vi "多点监测上位机.vi"() -> ()   [LabVIEW 2017]
uses:
  <vilib>/Utility/miscctls.llb/LVRowAndColumnTypeDef.ctl
  <vilib>/Utility/miscctls.llb/LVRowAndColumnUnsignedTypeDef.ctl
  <vilib>/Platform/TimedLoop/XDataNode/timing_clust.ctl
  <vilib>/Platform/TimedLoop/XDataNode/nitl_modes.ctl
  <vilib>/Platform/TimedLoop/XDataNode/wakeup.ctl
  <vilib>/event_ctls.llb/eventvkey.ctl
  <vilib>/Utility/xml.llb/Read From XML File(string).vi
  <vilib>/sound2/lvsound2.llb/Sound File Info (path).vi
  <vilib>/sound2/lvsound2.llb/Sound File Read Open.vi
  <vilib>/sound2/lvsound2.llb/Sound File Read (DBL).vi
  <vilib>/Instr/_visa.llb/VISA Configure Serial Port (Instr).vi
  <vilib>/Utility/inputDevices.llb/closeMouse.vi
  <vilib>/Utility/xml.llb/Write to XML File(string).vi
  <vilib>/Utility/inputDevices.llb/mouseAcquire.vi
  <vilib>/Platform/TimedLoop/XDataNode/XDataNode.xnode
  <vilib>/Platform/TimedLoop/XDataNode/XDNodeRunTimeDep.lvlib
  <vilib>/addons/database/NI_Database_API.lvlib
panel:
  out "标志-首次累积报警":bool=TRUE
  out "信号-保存配置":bool=TRUE
  out "手动静音窗口VI-引用":refnum<vi>
  in  "报警方式":T1(array[cluster])
  in  "轮询间隔 ms":dbl
  in  "一周期间隔":timestamp
  in  "周期":i64
  in  "有掉线？":bool
  out "事件-累积剂量":refnum<user-event>
  in  "报警状态":enum16{"正常", "一级报警", "二级报警", "累积报警"}[](array[ring])
  in  "累积剂量":T2(array[cluster])
  out "监测数量限值":cluster{"min":i32, "max":i32}
  out "监-停止信号":refnum<vi>
  in  "报警列表提示":string[](array[string])=["选行技巧：按住 ctl 可离散选择，按住 shift 可范围选择，ctl+A 选择全部行", "右键菜单：多选后 某些项可批量操作", "双击“单元格”：打开报警记录数据分析界面，可编辑结论、生成Word报表", "底端“状态栏”：可调整状态栏高度、分类筛选、清除状态"]
  in  "设备列表提示":string[](array[string])=["选行技巧：按住 ctl 可离散选择，按住 shift 可范围选择，ctl+A 选择全部行", "右键菜单：多选后 某些项可批量操作", "双击“状态”列：启用或禁用设备（某些版本中禁用此功能）", "双击“设备信息”列：修改设备信息", "双击“一级限值”列：修改报警限值", "双击“网络地址”列：删除设备", "双击“空白行”：添加设备"]
  in  "停止信号":enum16{"内部停止信号", "外部停止信号"}(ring)=enum."外部停止信号"
  out "事件-探头重连":refnum<user-event>
  out "报警记录数":i32
  out "通知窗口VI-引用":refnum<vi>
  in  "新记录簇":cluster{"新记录列表行":string[], "对应缓存文件":string}[](array[cluster])
  in  "报警状态":enum16{"正常", "一级报警", "二级报警", "累积报警"}(ring)
  out "蜂鸣音效":waveform(dbl)[](array[waveform]) caption="数据"
  in  "Right":i16
  in  "Left":i16
  out "间隔":u32
  in  "计时":u32
  out "引用-更新数据信号":refnum<vi>
  out "引用-更新数据簇":refnum<vi>
  in  "信号-设置":bool
  in  "菜单项-报警列表":enum16{"刷新", "预览并生成报表", "删除记录", "复制选中项至剪贴板"}(ring)=enum."预览并生成报表"
  in  "菜单项-实时列表":T3(ring)=enum."禁用"
  out "监测窗口VI":refnum<vi>
  out "报警记录缓存数据文件":string[](array[string])
  in  "缓存值":cluster{"X":timestamp[], "Y":dbl[]}[](array[cluster])
  in  "状态栏-项名[]":string[](array[string])
  in  "状态与编辑":bool
  in  "监测模式":bool caption="方格样式"
  in  "查看报表":bool caption="方格样式"
  in  "设置":bool
  in  "帮助":bool
  out "公司LOGO与型号":bool
  out "设备列表标题":enum16{"设备管理列表"}(ring)
  out "当前端口":string
  out "当前波特率":string
  out "设备列表操作提示":string
  in  "限值":T4(array[cluster])
  in  "实时数据列表":i32[](listbox)
  out "报警列表标题":enum16{"报警记录列表"}(ring)
  out "报警列表操作提示":string
  in  "T:G,F:B":bool
  in  "回复背景色锁":bool
  in  "等待时间（毫秒）":u32=10
  in  "暂停发送":bool=TRUE
  in  "报警记录列表":i32[](listbox)
  in  "状态类型":enum16{"全部", "报警", "通信", "设置"}(ring)
  in  "报警方式变了？":bool
  in  "限值变了？":bool
  in  "状态栏":i32(listbox)=-1
  out "事件-探头掉线":refnum<user-event>
  out "事件-报警缓存":refnum<user-event>
  out "测量值":cluster{"X":timestamp, "Y":dbl}[](array[cluster])
  in  "开机启动":bool
  in  "device ID":refnum<k1> caption="设备ID"
  in  "变了？":bool
  in  "发送次数":u8[](array[numeric])
  in  "异常保存记录？":bool[](array[boolean])
  in  "报警记录标志？":bool[](array[boolean])
  in  "更新列表？":bool
  in  "确认设置":bool
  out "编辑前项名":string[][](array[string])
  out "点到行列-实时列表":T5 caption="单元格位置"
  in  "探头地址":i32[](array[numeric])
  in  "探头信息":string[](array[string])
  out "点到行列-报警记录":T5 caption="单元格位置"
  in  "探头启用状态？":bool[](array[boolean])
  out "停止":bool=TRUE
  in  "清除状态":bool
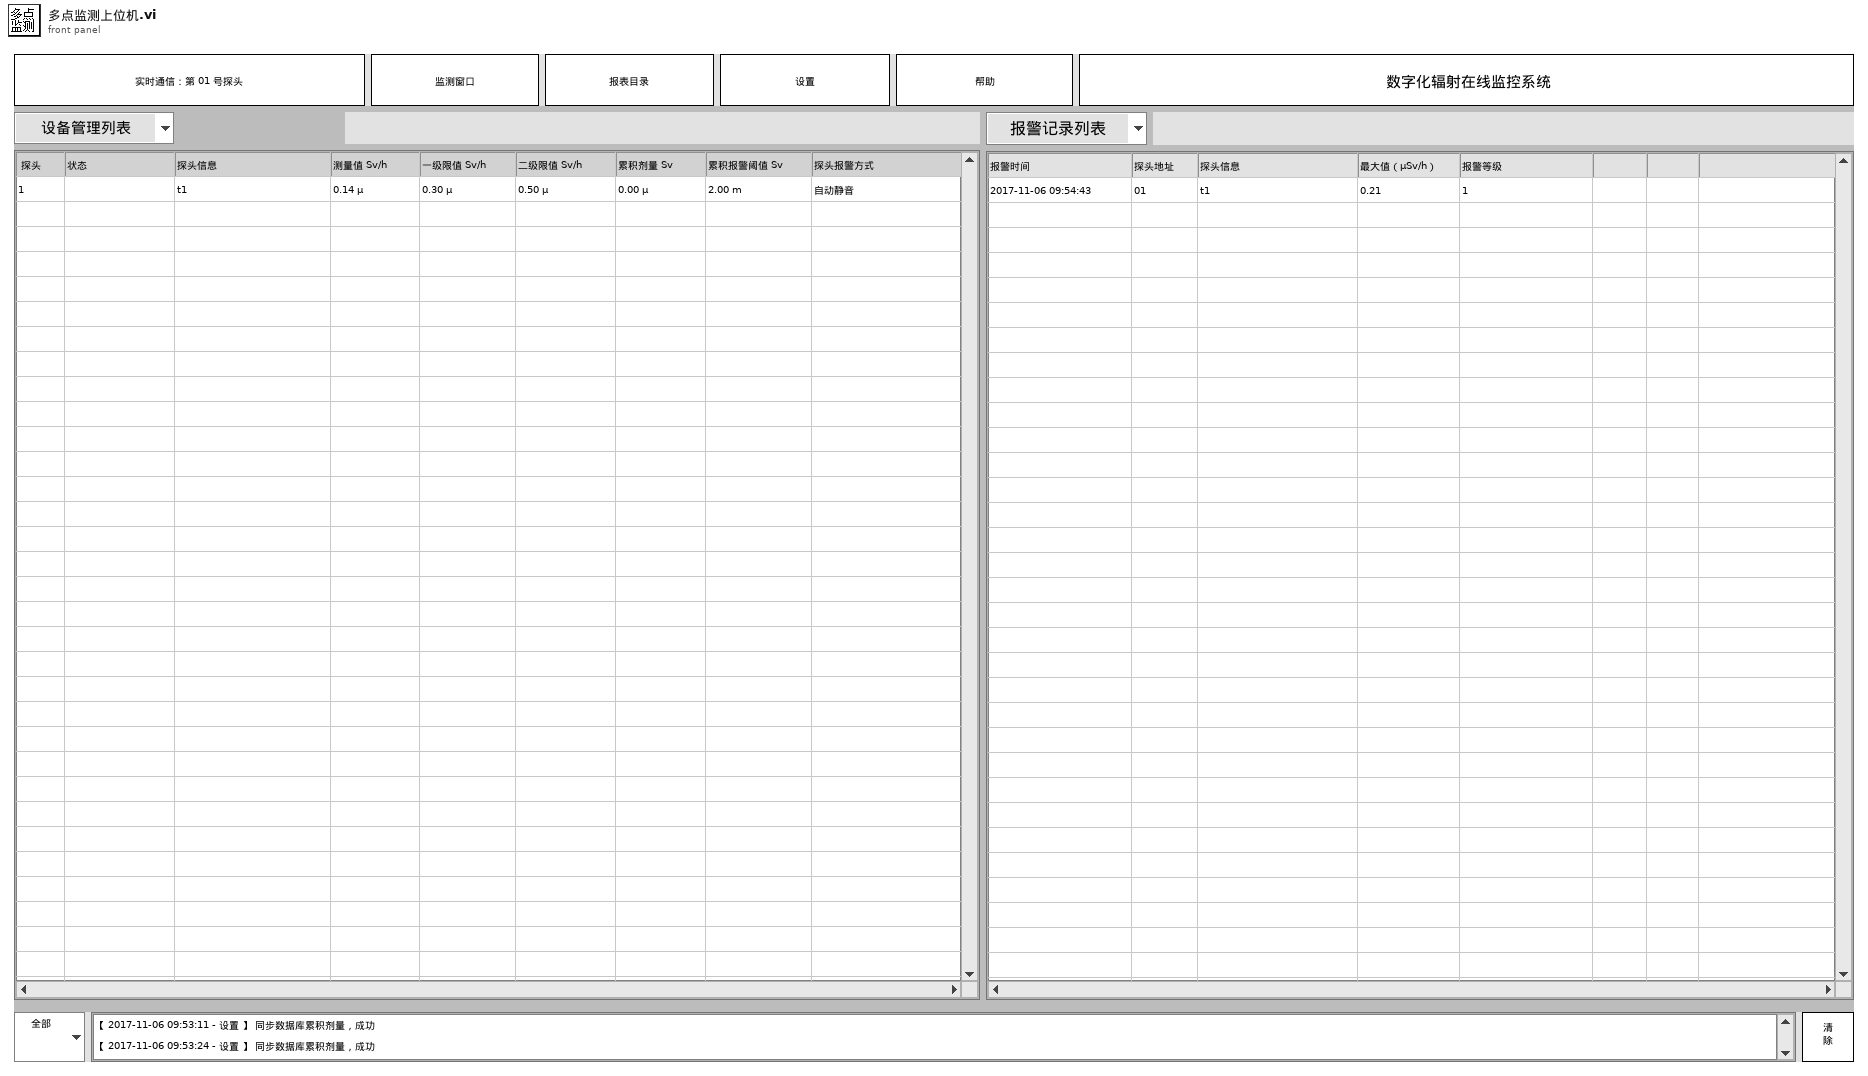
[diagram p1: front panel]
types:
  T1 = cluster{"报警方式":enum16{"常报警", "自动静音", "手动静音"}, "延迟计时":u16, "报警中？":bool}[]
  T2 = cluster{"设备名称":string, "启用累积？":bool, "起始时间":timestamp, "累积剂量":dbl, "累积报警阈值":dbl}[]
  T3 = enum16{"启用", "禁用", "修改探头信息", "修改报警限值", "交换探头地址", "备注信息", "启用累积", "禁用累积", "累积清零", "累积报警阈值", "探头报警方式"}
  T4 = cluster{"限值1":dbl, "限值2":dbl, "探头限值":enum16{"一级限值", "二级限值"}}[]
  T5 = typedef "LVRowAndColumnTypeDef.ctl" = cluster{"Row":i32, "Column":i32}
  T6 = typedef "LVRowAndColumnUnsignedTypeDef.ctl" = cluster{"Row":u32, "Column":u32}
  T7 = enum32{"Invalid", "Standard", "Closed", "Hidden", "Minimized", "Maximized"}
  T8 = enum8{"Enabled", "Disabled", "Disabled and Grayed Out"}
  T9 = enum16{"初始化", "扫描探头", "发送命令", "接收数据", "暂停发送", "结束程序", "退出"}
  T10 = typedef "XDNodeRunTimeDep.lvlib/timing_clust.ctl" = cluster{"Expected End [f-1]":u64, "Actual End [f-1]":u64, "Finished Late? [f-1]":bool, "Expected End [i-1]":u64, "Actual End [i-1]":u64, "Finished Late? [i-1]":bool, "Expected Start [i]":u64, "Actual Start [i]":u64, "Expected Start [f]":u64, "Actual Start [f]":u64, "Source Name":string, "Structure Name":string, "Period":i64, "Deadline":i64, "Offset":i64, "Start":i64, "Priority":i32, "Timeout":i32, "Mode":T11, "Wakeup Reason":T12, "Error":errorcluster, "Source Type":string, "Secondary Source Type":string, "Global End Time":u64, "Global Start Time":u64, "Frame Duration":u64, "Iteration Duration":u64, "Assigned CPU":i32, "I/O Scan Engine Mode":u32}
  T11 = typedef "XDNodeRunTimeDep.lvlib/nitl_modes.ctl" = enum32{"No Change", "Process missed periods, maintain original phase", "Discard missed periods, maintain original phase", "Process missed periods, ignore original phase", "Discard missed periods, ignore original phase"}
  T12 = typedef "XDNodeRunTimeDep.lvlib/wakeup.ctl" = enum32{"Normal", "Aborted", "Asynchronous wakeup", "Timing source error", "Timed loop error", "Timeout"}
  T13 = cluster{"探头启用状态？":bool[], "测量值":cluster{"X":timestamp, "Y":dbl}[], "限值":cluster{"限值1":dbl, "限值2":dbl, "探头限值":enum16{"一级限值", "二级限值"}}[], "报警状态":enum16{"正常", "一级报警", "二级报警", "累积报警"}[], "探头信息":string[], "累积剂量":cluster{"设备名称":string, "启用累积？":bool, "起始时间":timestamp, "累积剂量":dbl, "累积报警阈值":dbl}[]}
  T14 = cluster{"记录时间":string, "起始时间":string, "累积剂量":dbl, "报警":bool, "记录名称":string}
  T15 = cluster{"限值1":dbl, "限值2":dbl, "探头限值":enum16{"一级限值", "二级限值"}}
  T16 = enum16{"启用", "禁用", "修改探头信息", "修改报警限值", "交换探头地址", "微调测量值", "探头排序", "备注信息"}
  T17 = enum16{"启用", "禁用", "修改探头信息", "修改报警限值", "交换探头地址", "备注信息"}
  T18 = enum16{"启用", "禁用", "修改探头信息", "修改报警限值", "交换探头地址", "备注信息", "启用累积", "禁用累积", "累积清零", "累积报警阈值"}
  T19 = cluster{"实时数据列表":refnum<vi>, "缓存值":refnum<vi>, "发送次数":refnum<vi>, "限值":refnum<vi>, "异常保存记录？":refnum<vi>, "报警记录标志？":refnum<vi>, "探头启用状态？":refnum<vi>, "探头信息":refnum<vi>, "报警状态":refnum<vi>}
  T20 = cluster{"设备名称":string, "启用累积？":bool, "起始时间":timestamp, "累积剂量":dbl, "累积报警阈值":dbl}
  T21 = cluster{"企业编号":string, "员工编号":string, "通道号":string, "密码":string, "联系人数组":cluster{"姓名":string, "手机号":string}[]}
  T22 = cluster{"探头索引":i32, "缓存值":cluster{"X":timestamp[], "Y":dbl[]}}
  T23 = typedef "LVRectTypeDef.ctl" = cluster{"Left":i16, "Top":i16, "Right":i16, "Bottom":i16}
  T24 = typedef "Sound File Refnum.ctl" = refnum<file>
  T25 = cluster{"COM":refnum<visa-resource-name>, "探头地址":i32[], "探头启用状态？":bool[], "开机启动？":bool, "探头信息":string[], "限值":cluster{"限值1":dbl, "限值2":dbl, "探头限值":enum16{"一级限值", "二级限值"}}[], "最大探头数":i32, "波特率":enum16{"9600", "19200"}, "周期":i64, "报警方式":cluster{"报警方式":enum16{"常报警", "自动静音", "手动静音"}, "延迟计时":u16, "报警中？":bool}[], "静音延迟":u16}
  T26 = cluster{"COM":refnum<visa-resource-name>, "探头地址":i32[], "探头启用状态？":bool[], "开机启动？":bool, "探头信息":string[], "限值":cluster{"限值1":dbl, "限值2":dbl, "探头限值":enum16{"一级限值", "二级限值"}}[], "最大探头数":i32, "波特率":enum16{"9600", "19200"}, "周期":i64, "初始化的数组":cluster{"报警方式":enum16{"常报警", "自动静音", "手动静音"}, "延迟计时":u16, "报警中？":bool}[], "静音延迟":u16}
  T27 = cluster{"报警方式":enum16{"常报警", "自动静音", "手动静音"}, "延迟计时":u16, "报警中？":bool}
  T28 = cluster{"维数大小":i32, "缓存值":cluster{"X":timestamp[], "Y":dbl[]}}
  T29 = cluster{"seconds since 1Jan1904":timestamp, "测量值":dbl}
  T30 = typedef "NI_Database_API.lvlib/Conn ObjectReference.ctl" = refnum<k1>
  T31 = typedef "LVPoint32TypeDef.ctl" = cluster{"Horizontal":i32, "Vertical":i32}
  T32 = cluster{"button 1":bool, "button 2":bool, "button 3":bool, "button 4":bool}
  T33 = cluster{"Shift":bool, "Ctrl":bool, "Alt":bool, "Cmd":bool, "Opt":bool}
  T34 = typedef "eventvkey.ctl" = enum16{"ASCII", "Enter", "Return", "Shift", "Ctrl", "Alt", "Cmd", "Opt", "Caps", "NumLock", "Clear", "Break", "Up", "Down", "Left", "Right", "Insert", "Delete", "Home", "End", "PageUp", "PageDown", "Escape", "Help", "Pause", "ScrollLock", "F1", "F2", "F3", "F4", "F5", "F6", "F7", "F8", "F9", "F10", "F11", "F12", "F13", "F14", "F15", "F16", "F17", "F18", "F19", "F20", "F21", "F22", "F23", "F24", "Play", "VolumeUp", "VolumeDown", "Mute", "Two Byte Char"}
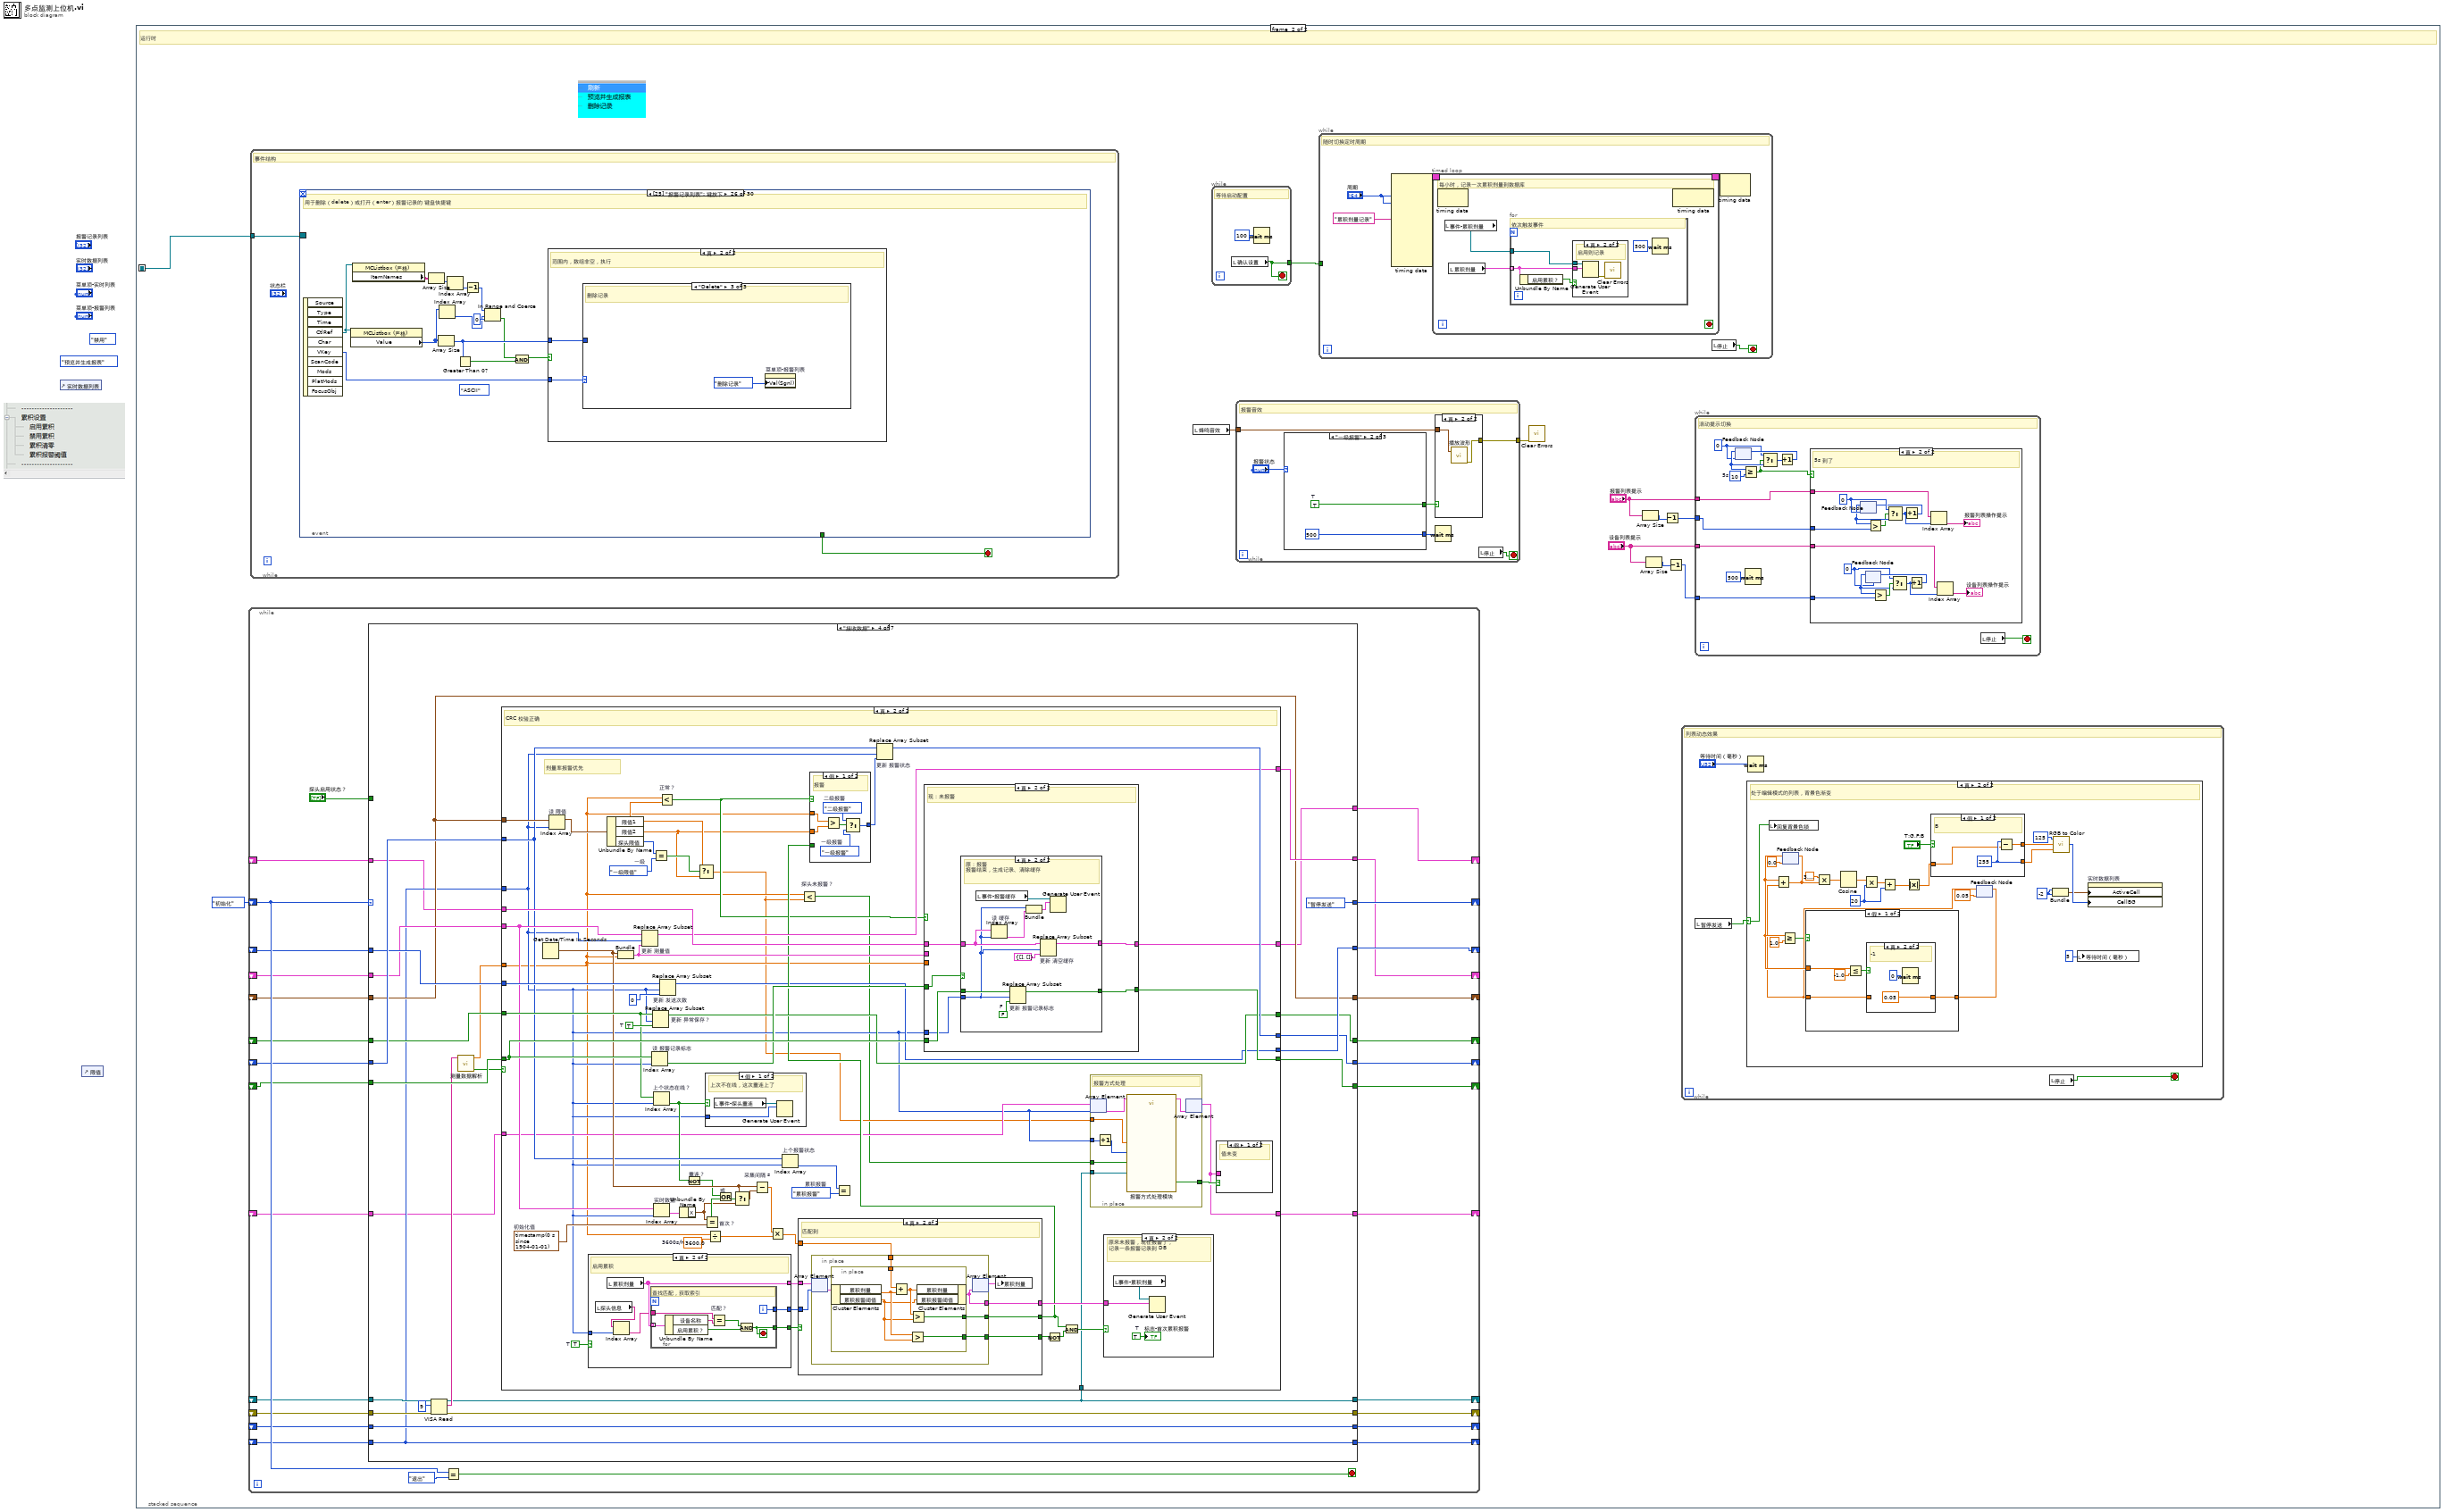
[diagram p0: block diagram]
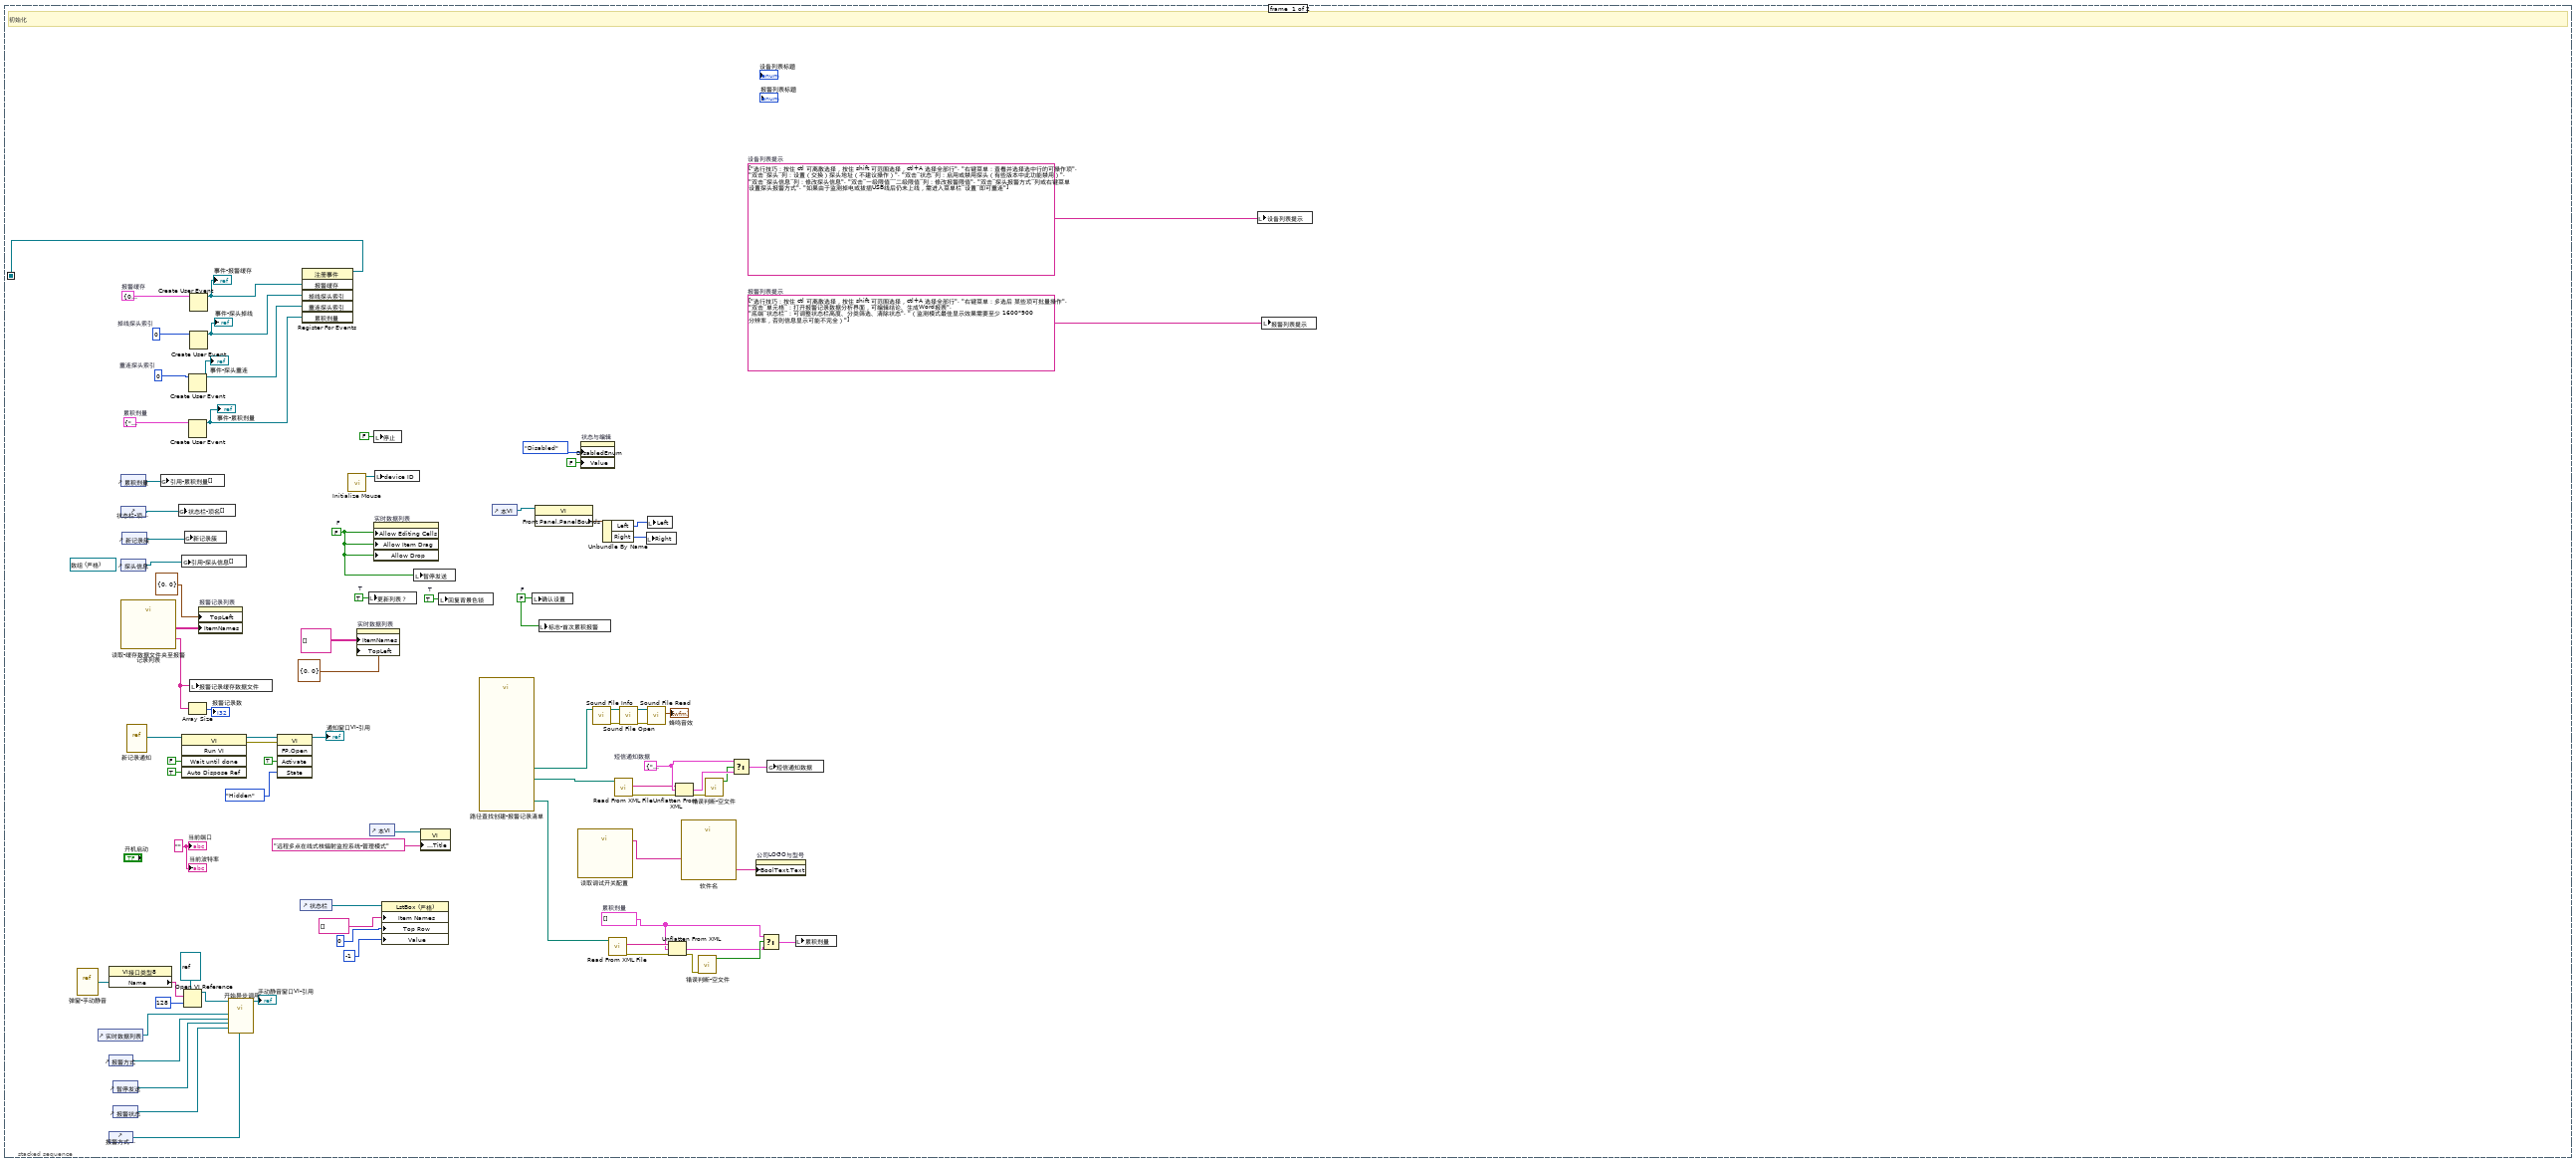
[diagram p2: hidden frame]
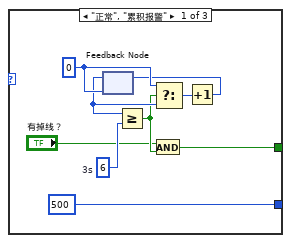
[diagram p6: hidden frame]
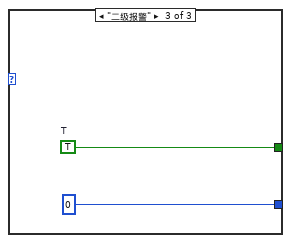
[diagram p7: hidden frame]
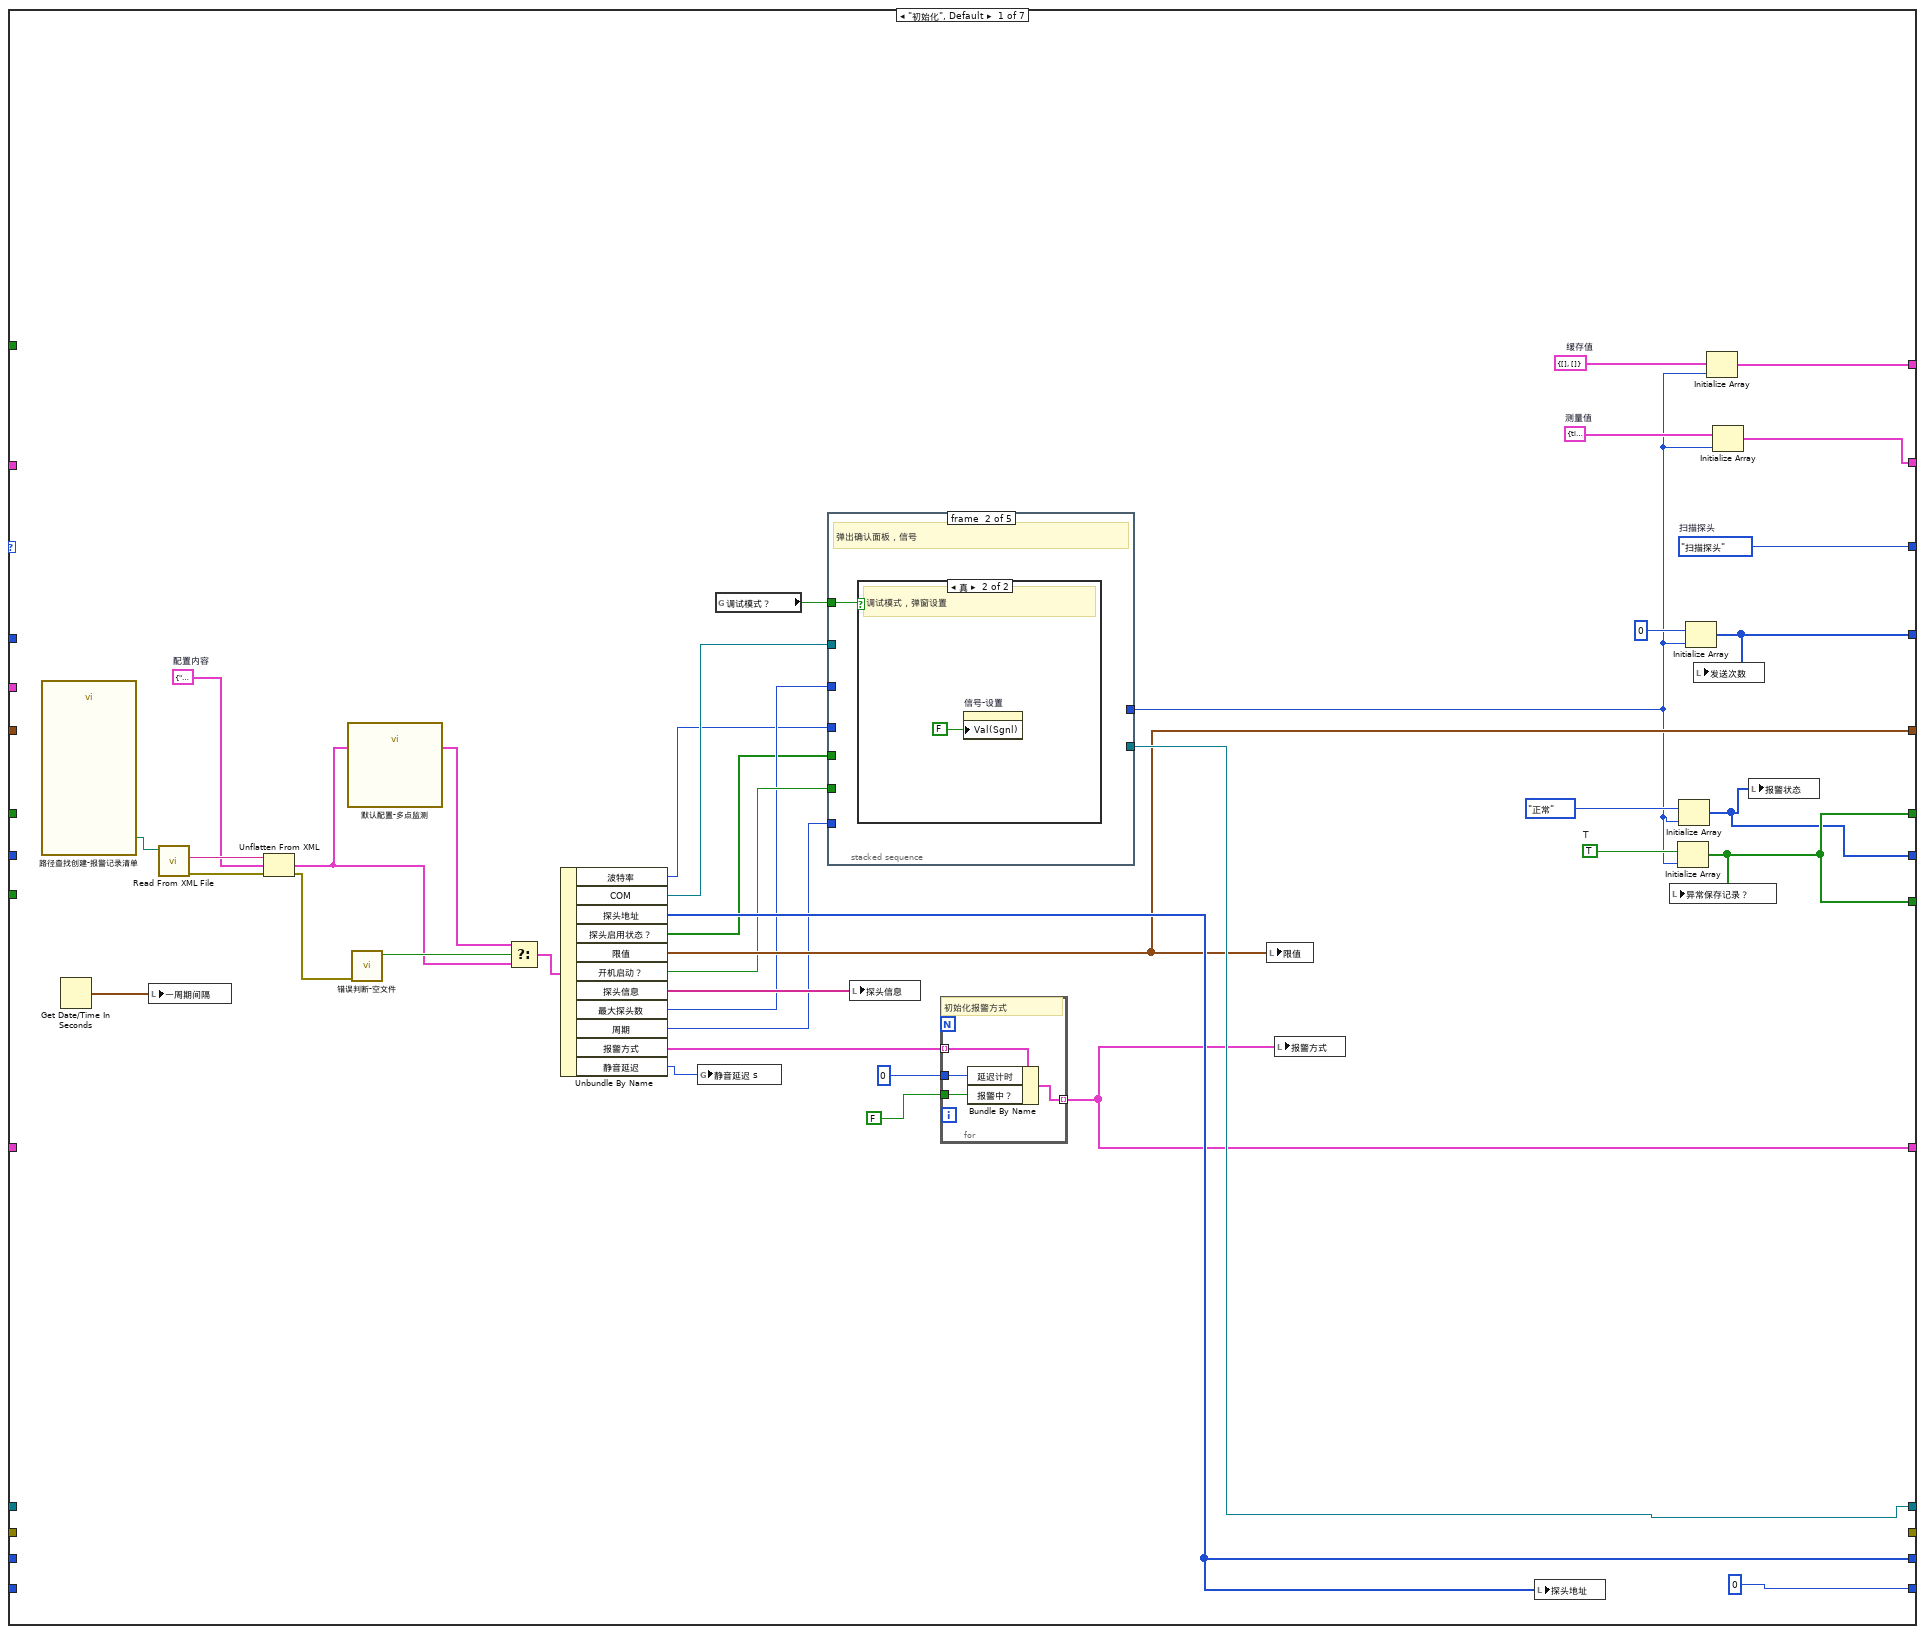
[diagram p8: hidden frame]
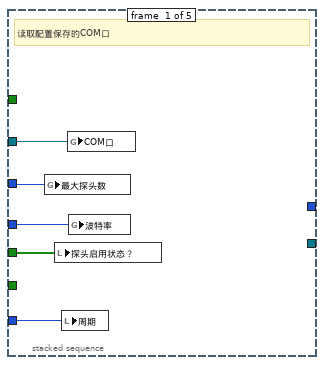
[diagram p9: hidden frame]
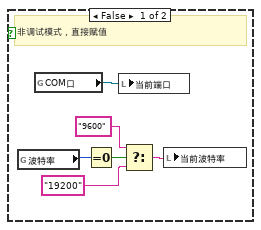
[diagram p10: hidden frame]
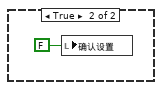
[diagram p12: hidden frame]
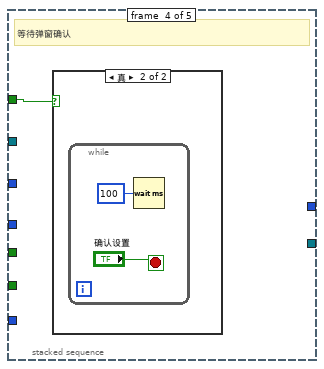
[diagram p13: hidden frame]
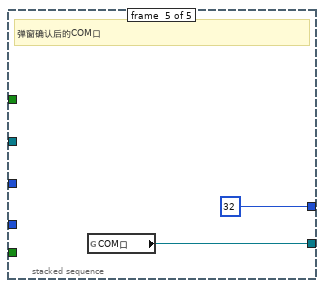
[diagram p15: hidden frame]
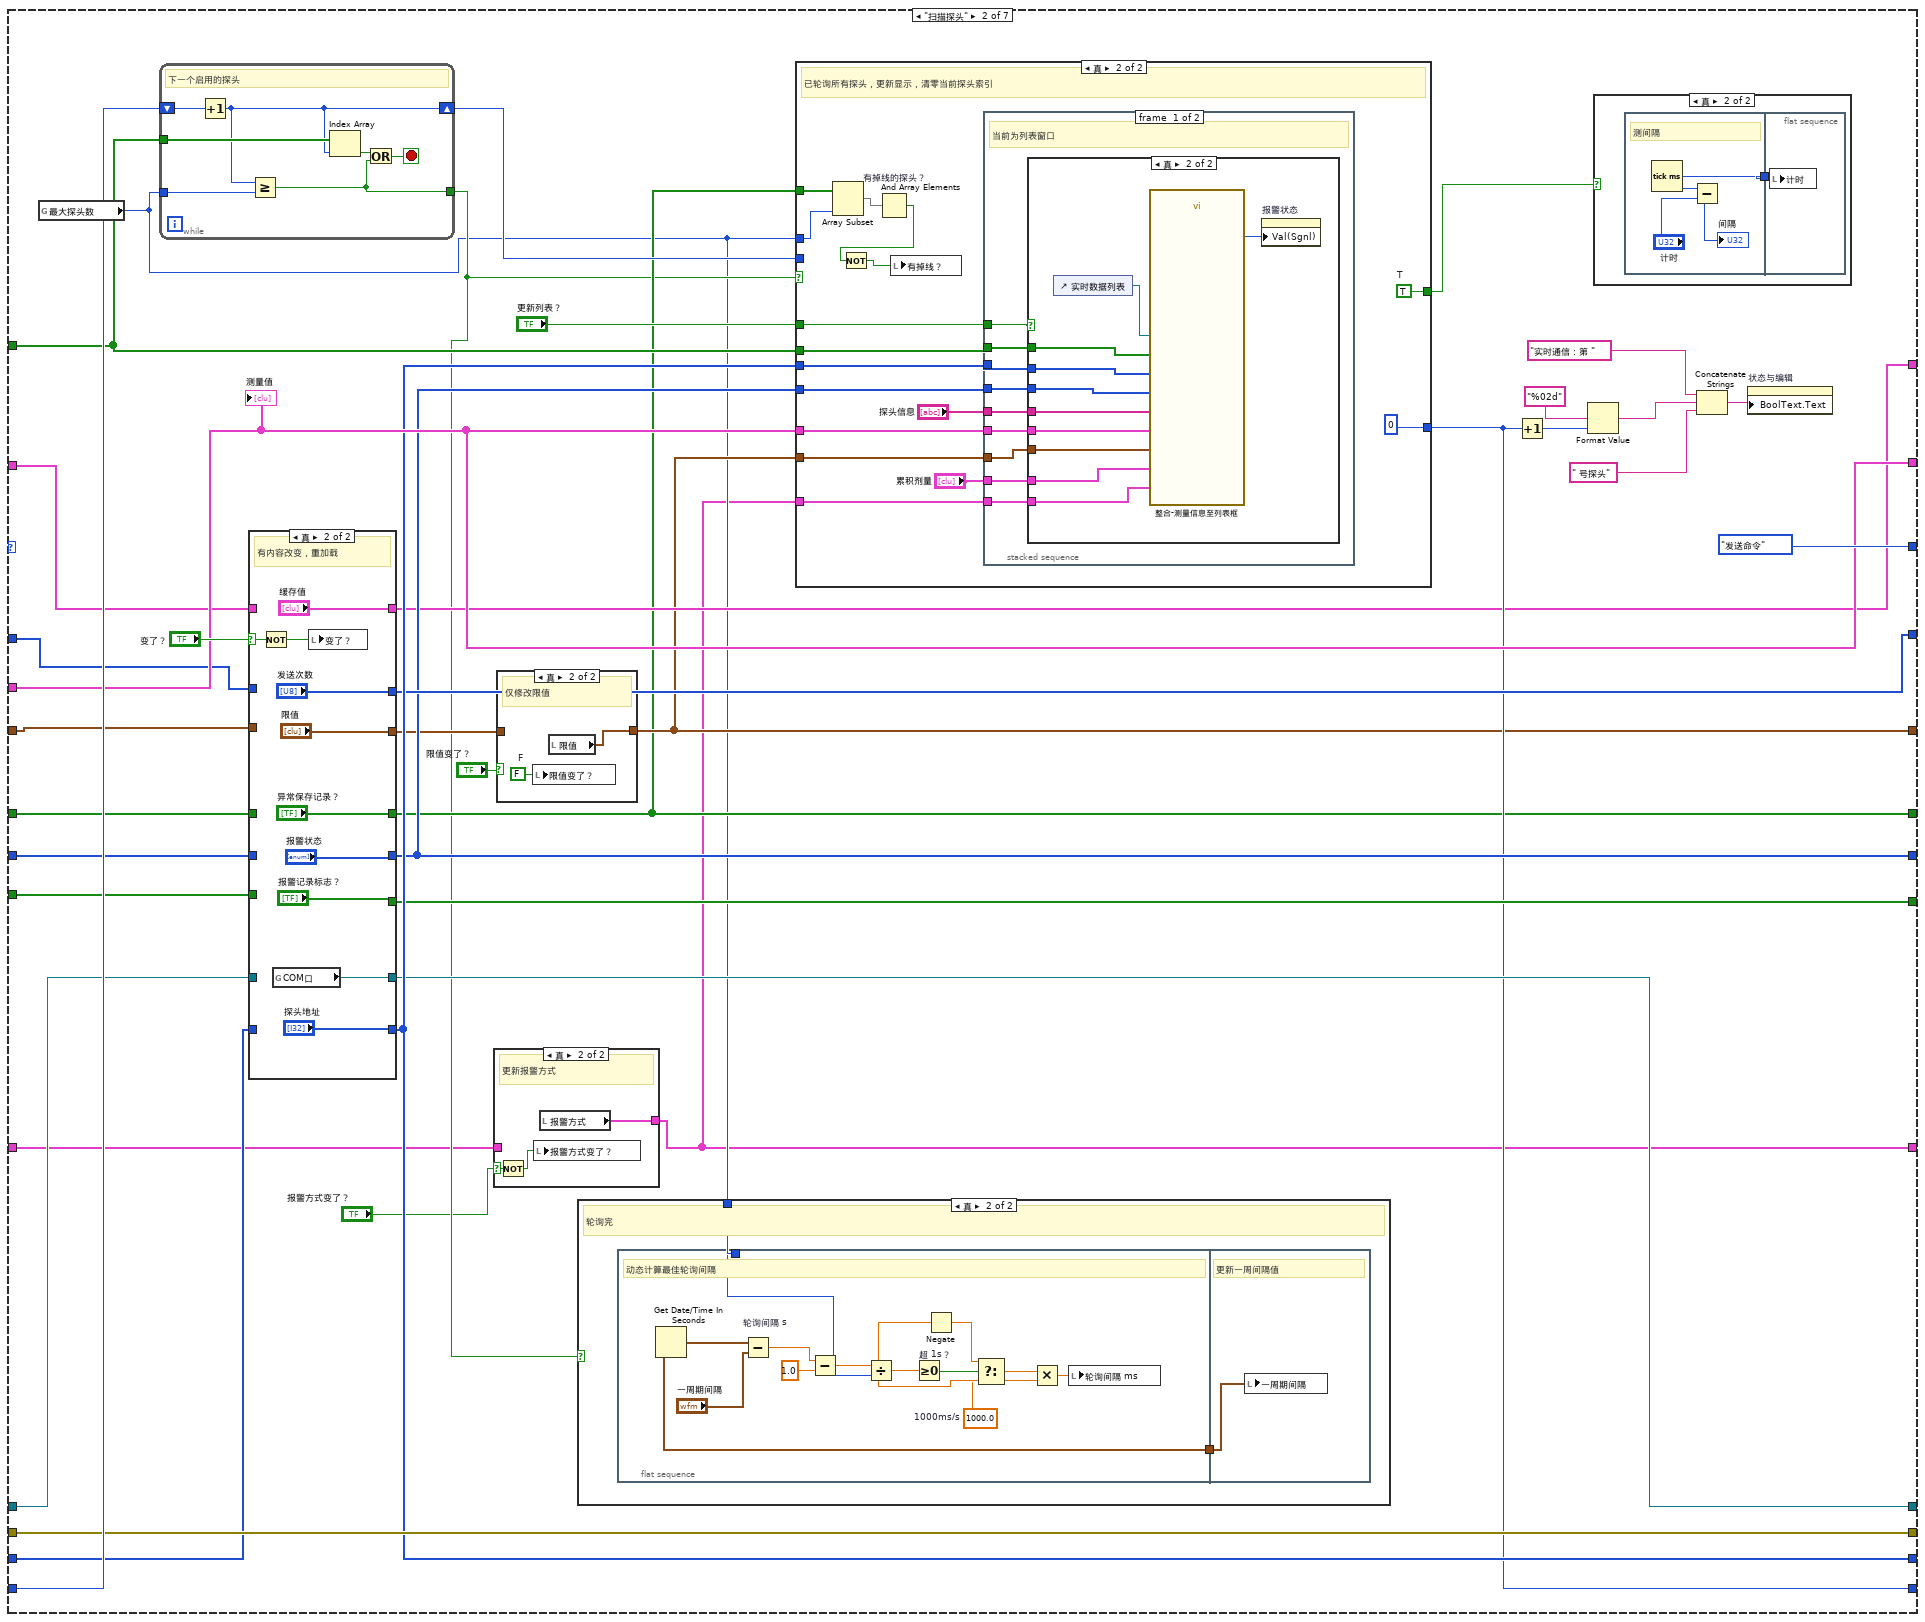
[diagram p16: hidden frame]
diagram:
  (unwired) T3."禁用" ("菜单项-实时列表")
  (unwired) enum16{"刷新", "预览并生成报表", "删除记录", "复制选中项至剪贴板"}."预览并生成报表" ("菜单项-报警列表")
  n1 = control-ref of="实时数据列表"() -> ()  [unwired: 1 out]
  n2 = control-ref of="限值"() -> ()  [unwired: 1 out]
  n3 = stacked-sequence {
    seq-local: [w80 _] -> [_ w93]
    frame #0 {
      w2 = FALSE  # F
      (unwired) refnum<vi> refnum ("探头信息")
      w20 = T20 {"设备名称"="", "启用累积？"=FALSE, "起始时间"=timestamp(0 s since 1904-01-01), "累积剂量"=0.0, "累积报警阈值"=0.0}  # 累积剂量
      w23 = T2 []  # 累积剂量
      w31 = "" ("当前端口")
      w35 = string[] ["选行技巧：按住 ctl 可离散选择，按住 shift 可范围选择，ctl+A 选择全部行", "右键菜单：多选后 某些项可批量操作", "双击“单元格”：打开报警记录数据分析界面，可编辑结论、生成Word报表", "底端“状态栏”：可调整状态栏高度、分类筛选、清除状态", "（监测模式最佳显示效果需要至少 1600*900 分辨率，否则信息显示可能不完全）"]  # 报警列表提示
      w36 = string[] ["选行技巧：按住 ctl 可离散选择，按住 shift 可范围选择，ctl+A 选择全部行", "右键菜单：查看并选择选中行的可操作项", "双击“探头”列：设置（交换）探头地址（不建议操作）", "双击“状态”列：启用或禁用探头（有些版本中此功能禁用）", "双击“探头信息”列：修改探头信息", "双击“一级限值”“二级限值”列：修改报警限值", "双击“探头报警方式”列或右键菜单 设置探头报警方式", "如果由于监测掉电或拔插USB线后仍未上线，需进入菜单栏“设置”即可重连"]  # 设备列表提示
      w42 = T21 {"企业编号"="", "员工编号"="", "通道号"="", "密码"="", "联系人数组"=[]}  # 短信通知数据
      w46 = u32 0  # 重连探头索引
      w70 = TRUE  # T
      w76 = TRUE  # T
      w75 = FALSE  # F
      w79 = u32 0  # 掉线探头索引
      w82 = T22 {"探头索引"=0, "缓存值"={"X"=[], "Y"=[]}}  # 报警缓存
      # "初始化"
      n4 = vi-ref "弹窗-手动静音.vi"() -> (w7:refnum<vi>)
      n5 = control-ref of="实时数据列表"() -> (w13:refnum<vi>)
      n6 = property class="VI接口类型8"(reference=w7) -> ("Name"=w6:string)  [unwired: 1 in, 2 out]
      n7 = control-ref of="报警方式"() -> (w12:refnum<vi>)
      n8 = control-ref of="报警方式变了？"() -> (w9:refnum<vi>)
      n9 = control-ref of="暂停发送"() -> (w11:refnum<vi>)
      n10 = control-ref of="报警状态"() -> (w10:refnum<vi>)
      n11 = control-ref of="累积剂量"() -> (w25:refnum<vi>)
      n12 = control-ref of="状态栏-项名[]"() -> (w78:refnum<vi>)
      n13 = control-ref of="探头信息"() -> (w18:refnum<vi>)
      n14 = call "读取-缓存数据文件夹至报警记录列表.vi"() -> ("文件名"=w48:string[], "报警记录列表"=w69:string[][])  [unwired: 8 in, 2 out]
      n15 = control-ref of="新记录簇"() -> (w58:refnum<vi>)
      n16 = vi-ref "新记录通知.vi"() -> (w57:refnum<vi>)
      n17 = global write "全局变量-35点监测.vi" "引用-累积剂量[]"(w25) -> ()
      n18 = global write "全局变量-35点监测.vi" "状态栏-项名[]"(w78) -> ()
      n19 = invoke class="VI" method="Run VI"(reference=w57, "Wait until done"=FALSE ("结束前等待"), "Auto Dispose Ref"=TRUE ("自动销毁引用")) -> (reference out=w54:refnum<vi>, error out=w34:errorcluster)  [unwired: 2 in, 3 out]
      n20 = global write "全局变量-35点监测.vi" "引用-探头信息[]"(w18) -> ()
      n21 = Open VI Reference(type specifier VI Refnum (for type only)=refnum<vi> refnum ("类型说明符VI引用句柄（仅用于类型）"), vi path=w6, options=128 ("选项")) -> (vi reference=w3:refnum<vi>)  [unwired: 3 in, 1 out]
      n22 = global write "全局变量-35点监测.vi" "新记录簇"(w58) -> ()
      n23 = Create User Event(user event datatype=w46) -> (user event=w45:refnum<user-event>)  [unwired: 1 in, 1 out]
      "事件-探头重连" <- w45
      n24 = Create User Event(user event datatype=w20) -> (user event=w19:refnum<user-event>)  [unwired: 1 in, 1 out]
      "事件-累积剂量" <- w19
      n25 = Array Size(array=w48) -> (size(s)=→"报警记录数":i32)
      n26 = Create User Event(user event datatype=w82) -> (user event=w81:refnum<user-event>)  [unwired: 1 in, 1 out]
      "事件-报警缓存" <- w81
      n27 = Create User Event(user event datatype=w79) -> (user event=w74:refnum<user-event>)  [unwired: 1 in, 1 out]
      "事件-探头掉线" <- w74
      n28 = local write "报警记录缓存数据文件"(w48) -> ()
      n29 = property on="报警记录列表" class="MCListbox (严格)"("TopLeft"=T6 {"Row"=0, "Column"=0} ("左上可见单元格"), "ItemNames"=w69) -> ()  [unwired: 2 in, 2 out]
      n30 = call-by-ref "开始异步调用"(reference=w3, "引用-报警方式值改变？"=w9, "引用-报警状态"=w10, "引用-暂停发送"=w11, "引用-报警方式"=w12, "引用-实时数据列表"=w13) -> (reference out=→"手动静音窗口VI-引用":refnum<vi>)  [unwired: 8 in, 1 out]
      n31 = invoke class="VI" method="FP.Open"(reference=w54, error in=w34, "Activate"=TRUE ("激活？"), "State"=T7."Hidden" ("状态")) -> (reference out=→"通知窗口VI-引用":refnum<vi>)  [unwired: 1 in, 4 out]
      n32 = control-ref of="状态栏"() -> (w16:refnum<vi>)
      n33 = register-events(w81, w74, w45, w19) -> (reference out=w80:refnum<event-registration>)  [unwired: 2 in, 1 out]
      n34 = call <vilib>:"Initialize Mouse.vi"() -> ("device ID"=w77:refnum<k1>)  [unwired: 10 in, 1 out]
      n35 = property on="实时数据列表" class="MCListbox (严格)"("ItemNames"=string[][] [] ("项名"), "TopLeft"=T6 {"Row"=0, "Column"=0} ("左上可见单元格")) -> ()  [unwired: 2 in, 2 out]
      n36 = local write "更新列表？"(w76) -> ()
      n37 = control-ref of="本VI"() -> (w50:refnum<vi>)
      n38 = local write "停止"(FALSE ("停止")) -> ()
      n39 = property on="实时数据列表" class="多列列表框 (严格)"("Allow Editing Cells"=w75, "Allow Item Drag"=w75, "Allow Drop"=w75) -> ()  [unwired: 2 in, 2 out]
      n40 = local write "device ID"(w77) -> ()
      n41 = property class="LstBox (严格)"(reference=w16, "Item Names"=string[] [] ("项名"), "Top Row"=0 ("顶行"), "Value"=-1 ("顶行")) -> ()  [unwired: 1 in, 2 out]
      n42 = local write "暂停发送"(w75) -> ()
      n43 = property class="VI"(reference=w50, "Front Panel.Title"="远程多点在线式核辐射监控系统-管理模式" ("前面板窗口:标题")) -> ()  [unwired: 1 in, 2 out]
      n44 = local write "回复背景色锁"(w70) -> ()
      n45 = call "路径查找创建-报警记录清单.vi"() -> ("短信通知配置文件"=w37:path, "蜂鸣音效文件路径"=w60:path, "累积剂量配置文件"=w17:path)  [unwired: 8 in, 9 out]
      n46 = control-ref of="本VI"() -> (w67:refnum<vi>)
      n47 = local write "确认设置"(w2) -> ()
      n48 = property class="VI"(reference=w67) -> ("Front Panel.PanelBounds"=w68:T23)  [unwired: 1 in, 2 out]
      n49 = local write "标志-首次累积报警"(w2) -> ()
      n50 = call "读取调试开关配置.vi"() -> ("软件版本"=w30:string)  [unwired: 9 in, 2 out]
      n51 = property on="状态与编辑" class="Bool (严格)"("DisabledEnum"=T8."Disabled" ("禁用"), "Value"=FALSE ("状态与编辑")) -> ()  [unwired: 2 in, 2 out]
      n52 = call-poly <vilib>:"Sound File Info.vi"("path"=w60) -> ("error out"=w63:errorcluster, "path out"=w62:path)  [unwired: 7 in, 2 out]
      n53 = Unbundle By Name(w68) -> ("Left"=w66:i16, "Right"=w65:i16)
      n54 = call-poly <vilib>:"Read From XML File.vi"("XML File Path"=w17) -> ("error out"=w28:errorcluster, "XML Elements"=w26:string)  [unwired: 8 in, 1 out]
      n55 = call-poly <vilib>:"Read From XML File.vi"("XML File Path"=w37) -> ("error out"=w38:errorcluster, "XML Elements"=w40:string)  [unwired: 8 in, 1 out]
      n56 = call-poly <vilib>:"Sound File Open.vi"("error in (no error)"=w63, "path"=w62) -> ("error out"=w64:errorcluster, "sound file refnum"=w61:T24)  [unwired: 8 in]
      n57 = local write "Right"(w65) -> ()
      n58 = local write "Left"(w66) -> ()
      n59 = call-poly <vilib>:"Sound File Read.vi"("error in (no error)"=w64, "sound file refnum"=w61) -> ("data"=→"蜂鸣音效":waveform(dbl)[])  [unwired: 5 in, 4 out]
      n60 = Unflatten From XML(xml string=w26, type=w23, error in (no error)=w28) -> (value=w22:T2, error out=w27:errorcluster)
      n61 = Unflatten From XML(xml string=w40, type=w42, error in (no error)=w38) -> (value=w43:T21, error out=w39:errorcluster)
      n62 = call "软件名"("软件版本"=w30) -> ("Result"=w29:string)  [unwired: 13 in, 1 out]
      n63 = call "错误判断-空文件.vi"("错误输入"=w27) -> ("空文件？"=w24:bool)  [unwired: 9 in, 1 out]
      n64 = call "错误判断-空文件.vi"("错误输入"=w39) -> ("空文件？"=w41:bool)  [unwired: 9 in, 1 out]
      n65 = Select(t=w42, s=w41, f=w43) -> (s? t:f=w44:T21)
      n66 = property on="公司LOGO与型号" class="Bool"("BoolText.Text"=w29) -> ()  [unwired: 2 in, 2 out]
      n67 = Select(t=w23, s=w24, f=w22) -> (s? t:f=w21:T2)
      n68 = global write "全局变量-35点监测.vi" "短信通知数据"(w44) -> ()
      n69 = local write "累积剂量"(w21) -> ()
      n70 = local write "设备列表提示"(w36) -> ()
      n71 = local write "报警列表提示"(w35) -> ()
      "当前端口" <- w31
      "当前波特率" <- w31
    }
    frame #1 {
      # "运行时"
      n72 = while {
        shift-right: [w194] -> _
        shift-left: T9."初始化" -> [w195]
        shift-right: [w193] -> _
        shift-left: _ -> [w191]
        shift-right: [w192] -> _
        shift-left: _ -> [w190]
        shift-right: [w176] -> _
        shift-left: _ -> [w180]
        shift-right: [w175] -> _
        shift-left: _ -> [w182]
        shift-right: [w179] -> _
        shift-left: _ -> [w181]
        shift-right: [w187] -> _
        shift-left: _ -> [w188]
        shift-right: [w173] -> _
        shift-left: _ -> [w185]
        shift-right: [w183] -> _
        shift-left: _ -> [w184]
        shift-right: [w174] -> _
        shift-left: _ -> [w178]
        shift-right: [w177] -> _
        shift-left: _ -> [w186]
        shift-right: [w172] -> _
        shift-left: _ -> [w171]
        shift-right: [w169] -> _
        shift-left: _ -> [w168]
        stop <- w196 stop-if-true
        n73 = case shown="\"接收数据\"" w195 {
          selector: w195 -> [_ _ _ _ _ _ w758]
          tunnel: [w235 T9."发送命令" T9."接收数据" T9."暂停发送" w714 T9."退出" w758] -> w194
          tunnel: [w224 w281 w426 w486 w712 _ w757] -> w193
          tunnel: [_ w297 w437 w489 w711 _ w756] -> w192
          tunnel: w191 -> [_ w282 _ w510 w712 w742 w757]
          tunnel: w190 -> [_ w297 _ w509 w711 w744 w756]
          tunnel: w188 -> [_ w286 w432 w506 w706 w737 w753]
          tunnel: [w227 w285 w430 w501 w706 w737 w753] -> w187
          tunnel: w186 -> [_ w291 w421 w496 w701 w733 w749]
          tunnel: w185 -> [_ w298 w411 w495 w700 w732 w748]
          tunnel: w184 -> [_ w287 w429 w505 w704 w736 w750]
          tunnel: [w226 w265 w428 w500 w704 w736 w750] -> w183
          tunnel: [0 ("维数大小") w278 w411 w495 w700 w732 w748] -> w173
          tunnel: w182 -> [_ w284 w422 w507 w703 w735 w755]
          tunnel: w181 -> [_ w292 w424 w504 w707 w738 w752]
          tunnel: w180 -> [_ w293 w418 w499 w705 w725 w751]
          tunnel: [w220 w292 w423 w502 w707 w738 w752] -> w179
          tunnel: w178 -> [_ w289 w414 w503 w702 w734 w754]
          tunnel: [w223 w290 w421 w496 w701 w733 w749] -> w177
          tunnel: [w216 w270 w417 w499 w705 w725 w751] -> w176
          tunnel: [w208 w283 w422 w497 w703 w735 w755] -> w175
          tunnel: [w226 w288 w413 w498 w702 w734 w754] -> w174
          tunnel: [w219 w276 w415 w490 w699 w729 w747] -> w172
          tunnel: w171 -> [_ w275 w410 w491 w699 w729 w747]
          tunnel: "探头启用状态？" -> [_ w266 _ _ _ _ _]
          tunnel: [w200 w260 w404 w487 w688 w719 w746] -> w169
          tunnel: w168 -> [_ w261 w404 w488 w688 w719 w746]
          frame "初始化", Default {
            w199 = T25 {"COM"="", "探头地址"=[], "探头启用状态？"=[], "开机启动？"=FALSE, "探头信息"=[], "限值"=[], "最大探头数"=0, "波特率"=enum."19200", "周期"=0, "报警方式"=[], "静音延迟"=0}  # 配置内容
            w221 = cluster{"X":timestamp[], "Y":dbl[]} {"X"=[], "Y"=[]}  # 缓存值
            w222 = cluster{"X":timestamp, "Y":dbl} {"X"=timestamp(0 s since 1904-01-01), "Y"=0.0}  # 测量值
            w232 = TRUE  # T
            w235 = T9."扫描探头"  # 扫描探头
            n74 = call "路径查找创建-报警记录清单.vi"() -> ("配置文件"=w217:path)  [unwired: 8 in, 11 out]
            n75 = Get Date/Time In Seconds() -> (seconds since 1Jan1904=w206:timestamp)
            n76 = local write "一周期间隔"(w206) -> ()
            n77 = call-poly <vilib>:"Read From XML File.vi"("XML File Path"=w217) -> ("error out"=w233:errorcluster, "XML Elements"=w234:string)  [unwired: 8 in, 1 out]
            n78 = Unflatten From XML(xml string=w234, type=w199, error in (no error)=w233) -> (value=w198:T25, error out=w210:errorcluster)
            n79 = call "默认配置-多点监测.vi"("配置内容（结构）"=w198) -> ("默认配置"=w228:T26)  [unwired: 10 in]
            n80 = call "错误判断-空文件.vi"("错误输入"=w210) -> ("空文件？"=w209:bool)  [unwired: 9 in, 1 out]
            n81 = Select(t=w228, s=w209, f=w198) -> (s? t:f=w229:T25)
            n82 = Unbundle By Name(w229) -> ("波特率"=w212:enum16{"9600", "19200"}, "COM"=w225:refnum<visa-resource-name>, "探头地址"=w223:i32[], "探头启用状态？"=w211:bool[], "限值"=w216:T4, "开机启动？"=w214:bool, "探头信息"=w215:string[], "最大探头数"=w213:i32, "周期"=w207:i64, "报警方式"=w203:T1, "静音延迟"=w197:u16)
            n83 = global write "全局变量-35点监测.vi" "静音延迟 s"(w197) -> ()
            n84 = global read "全局变量-35点监测.vi" "调试模式？"() -> (w205:bool)
            n85 = stacked-sequence {
              tunnel: w225 -> [w244 _ _ _ _]
              tunnel: [_ _ _ _ w259] -> w224
              tunnel: [_ _ _ _ 32 ("最大探头数")] -> w204
              tunnel: w214 -> [_ _ _ _ _]
              tunnel: w213 -> [w243 _ _ _ _]
              tunnel: w212 -> [w242 _ _ _ _]
              tunnel: w211 -> [w241 _ _ _ _]
              tunnel: w207 -> [w240 _ _ _ _]
              tunnel: w205 -> [_ w245 w253 w255 _]
              frame #0 {
                # "读取配置保存的COM口"
                n86 = global write "全局变量-35点监测.vi" "最大探头数"(w243) -> ()
                n87 = local write "探头启用状态？"(w241) -> ()
                n88 = local write "周期"(w240) -> ()
                n89 = global write "全局变量-35点监测.vi" "COM口"(w244) -> ()
                n90 = global write "全局变量-35点监测.vi" "波特率"(w242) -> ()
              }
              frame #1 {
                # "弹出确认面板，信号"
                n91 = case shown="真" w245 {
                  frame False {
                    # "非调试模式，直接赋值"
                    n92 = global read "全局变量-35点监测.vi" "波特率"() -> (w250:enum16{"9600", "19200"})
                    n93 = global read "全局变量-35点监测.vi" "COM口"() -> (w251:refnum<visa-resource-name>)
                    n94 = Equal To 0?(x=w250) -> (x = 0?=w249:bool)
                    n95 = local write "当前端口"(w251) -> ()
                    n96 = Select(t="9600" ("当前波特率"), s=w249, f="19200" ("当前波特率")) -> (s? t:f=w246:string)
                    n97 = local write "当前波特率"(w246) -> ()
                  }
                  frame True {
                    # "调试模式，弹窗设置"
                    n98 = property on="信号-设置" class="Bool (严格)"("Val(Sgnl)"=FALSE ("允许编辑单元格")) -> ()  [unwired: 2 in, 2 out]
                  }
                }
              }
              frame #2 {
                # "等待标志置F"
                n99 = case shown="假" w253 {
                  frame False {
                  }
                  frame True {
                    n100 = local write "确认设置"(FALSE ("确认COM")) -> ()
                  }
                }
              }
              frame #3 {
                # "等待弹窗确认"
                n101 = case shown="真" w255 {
                  frame False {
                  }
                  frame True {
                    n102 = while {
                      stop <- "确认设置" stop-if-true
                      n103 = Wait (ms)(milliseconds to wait=u32 100 ("等待时间（毫秒）")) -> ()  [unwired: 1 out]
                    }
                  }
                }
              }
              frame #4 {
                # "弹窗确认后的COM口"
                n104 = global read "全局变量-35点监测.vi" "COM口"() -> (w259:refnum<visa-resource-name>)
              }
            }
            n105 = local write "探头信息"(w215) -> ()
            n106 = for {
              tunnel: w203 -> [w239] mode=indexing
              tunnel: u16 0 ("延迟计时") -> [w238]
              tunnel: FALSE ("报警中？") -> [w237]
              tunnel: [w236] -> w200 mode=indexing
              # "初始化报警方式"
              n107 = Bundle By Name(cluster=w239, "延迟计时"=w238, "报警中？"=w237) -> (w236:T27)
            }
            n108 = local write "限值"(w216) -> ()
            n109 = local write "报警方式"(w200) -> ()
            n110 = local write "探头地址"(w223) -> ()
            n111 = Initialize Array(w232, w204) -> (w226:bool[])
            n112 = local write "异常保存记录？"(w226) -> ()
            n113 = Initialize Array(enum16{"正常", "一级报警", "二级报警", "累积报警"}."正常", w204) -> (w208:enum16{"正常", "一级报警", "二级报警", "累积报警"}[])
            n114 = Initialize Array(u8 0 ("维数大小"), w204) -> (w227:u8[])
            n115 = local write "发送次数"(w227) -> ()
            n116 = Initialize Array(w221, w204) -> (w219:cluster{"X":timestamp[], "Y":dbl[]}[])
            n117 = Initialize Array(w222, w204) -> (w220:cluster{"X":timestamp, "Y":dbl}[])
            n118 = local write "报警状态"(w208) -> ()
          }
          frame "扫描探头" {
            n119 = global read "全局变量-35点监测.vi" "最大探头数"() -> (w263:i32)
            n120 = while {
              shift-right: [w398] -> w296
              shift-left: w298 -> [w403]
              tunnel: [w400] -> w264
              tunnel: w266 -> [w399]
              tunnel: w263 -> [w397]
              stop <- w401 stop-if-true
              # "下一个启用的探头"
              n121 = Increment(x=w403) -> (x+1=w398:i32)
              n122 = Greater Or Equal?(x=w398, y=w397) -> (x >= y?=w400:bool)
              n123 = Index Array(array=w399, index=w398) -> (element=w402:bool)
              n124 = Or(x=w402, y=w400) -> (x .or. y?=w401:bool)
            }
            n125 = case shown="真" "变了？" {
              selector: "变了？" -> [_ w343]
              tunnel: [w333 "限值"] -> w268
              tunnel: w293 -> [w333 _]
              tunnel: w291 -> [w332 _]
              tunnel: [w332 "探头地址"] -> w290
              tunnel: w289 -> [w331 _]
              tunnel: [w331 "报警记录标志？"] -> w288
              tunnel: w284 -> [w330 _]
              tunnel: [w330 "报警状态"] -> w283
              tunnel: w287 -> [w329 _]
              tunnel: [w329 "异常保存记录？"] -> w265
              tunnel: w286 -> [w328 _]
              tunnel: [w328 "发送次数"] -> w285
              tunnel: w282 -> [w327 _]
              tunnel: [w327 w338] -> w281
              tunnel: [w326 "缓存值"] -> w276
              tunnel: w275 -> [w326 _]
              frame False {
                # "没有内容改变，则传递"
              }
              frame True {
                # "有内容改变，重加载"
                n126 = Not(x=w343) -> (.not. x?=w342:bool)
                n127 = global read "全局变量-35点监测.vi" "COM口"() -> (w338:refnum<visa-resource-name>)
                n128 = local write "变了？"(w342) -> ()
              }
            }
            n129 = case shown="真" "报警方式变了？" {
              selector: "报警方式变了？" -> [_ w302]
              tunnel: w261 -> [w299 _]
              tunnel: [w299 w300] -> w260
              frame False {
                # "没变"
              }
              frame True {
                # "更新报警方式"
                n130 = Not(x=w302) -> (.not. x?=w301:bool)
                n131 = local write "报警方式变了？"(w301) -> ()
                n132 = local read "报警方式"() -> (w300:T1)
              }
            }
            n133 = case shown="真" "限值变了？" {
              tunnel: [w323 w325] -> w270
              tunnel: w268 -> [w323 _]
              frame False {
              }
              frame True {
                w324 = FALSE  # F
                # "仅修改限值"
                n134 = local write "限值变了？"(w324) -> ()
                n135 = local read "限值"() -> (w325:T4)
              }
            }
            n136 = case shown="真" w264 {
              tunnel: w263 -> [_ w303]
              frame False {
                # "未轮询完"
              }
              frame True {
                # "轮询完"
                n137 = flat-sequence {
                  tunnel: w303 -> [w312]
                  tunnel: [w305] -> w304
                  tunnel: w304 -> [w317]
                  frame #0 {
                    w307 = 1000.0  # 1000ms/s
                    # "动态计算最佳轮询间隔"
                    n138 = Get Date/Time In Seconds() -> (seconds since 1Jan1904=w305:timestamp)
                    n139 = Subtract "轮询间隔 s"(x=w305, y="一周期间隔") -> (x-y=w315:dbl)
                    n140 = Subtract(x=w315, y=1.0) -> (x-y=w313:dbl)
                    n141 = Divide(x=w313, y=w312) -> (x/y=w309:dbl)
                    n142 = Greater Or Equal To 0? "超 1s？"(x=w309) -> (x >= 0?=w311:bool)
                    n143 = Negate(x=w309) -> (-x=w310:dbl)
                    n144 = Select(t=w310, s=w311, f=w309) -> (s? t:f=w308:dbl)
                    n145 = Multiply(x=w308, y=w307) -> (x*y=w306:dbl)
                    n146 = local write "轮询间隔 ms"(w306) -> ()
                  }
                  frame #1 {
                    # "更新一周间隔值"
                    n147 = local write "一周期间隔"(w317) -> ()
                  }
                }
              }
            }
            n148 = case shown="真" w264 {
              tunnel: w292 -> [_ w360]
              tunnel: w270 -> [_ w359]
              tunnel: w283 -> [_ w358]
              tunnel: w290 -> [_ w357]
              tunnel: w296 -> [w344 _]
              tunnel: [w344 u8 0] -> w278
              tunnel: w266 -> [_ w355]
              tunnel: "更新列表？" -> [_ w352]
              tunnel: [_ w353] -> w267
              tunnel: w265 -> [_ w348]
              tunnel: w263 -> [_ w349]
              tunnel: w260 -> [_ w345]
              frame False {
                # "更新当前探头索引，通知全探头窗口更新显示"
              }
              frame True {
                w353 = TRUE  # T
                # "已轮询所有探头，更新显示，清零当前探头索引"
                n149 = Array Subset(array=w348, length=w349) -> (w347:bool[])  [unwired: 1 in]
                n150 = And Array Elements "有掉线的探头？"(Boolean array=w347) -> (logical AND=w350:bool)
                n151 = Not(x=w350) -> (.not. x?=w346:bool)
                n152 = local write "有掉线？"(w346) -> ()
                n153 = stacked-sequence {
                  tunnel: w360 -> [w366 w388]
                  tunnel: w359 -> [w365 w387]
                  tunnel: w358 -> [w367 w382]
                  tunnel: w357 -> [w368 _]
                  tunnel: w355 -> [w369 w389]
                  tunnel: "探头信息" -> [w364 w386]
                  tunnel: w352 -> [w363 _]
                  tunnel: "累积剂量" -> [w362 w381]
                  tunnel: w345 -> [w361 _]
                  frame #0 {
                    # "当前为列表窗口"
                    n154 = case shown="真" w363 {
                      tunnel: w369 -> [_ w378]
                      tunnel: w368 -> [_ w377]
                      tunnel: w367 -> [_ w376]
                      tunnel: w366 -> [_ w375]
                      tunnel: w365 -> [_ w374]
                      tunnel: w364 -> [_ w373]
                      tunnel: w362 -> [_ w372]
                      tunnel: w361 -> [_ w371]
                      frame False {
                      }
                      frame True {
                        n155 = control-ref of="实时数据列表"() -> (w379:refnum<vi>)
                        n156 = call "整合-测量信息至列表框.vi"("报警方式"=w371, "限值"=w374, "累积剂量"=w372, "测量值"=w375, "MCListbox引用句柄"=w379, "备注信息"=w373, "报警状态"=w376, "探头地址"=w377, "探头启用状态？"=w378) -> ("报警状态状态"=w370:enum16{"正常", "一级报警", "二级报警", "累积报警"})  [unwired: 2 in]
                        n157 = property on="报警状态" class="Enum (严格)"("Val(Sgnl)"=w370) -> ()  [unwired: 2 in, 2 out]
                      }
                    }
                  }
                  frame #1 {
                    # "当前为探头模块窗口"
                    n158 = local read "引用-更新数据信号"() -> (w383:refnum<vi>)
                    n159 = local read "引用-更新数据簇"() -> (w385:refnum<vi>)
                    n160 = Bundle By Name(cluster=T13 {"探头启用状态？"=[], "测量值"=[], "限值"=[], "报警状态"=[], "探头信息"=[], "累积剂量"=[]} ("输出簇"), "探头启用状态？"=w389, "测量值"=w388, "限值"=w387, "报警状态"=w382, "探头信息"=w386, "累积剂量"=w381) -> (w384:T13)
                    n161 = Array Max & Min(array=w382) -> (max value=w380:enum16{"正常", "一级报警", "二级报警", "累积报警"})  [unwired: 3 out]
                    n162 = stacked-sequence {
                      tunnel: w385 -> [w393 _]
                      tunnel: w384 -> [w392 _]
                      tunnel: w383 -> [_ w396]
                      frame #0 {
                        # "先更新数据"
                        n163 = property class="Ctl"(reference=w393, "Value"=w392) -> (error out=w391:errorcluster)  [unwired: 1 in, 1 out]
                        n164 = call <vilib>:"Clear Errors.vi"("error in (no error)"=w391) -> ()  [unwired: 5 in, 2 out]
                      }
                      frame #1 {
                        # "再通知更新"
                        n165 = property class="Ctl"(reference=w396, "Val(Sgnl)"=TRUE ("更新列表？")) -> (error out=w394:errorcluster)  [unwired: 1 in, 1 out]
                        n166 = call <vilib>:"Clear Errors.vi"("error in (no error)"=w394) -> ()  [unwired: 5 in, 2 out]
                      }
                    }
                    n167 = property on="报警状态" class="Enum (严格)"("Val(Sgnl)"=w380) -> ()  [unwired: 2 in, 2 out]
                  }
                }
              }
            }
            n168 = Increment(x=w278) -> (x+1=w274:i32)
            n169 = Format Value(format string="%02d" ("格式字符串"), value (0)=w274) -> (output string=w272:string)  [unwired: 1 in]
            n170 = case shown="真" w267 {
              frame False {
              }
              frame True {
                n171 = flat-sequence {
                  tunnel: [w319] -> w318
                  tunnel: w318 -> [w322]
                  frame #0 {
                    # "测间隔"
                    n172 = Tick Count (ms)() -> (millisecond timer value=w319:u32)
                    n173 = Subtract(x=w319, y="计时") -> (x-y=→"间隔":u32)
                  }
                  frame #1 {
                    n174 = local write "计时"(w322) -> ()
                  }
                }
              }
            }
            n175 = Concatenate Strings("实时通信：第 " ("字符串"), w272, " 号探头" ("字符串")) -> (w271:string)
            n176 = property on="状态与编辑" class="Bool (严格)"("BoolText.Text"=w271) -> ()  [unwired: 2 in, 2 out]
            "测量值" <- w292
          }
          frame "发送命令" {
            w435 = 3
            n177 = Index Array(array=w432, index=w411) -> (element=w434:u8)
            n178 = Increment(x=w434) -> (x+1=w433:u8)
            n179 = Index Array(array=w421, index=w411) -> (element=w425:i32)
            n180 = Index Array "读 缓存"(array=w410, index=w411) -> (element=w409:cluster{"X":timestamp[], "Y":dbl[]})
            n181 = global read "全局变量-35点监测.vi" "波特率"() -> (w420:enum16{"9600", "19200"})
            n182 = global read "全局变量-35点监测.vi" "COM口"() -> (w416:refnum<visa-resource-name>)
            n183 = Greater?(x=w433, y=w435) -> (0:w412:bool)
            n184 = Unbundle By Name(w409) -> ("Y"=w408:dbl[])
            n185 = Select(t=w435, s=w412, f=w433) -> (s? t:f=w431:i32)
            n186 = Empty Array?(array=w408) -> (empty?=w407:bool)
            n187 = case shown="\"9600\", 默认" w420 {
              tunnel: [u16 9600 u16 19200] -> w446
              frame "9600", Default {
              }
              frame "19200" {
              }
            }
            n188 = Not(x=w407) -> (.not. x?=w405:bool)
            n189 = Replace Array Subset "更新发送次数"(array=w432, new element=w431, index=w411) -> (w430:u8[])
            n190 = VISA Open(VISA resource name=w416) -> (VISA resource name=w438:refnum<visa-resource-name>, error out=w439:errorcluster)  [unwired: 1 in, 3 out]
            n191 = And(x=w405, y=w412) -> (x .and. y?=w406:bool)
            n192 = call-poly "VISA Configure Serial Port"("VISA resource name"=w438, "timeout (10sec)"=u32 50, "Enable Termination\nChar (T)"=FALSE ("Enable Termination\nChar (T)"), "baud rate (9600)"=w446, "error in (no error)"=w439) -> ("VISA resource name out"=w440:refnum<visa-resource-name>, "error out"=w441:errorcluster)  [unwired: 3 in, 6 out]
            n193 = case shown="真" w406 {
              tunnel: w414 -> [w447 w457]
              tunnel: w411 -> [_ w451]
              tunnel: [w447 w456] -> w413
              tunnel: w410 -> [w448 w452]
              tunnel: [w448 w449] -> w415
              frame False {
                # "原值：未报警"
              }
              frame True {
                w458 = FALSE  # F
                # "原：报警\n报警结束，生成记录、清除缓存"
                n194 = local read "事件-报警缓存"() -> (w455:refnum<user-event>)
                n195 = Index Array "读 缓存"(array=w452, index=w451) -> (element=w453:cluster{"X":timestamp[], "Y":dbl[]})
                n196 = Replace Array Subset "更新 报警记录标志"(array=w457, new element=w458, index=w451) -> (w456:bool[])
                n197 = Bundle("维数大小"=w451, "缓存值"=w453) -> (w454:T28)  [unwired: 1 in]
                n198 = Replace Array Subset "更新 清空缓存"(array=w452, new element=cluster{"X":timestamp[], "Y":dbl[]} {"X"=[], "Y"=[]} ("新元素/子数组"), index=w451) -> (w449:cluster{"X":timestamp[], "Y":dbl[]}[])
                n199 = Generate User Event(user event=w455, event data cluster=w454) -> ()  [unwired: 2 in, 2 out]
              }
            }
            n200 = VISA Set I/O Buffer Size(VISA resource name=w440, error in (no error)=w441) -> (VISA resource name out=w442:refnum<visa-resource-name>, error out=w443:errorcluster)  [unwired: 2 out]
            n201 = case shown="真" w412 {
              tunnel: w429 -> [w463 w470]
              tunnel: [w463 w469] -> w428
              tunnel: w411 -> [_ w466]
              tunnel: w424 -> [w462 w468]
              tunnel: [w462 w467] -> w423
              tunnel: w418 -> [w461 w465]
              tunnel: [w461 w464] -> w417
              frame False {
                # "通信正常"
              }
              frame True {
                # "多次无回应，认为掉线异常，将测量值置-1，用于判断掉线"
                n202 = Index Array(array=w470, index=w466) -> (element=w471:bool)
                n203 = in-place {
                  # "用“-1”表示掉线"
                  n204 = in-place-array #1(w468, w466) -> (w474:cluster{"X":timestamp, "Y":dbl})
                  n205 = Bundle By Name(cluster=w474, "Y"=-1.0 ("新元素/子数组")) -> (w473:cluster{"X":timestamp, "Y":dbl})
                  n206 = in-place-array #1(w473) -> (w467:cluster{"X":timestamp, "Y":dbl}[])  [unwired: 1 out]
                }
                n207 = case shown="真" w471 {
                  tunnel: w466 -> [_ w478]
                  tunnel: w470 -> [w476 w483]
                  tunnel: [w476 w481] -> w469
                  tunnel: w465 -> [w475 w477]
                  tunnel: [w475 w477] -> w464
                  frame False {
                  }
                  frame True {
                    w482 = FALSE  # F
                    # "不至位 Inf，等重连时自动同步"
                    # "探头掉线事件"
                    n208 = Increment(x=w478) -> (x+1=w479:i32)
                    n209 = local read "事件-探头掉线"() -> (w480:refnum<user-event>)
                    n210 = Replace Array Subset(array=w483, new element=w482, index=w478) -> (w481:bool[])
                    n211 = Generate User Event(user event=w480, event data cluster=w479) -> ()  [unwired: 2 in, 2 out]
                  }
                }
              }
            }
            n212 = call "发送命令.vi"("探头号"=w425) -> ("探头命令"=w419:string)
            n213 = VISA Write(VISA resource name=w442, write buffer=w419, error in (no error)=w443) -> (VISA resource name out=w427:refnum<visa-resource-name>, error out=w437:errorcluster)  [unwired: 1 out]
            n214 = flat-sequence {
              tunnel: w427 -> [w460]
              tunnel: [w460] -> w426
              frame #0 {
                # "通讯等待"
                n215 = Wait (ms)(milliseconds to wait=u32 0 ("毫秒倍数")) -> ()  [unwired: 1 out]
              }
            }
          }
          frame "接收数据" {
            n216 = VISA Read(VISA resource name=w510, byte count=u32 9 ("字节总数"), error in (no error)=w509) -> (VISA resource name out=w486:refnum<visa-resource-name>, read buffer=w494:string, error out=w489:errorcluster)  [unwired: 1 out]
            n217 = call "测量数据解析.vi"("完整输入"=w494) -> ("CRC？"=w492:bool, "测量值"=w493:dbl)  [unwired: 8 in, 1 out]
            n218 = case shown="真" w492 {
              tunnel: w493 -> [_ w532]
              tunnel: w495 -> [w516 w541]
              tunnel: w507 -> [w521 w553]
              tunnel: w506 -> [w517 w583]
              tunnel: w505 -> [w522 w572]
              tunnel: w504 -> [w523 w561]
              tunnel: w499 -> [_ w582]
              tunnel: w503 -> [w520 w581]
              tunnel: [w523 w568] -> w502
              tunnel: [w517 w544] -> w501
              tunnel: [w522 w546] -> w500
              tunnel: [w520 w579] -> w498
              tunnel: [w518 w578] -> w497
              tunnel: w491 -> [w519 w575]
              tunnel: [w519 w574] -> w490
              tunnel: w488 -> [w512 w543]
              tunnel: [w512 w538] -> w487
              tunnel: w486 -> [_ w540]
              frame False {
                w514 = u8 3  # 离线标志
                # "校验错误"
                n219 = Index Array "发送次数"(array=w517, index=w516) -> (element=w515:u8)
                n220 = Equal? "离线？"(x=w514, y=w515) -> (x = y?=w513:bool)
                n221 = case shown="假" w513 {
                  tunnel: w521 -> [w524 w528]
                  tunnel: [w524 w527] -> w518
                  tunnel: w516 -> [_ w525]
                  frame False {
                  }
                  frame True {
                    # "掉线的设备 设为“正常”\n防止报警时掉线无法停止报警"
                    # "离线则恢复为‘正常’"
                    n222 = Replace Array Subset "更新 报警状态"(array=w528, new element=enum16{"正常", "一级报警", "二级报警", "累积报警"}."正常" ("新元素/子数组"), index=w525) -> (w527:enum16{"正常", "一级报警", "二级报警", "累积报警"}[])
                  }
                }
              }
              frame True {
                w536 = enum16{"一级限值", "二级限值"}."一级限值"  # 一级
                w551 = enum16{"正常", "一级报警", "二级报警", "累积报警"}."累积报警"  # 累积报警
                w556 = timestamp(0 s since 1904-01-01)  # 初始化值
                w563 = 3600.0  # 3600s/h
                w565 = TRUE  # T
                w584 = TRUE  # T
                # "剂量率报警优先"
                # "CRC 校验正确"
                n223 = Get Date/Time In Seconds() -> (seconds since 1Jan1904=w559:timestamp)
                n224 = Index Array "读 限值"(array=w582, index=w541) -> (element=w577:T15)
                n225 = case shown="真" w565 {
                  tunnel: [_ w603] -> w571
                  tunnel: [_ w602] -> w570
                  tunnel: [_ w601] -> w569
                  tunnel: w541 -> [_ w599]
                  frame False {
                    # "禁用累积"
                  }
                  frame True {
                    # "启用累积"
                    n226 = local read "探头信息"() -> (w600:string[])
                    n227 = local read "累积剂量"() -> (w601:T2)
                    n228 = Index Array(array=w600, index=w599) -> (element=w598:string)
                    n229 = for {
                      tunnel: w601 -> [w610] mode=indexing
                      tunnel: w598 -> [w608]
                      tunnel: [w605] -> w602
                      tunnel: [w604] -> w603
                      i -> [w605]
                      stop <- w604 stop-if-true
                      # "查找匹配，获取索引"
                      n230 = Unbundle By Name(w610) -> ("设备名称"=w609:string, "启用累积？"=w606:bool)
                      n231 = Equal? "匹配？"(x=w608, y=w609) -> (x = y?=w607:bool)
                      n232 = And(x=w607, y=w606) -> (x .and. y?=w604:bool)
                    }
                  }
                }
                n233 = Unbundle By Name(w577) -> ("限值1"=w534:dbl, "限值2"=w533:dbl, "探头限值"=w537:enum16{"一级限值", "二级限值"})
                n234 = Bundle("seconds since 1Jan1904"=w559, "测量值"=w532) -> (w573:T29)  [unwired: 1 in]
                n235 = Replace Array Subset "更新 测量值"(array=w561, new element=w573, index=w541) -> (w568:cluster{"X":timestamp, "Y":dbl}[])
                n236 = Index Array "读 报警记录标志"(array=w581, index=w541) -> (element=w580:bool)
                n237 = Replace Array Subset "更新 异常保存？"(array=w572, new element=w584, index=w541) -> (w546:bool[])
                n238 = Equal?(x=w537, y=w536) -> (x = y?=w535:bool)
                n239 = Index Array "上个状态在线？"(array=w572, index=w541) -> (element=w548:bool)
                n240 = Index Array "实时数据"(array=w561, index=w541) -> (element=w560:cluster{"X":timestamp, "Y":dbl})
                n241 = Less? "正常？"(x=w532, y=w534) -> (x < y?=w542:bool)
                n242 = Replace Array Subset "更新 发送次数"(array=w583, new element=0, index=w541) -> (w544:u8[])
                n243 = Unbundle By Name(w560) -> ("X"=w554:timestamp)
                n244 = Not "重连？"(x=w548) -> (.not. x?=w547:bool)
                n245 = Select(t=w534, s=w535, f=w533) -> (s? t:f=w531:dbl)
                n246 = Equal? "首次？"(x=w554, y=w556) -> (x = y?=w555:bool)
                n247 = case shown="假" w548 {
                  tunnel: w541 -> [w629 _]
                  frame False {
                    # "上次不在线，这次重连上了"
                    n248 = local read "事件-探头重连"() -> (w630:refnum<user-event>)
                    n249 = Generate User Event(user event=w630, event data cluster=w629) -> ()  [unwired: 2 in, 2 out]
                  }
                  frame True {
                    # "上次在线，不执行"
                  }
                }
                n250 = Divide(x=w532, y=w563) -> (x/y=w564:dbl)
                n251 = Or "或"(x=w547, y=w555) -> (x .or. y?=w549:bool)
                n252 = Select(t=w559, s=w549, f=w554) -> (s? t:f=w558:timestamp)
                n253 = Subtract "采集间隔 s"(x=w559, y=w558) -> (x-y=w557:dbl)
                n254 = Multiply(x=w557, y=w564) -> (x*y=w562:dbl)
                n255 = Index Array "上个报警状态"(array=w553, index=w541) -> (element=w552:enum16{"正常", "一级报警", "二级报警", "累积报警"})
                n256 = case shown="真" w571 {
                  tunnel: w569 -> [_ w617]
                  tunnel: w570 -> [_ w616]
                  tunnel: w562 -> [_ w614]
                  tunnel: [_ w613] -> w545
                  tunnel: [_ w612] -> w529
                  tunnel: [_ w611] -> w566
                  frame False {
                    # "未匹配"
                  }
                  frame True {
                    # "匹配到"
                    n257 = in-place {
                      in-place-border: w614 -> [w621]
                      in-place-border: [w620] -> w613
                      in-place-border: [w619] -> w612
                      in-place-border: [w618] -> w611
                      n258 = in-place-array #2(w617, w616) -> (w622:T20)
                      n259 = in-place {
                        in-place-border: w621 -> [w628]
                        in-place-border: [w626] -> w620
                        in-place-border: [w624] -> w619
                        n260 = in-place-cluster #3(w622) -> ("累积剂量"=w625:dbl, "累积报警阈值"=w623:dbl)
                        n261 = Add(x=w628, y=w625) -> (x+y=w627:dbl)
                        n262 = Greater?(x=w625, y=w623) -> (0:w624:bool)
                        n263 = Greater?(x=w627, y=w623) -> (0:w626:bool)
                        n264 = in-place-cluster #3("累积剂量"=w627, "累积报警阈值"=w623) -> (w618:T20)
                      }
                      n265 = in-place-array #2(w618) -> (w615:T2)  [unwired: 1 out]
                    }
                    n266 = local write "累积剂量"(w615) -> ()
                  }
                }
                n267 = Less? "探头未报警？"(x=w532, y=w531) -> (x < y?=w530:bool)
                n268 = case shown="假" w542 {
                  tunnel: w532 -> [w635 _]
                  tunnel: w533 -> [w634 _]
                  tunnel: [w631 w637] -> w576
                  tunnel: w545 -> [_ w640]
                  frame False {
                    w633 = enum16{"正常", "一级报警", "二级报警", "累积报警"}."一级报警"  # 一级报警
                    w632 = enum16{"正常", "一级报警", "二级报警", "累积报警"}."二级报警"  # 二级报警
                    # "报警"
                    n269 = Greater?(x=w635, y=w634) -> (0:w636:bool)
                    n270 = Select(t=w632, s=w636, f=w633) -> (s? t:f=w631:enum16{"正常", "一级报警", "二级报警", "累积报警"})
                  }
                  frame True {
                    w638 = enum16{"正常", "一级报警", "二级报警", "累积报警"}."累积报警"  # 累积
                    w639 = enum16{"正常", "一级报警", "二级报警", "累积报警"}."正常"  # 正常
                    # "正常"
                    n271 = Select(t=w638, s=w640, f=w639) -> (s? t:f=w637:enum16{"正常", "一级报警", "二级报警", "累积报警"})
                  }
                }
                n272 = Equal?(x=w552, y=w551) -> ()  [unwired: 1 out]
                n273 = Replace Array Subset "更新 报警状态"(array=w553, new element=w576, index=w541) -> (w578:enum16{"正常", "一级报警", "二级报警", "累积报警"}[])
                n274 = case shown="真" w542 {
                  tunnel: w532 -> [_ _]
                  tunnel: w580 -> [w648 w671]
                  tunnel: w541 -> [w641 w673]
                  tunnel: w581 -> [w650 w674]
                  tunnel: [w649 w672] -> w579
                  tunnel: w575 -> [w643 w670]
                  tunnel: [w646 w669] -> w574
                  tunnel: w573 -> [w647 _]
                  frame False {
                    # "现：报警"
                    n275 = Array Size(array=w643) -> (size(s)=w644:i32)
                    n276 = in-place {
                      in-place-border: w647 -> [w654]
                      # "插入新测量值"
                      n277 = in-place-array #4(w643, w641) -> (w656:cluster{"X":timestamp[], "Y":dbl[]})
                      n278 = in-place {
                        in-place-border: w654 -> [w661]
                        n279 = in-place-cluster #5(w656) -> ("X"=w663:timestamp[], "Y"=w662:dbl[])
                        n280 = Unbundle(w661) -> ("seconds since 1Jan1904"=w660:timestamp, "测量值"=w659:dbl)
                        n281 = Insert Into Array(array=w663, new element=w660) -> (w657:timestamp[])  [unwired: 1 in]
                        n282 = Insert Into Array(array=w662, new element=w659) -> (w658:dbl[])  [unwired: 1 in]
                        n283 = in-place-cluster #5("X"=w657, "Y"=w658) -> (w655:cluster{"X":timestamp[], "Y":dbl[]})
                      }
                      n284 = in-place-array #4(w655) -> (w646:cluster{"X":timestamp[], "Y":dbl[]}[])  [unwired: 1 out]
                    }
                    n285 = case shown="假" w648 {
                      tunnel: w641 -> [w667 _]
                      tunnel: w650 -> [w666 w668]
                      tunnel: [w665 w668] -> w649
                      frame False {
                        w664 = TRUE  # T
                        # "原：未报警"
                        n286 = Replace Array Subset "更新 报警记录标志"(array=w666, new element=w664, index=w667) -> (w665:bool[])
                      }
                      frame True {
                        # "原：报警"
                      }
                    }
                    n287 = Equal?(x=w644, y=10 ("x")) -> (x = y?=w642:bool)
                    n288 = case shown="真" w642 {
                      tunnel: w641 -> [_ w652]
                      frame False {
                      }
                      frame True {
                        n289 = local read "探头信息"() -> (w653:string[])
                        n290 = Index Array(array=w653, index=w652) -> (element=w651:string)
                        n291 = call "短信通知-发送.vi"("探头名称"=w651) -> ()  [unwired: 11 in]
                      }
                    }
                  }
                  frame True {
                    # "现：未报警"
                    n292 = case shown="真" w671 {
                      tunnel: w674 -> [w675 w685]
                      tunnel: w673 -> [_ w679]
                      tunnel: [w675 w684] -> w672
                      tunnel: w670 -> [w676 w680]
                      tunnel: [w676 w677] -> w669
                      frame False {
                        # "原值：未报警"
                      }
                      frame True {
                        w686 = FALSE  # F
                        # "原：报警\n报警结束，生成记录、清除缓存"
                        n293 = local read "事件-报警缓存"() -> (w683:refnum<user-event>)
                        n294 = Index Array "读 缓存"(array=w680, index=w679) -> (element=w681:cluster{"X":timestamp[], "Y":dbl[]})
                        n295 = Replace Array Subset "更新 报警记录标志"(array=w685, new element=w686, index=w679) -> (w684:bool[])
                        n296 = Bundle("维数大小"=w679, "缓存值"=w681) -> (w682:T28)  [unwired: 1 in]
                        n297 = Replace Array Subset "更新 清空缓存"(array=w680, new element=cluster{"X":timestamp[], "Y":dbl[]} {"X"=[], "Y"=[]} ("新元素/子数组"), index=w679) -> (w677:cluster{"X":timestamp[], "Y":dbl[]}[])
                        n298 = Generate User Event(user event=w683, event data cluster=w682) -> ()  [unwired: 2 in, 2 out]
                      }
                    }
                  }
                }
                n299 = Not(x=w529) -> (.not. x?=w550:bool)
                n300 = And(x=w545, y=w550) -> (x .and. y?=w567:bool)
                n301 = in-place {
                  in-place-border: w531 -> [w592]
                  in-place-border: w530 -> [w591]
                  in-place-border: w541 -> [w590]
                  in-place-border: w540 -> [w588]
                  in-place-border: [w587] -> w539
                  # "报警方式处理"
                  n302 = in-place-array #6(w543, w541) -> (w594:T27)
                  n303 = Increment(x=w590) -> (x+1=w589:i32)
                  n304 = call "报警方式处理模块.vi"("未报警状态？"=w591, "VISA资源名称"=w588, "探头地址"=w589, "探头限值"=w592, "报警方式 i"=w594) -> ("值改变？"=w587:bool, "报警方式 o"=w593:T27)  [unwired: 5 in]
                  n305 = in-place-array #6(w593) -> (w538:T1)  [unwired: 1 out]
                }
                n306 = case shown="真" w567 {
                  tunnel: w566 -> [_ w596]
                  frame False {
                  }
                  frame True {
                    w595 = TRUE  # T
                    # "原来未报警，现在报警了，\n记录一条报警记录到 DB"
                    n307 = local read "事件-累积剂量"() -> (w597:refnum<user-event>)
                    n308 = Generate User Event(user event=w597, event data cluster=w596) -> ()  [unwired: 2 in, 2 out]
                    "标志-首次累积报警" <- w595
                  }
                }
                n309 = case shown="假" w539 {
                  tunnel: w538 -> [_ w586]
                  frame False {
                    # "值未变"
                  }
                  frame True {
                    # "值改变"
                    n310 = local write "报警方式"(w586) -> ()
                  }
                }
              }
            }
          }
          frame "暂停发送" {
            n311 = global read "全局变量-35点监测.vi" "最大探头数"() -> (w695:i32)
            n312 = Divide(x=1000.0 ("最大探头数"), y=w695) -> (x/y=w696:dbl)
            n313 = Add(x="轮询间隔 ms", y=w696) -> (x+y=w691:dbl)
            n314 = Greater Or Equal To 0?(x=w691) -> (x >= 0?=w690:bool)
            n315 = Select(t=w691, s=w690, f=0.0) -> (s? t:f=w689:dbl)
            n316 = Wait (ms)(milliseconds to wait=w689) -> (millisecond timer value=w687:u32)
            n317 = stacked-sequence {
              tunnel: ["暂停发送"] -> w697
              tunnel: w687 -> [_]
              frame #0 {
              }
            }
            n318 = case shown="真" w697 {
              frame False {
              }
              frame True {
                # "暂停发送，增加延迟"
                n319 = Wait (ms)(milliseconds to wait=u32 100 ("等待时间（毫秒）")) -> ()  [unwired: 1 out]
              }
            }
            n320 = local read "停止"() -> (w698:bool)
            n321 = Select(t=T9."暂停发送", s=w697, f=T9."扫描探头") -> (s? t:f=w713:T9)
            n322 = Select(t=T9."结束程序", s=w698, f=w713) -> (s? t:f=w714:T9)
          }
          frame "结束程序" {
            w717 = T25 {"COM"="", "探头地址"=[], "探头启用状态？"=[], "开机启动？"=FALSE, "探头信息"=[], "限值"=[], "最大探头数"=0, "波特率"=enum."19200", "周期"=0, "报警方式"=[], "静音延迟"=0}  # 配置内容
            n323 = VISA Close(VISA resource name=w742, error in (no error)=w744) -> (error out=w745:errorcluster)
            n324 = global read "全局变量-35点监测.vi" "波特率"() -> (w724:enum16{"9600", "19200"})
            n325 = local read "探头启用状态？"() -> (w730:bool[])
            n326 = call <vilib>:"Clear Errors.vi"("error in (no error)"=w745) -> ()  [unwired: 5 in, 2 out]
            n327 = global read "全局变量-35点监测.vi" "最大探头数"() -> (w727:i32)
            n328 = local read "探头信息"() -> (w728:string[])
            n329 = local read "开机启动"() -> (w741:bool)
            n330 = global read "全局变量-35点监测.vi" "静音延迟 s"() -> (w718:u16)
            n331 = local read "周期"() -> (w720:i64)
            n332 = Bundle By Name(cluster=w717, "静音延迟"=w718, "周期"=w720, "限值"=w725, "COM"=w742, "探头地址"=w733, "探头启用状态？"=w730, "最大探头数"=w727, "开机启动？"=w741, "探头信息"=w728, "波特率"=w724, "报警方式"=w719) -> (w740:T25)
            n333 = local read "累积剂量"() -> (w723:T2)
            n334 = Flatten To XML(anything=w740) -> (xml string=w739:string)
            n335 = Flatten To XML(anything=w723) -> (xml string=w722:string)
            n336 = call "路径查找创建-报警记录清单.vi"() -> ("配置文件"=w726:path, "累积剂量配置文件"=w721:path)  [unwired: 8 in, 10 out]
            n337 = call-poly <vilib>:"Write to XML File.vi"("XML Input"=w739, "XML File Path"=w726) -> ()  [unwired: 7 in, 3 out]
            n338 = call-poly <vilib>:"Write to XML File.vi"("XML Input"=w722, "XML File Path"=w721) -> ()  [unwired: 7 in, 3 out]
            n339 = local read "device ID"() -> (w731:refnum<k1>)
            n340 = call-poly <vilib>:"Close Input Device.vi"("device ID"=w731) -> ()  [unwired: 9 in, 1 out]
          }
          frame "退出" {
            n341 = Quit LabVIEW() -> ()  [unwired: 1 in]
          }
        }
        n342 = Equal?(x=w195, y=T9."退出") -> (x = y?=w196:bool)
      }
      n343 = while {
        tunnel: w93 -> [w814]
        stop <- w815 stop-if-true
        # "事件结构"
        n344 = event shown="[25] \"报警记录列表\": 键按下" {
          selector: w814 -> [_ _ _ _ _ _ _ _ _ _ _ _ _ _ _ _ _ _ _ _ _ _ _ _ _ _ _ _ _ _]
          dyn-events: _ -> [_ _ _ _ _ _ _ _ _ _ _ _ _ _ _ _ _ _ _ _ _ _ _ _ _ _ _ _ _ _]
          timeout: _ -> [_ _ _ _ _ _ _ _ _ _ _ _ _ _ _ _ _ _ _ _ _ _ _ _ _ _ _ _ _ _]
          tunnel: [_ w817 _ _ _ _ _ _ _ _ _ _ _ _ _ _ _ _ _ _ _ _ _ _ _ _ _ _ _ _] -> w815
          event Timeout {
            # "每分钟 保存配置"
            n345 = event-data() -> ()  [unwired: 1 in, 3 out]
          }
          event "停止信号": Value Change {
            # "触发停止"
            n346 = event-data() -> ("NewVal"=w816:enum16{"内部停止信号", "外部停止信号"})  [unwired: 1 in, 5 out]
            n347 = case shown="\"外部停止信号\"" w816 {
              tunnel: [w818 w819] -> w817
              frame "内部停止信号", Default {
                # "内部停止信号，需弹窗"
                n348 = call "显示对话框信息3"() -> ("确定"=w818:bool)  [unwired: 10 in, 1 out]
              }
              frame "外部停止信号" {
                w819 = TRUE  # T
                # "外部停止信号，不弹窗"
              }
            }
            "停止" <- w817
            n349 = case shown="真" w817 {
              frame False {
              }
              frame True {
                # "停止，关闭平行运行的通知窗口"
                n350 = local read "通知窗口VI-引用"() -> (w829:refnum<vi>)
                n351 = local read "手动静音窗口VI-引用"() -> (w821:refnum<vi>)
                n352 = invoke class="VI" method="Abort VI"(reference=w829) -> (reference out=w827:refnum<vi>, error out=w826:errorcluster)  [unwired: 2 in, 1 out]
                n353 = call <vilib>:"Stop Timed Structure.vi"("name"="累积剂量记录" ("源名称")) -> ("error out"=w824:errorcluster)  [unwired: 10 in]
                n354 = invoke class="VI (严格)" method="Abort VI"(reference=w821) -> (reference out=w822:refnum<vi>, error out=w823:errorcluster)  [unwired: 2 in, 1 out]
                n355 = call <vilib>:"Clear Errors.vi"("error in (no error)"=w824) -> ()  [unwired: 5 in, 2 out]
                n356 = invoke class="VI" method="FP.Close"(reference=w827, error in=w826) -> (error out=w828:errorcluster)  [unwired: 1 in, 2 out]
                n357 = invoke class="VI (严格)" method="FP.Close"(reference=w822, error in=w823) -> (error out=w820:errorcluster)  [unwired: 1 in, 2 out]
                n358 = call <vilib>:"Clear Errors.vi"("error in (no error)"=w828) -> ()  [unwired: 5 in, 2 out]
                n359 = call <vilib>:"Clear Errors.vi"("error in (no error)"=w820) -> ()  [unwired: 5 in, 2 out]
              }
            }
          }
          event Panel Close? {
            w831 = TRUE  # T
            n360 = event-data() -> ()  [unwired: 1 in, 4 out]
            n361 = property on="停止信号" class="Enum (严格)"("Val(Sgnl)"=enum16{"内部停止信号", "外部停止信号"}."内部停止信号" ("值(信号)")) -> ()  [unwired: 2 in, 2 out]
            n362 = event-data("Discard?"=w831) -> ()  [unwired: 1 in, 1 out]
          }
          event User Event {
            # "报警记录缓存结束，生成记录，生成报告"
            n363 = event-data() -> ("缓存值"=w832:cluster{"X":timestamp[], "Y":dbl[]}, "探头索引"=w833:i32)  [unwired: 1 in, 4 out]
            n364 = stacked-sequence {
              tunnel: w833 -> [w838 _]
              tunnel: w832 -> [w837 _]
              frame #0 {
                # "生成记录数据"
                n365 = local read "探头地址"() -> (w841:i32[])
                n366 = local read "探头信息"() -> (w840:string[])
                n367 = local read "限值"() -> (w839:T4)
                n368 = Index Array(array=w841, index=w838) -> (element=w836:i32)
                n369 = Index Array(array=w840, index=w838) -> (element=w835:string)
                n370 = Index Array(array=w839, index=w838) -> (element=w834:T15)
                n371 = call "生成-报警记录缓存数据文件-分类计时版.vi"("缓存绘图数据"=w837, "限值"=w834, "探头信息"=w835, "探头地址"=w836) -> ()  [unwired: 8 in]
              }
              frame #1 {
                w842 = enum16{"刷新", "预览并生成报表", "删除记录"}."刷新"  # 刷新
                # "立刻刷新报警列表"
                n372 = property on="菜单项-报警列表" class="Enum (严格)"("Val(Sgnl)"=w842) -> ()  [unwired: 2 in, 2 out]
              }
            }
          }
          event User Event {
            # "通知栏提示掉线"
            n373 = event-data() -> ("掉线探头索引"=w846:u32)  [unwired: 1 in, 4 out]
            n374 = Number To Decimal String(number=w846) -> (decimal integer string=w845:string)  [unwired: 1 in]
            n375 = Concatenate Strings(w845, "号探头掉线" ("字符串")) -> (w843:string)
            n376 = call "状态栏-插入状态信息-35点监测专用.vi"("消息内容"=w843, "状态类型"=enum16{"全部", "报警", "通信", "设置"}."通信") -> ()  [unwired: 10 in]
          }
          event User Event {
            n377 = event-data() -> ("重连探头索引"=w848:u32)  [unwired: 1 in, 4 out]
            n378 = stacked-sequence {
              tunnel: w848 -> [_ w859 _]
              frame #0 {
                # "暂停发送"
                n379 = local write "暂停发送"(TRUE ("暂停发送")) -> ()
              }
              frame #1 {
                w854 = enum16{"一级限值", "二级限值"}."一级限值"  # 一级
                # "同步报警限值"
                n380 = local read "探头信息"() -> (w860:string[])
                n381 = local read "限值"() -> (w864:T4)
                n382 = Index Array(array=w864, index=w859) -> (element=w880:T15)
                n383 = Index Array(array=w860, index=w859) -> (element=w857:string)
                n384 = Unbundle By Name(w880) -> ("探头限值"=w855:enum16{"一级限值", "二级限值"}, "限值1"=w852:dbl, "限值2"=w851:dbl)
                n385 = Increment(x=w859) -> (x+1=w858:u32)
                n386 = Equal?(x=w854, y=w855) -> (x = y?=w853:bool)
                n387 = Select(t=w852, s=w853, f=w851) -> (s? t:f=w850:dbl)
                n388 = call "创建文本3"("探头编号"=w858, "探头名称"=w857) -> ("Result"=w856:string)  [unwired: 12 in, 1 out]
                n389 = Greater Or Equal?(x=w850, y=1000.0) -> (x >= y?=w878:bool)
                n390 = Increment(x=w859) -> (x+1=w884:u32)
                n391 = Multiply(x=w850, y=10) -> (x*y=w882:dbl)
                n392 = Boolean To (0,1)(Boolean=w878) -> (0, 1=w877:i16)
                n393 = To Unsigned Word Integer(number=w882) -> (unsigned 16bit integer=w883:u16)
                n394 = To Unsigned Byte Integer(number=w884) -> (unsigned 8bit integer=w885:u8)
                n395 = To Unsigned Byte Integer(number=w877) -> (unsigned 8bit integer=w876:u8)
                n396 = Type Cast "数值"(x=w883) -> (*(type *) &x=w867:string)  [unwired: 1 in]
                n397 = Type Cast "单位"(x=w876) -> (*(type *) &x=w866:string)  [unwired: 1 in]
                n398 = Type Cast "编号"(x=w885) -> (*(type *) &x=w868:string)  [unwired: 1 in]
                n399 = global read "全局变量-35点监测.vi" "COM口"() -> (w861:refnum<visa-resource-name>)
                n400 = Concatenate Strings(w868, "\t\u0000", w867, w866) -> (w869:string)
                n401 = call "CRC16-发送校验.vi"("净数据"=w869) -> ("完整输出"=w871:string)
                n402 = VISA Write(VISA resource name=w861, write buffer=w871) -> (VISA resource name out=w873:refnum<visa-resource-name>, error out=w872:errorcluster)  [unwired: 1 in, 1 out]
                n403 = VISA Read(VISA resource name=w873, byte count=u32 9 ("字节总数"), error in (no error)=w872) -> (return count=w865:u32, error out=w875:errorcluster)  [unwired: 2 out]
                n404 = call <vilib>:"Clear Errors.vi"("error in (no error)"=w875) -> ()  [unwired: 5 in, 2 out]
                n405 = Greater Than 0?(x=w865) -> (x > 0?=w862:bool)
                n406 = case shown="真" w862 {
                  tunnel: w856 -> [_ w886]
                  frame False {
                  }
                  frame True {
                    # "有回复，设置成功"
                    n407 = call "状态栏-插入状态信息-35点监测专用.vi"("消息内容"=w886, "状态类型"=enum16{"全部", "报警", "通信", "设置"}."设置") -> ()  [unwired: 10 in]
                  }
                }
                n408 = Wait (ms)(milliseconds to wait=u32 70 ("等待时间（毫秒）")) -> ()  [unwired: 1 out]
              }
              frame #2 {
                w889 = TRUE  # T
                # "恢复发送"
                n409 = local write "限值变了？"(w889) -> ()
                n410 = local write "暂停发送"(FALSE ("暂停发送")) -> ()
              }
            }
          }
          event User Event {
            # "生成累积剂量，保存到数据库"
            n411 = event-data() -> ("设备名称"=w893:string, "起始时间"=w892:timestamp, "累积剂量"=w891:dbl, "累积报警阈值"=w890:dbl)  [unwired: 1 in, 4 out]
            n412 = local read "累积剂量"() -> (w895:T2)
            n413 = call "查找匹配累积剂量.vi"("探头名称"=w893, "累积剂量"=w895) -> ("匹配？"=w894:bool)  [unwired: 7 in, 2 out]
            n414 = case shown="真" w894 {
              tunnel: w893 -> [_ w906]
              tunnel: w892 -> [_ w900]
              tunnel: w891 -> [_ w909]
              tunnel: w890 -> [_ w911]
              frame False {
                # "无匹配，不执行"
              }
              frame True {
                # "有匹配，插入新数据"
                n415 = Equal? "空值？"(x=timestamp(0 s since 1904-01-01), y=w900) -> (x = y?=w902:bool)
                n416 = case shown="假" w902 {
                  tunnel: [w923 w924] -> w901
                  tunnel: w900 -> [w923 _]
                  frame False {
                    # "非空，不需初始化"
                  }
                  frame True {
                    # "初始化为今日"
                    n417 = Get Date/Time In Seconds() -> (seconds since 1Jan1904=w924:timestamp)
                  }
                }
                n418 = Greater?(x=w909, y=w911) -> (0:w910:bool)
                n419 = Format Date/Time String "日期时间"(time format string (%c)="%Y-%m-%d %H:%M:%S" ("时间格式字符串(%c)"), seconds (now)=w901) -> (date/time string=w912:string)  [unwired: 1 in]
                n420 = local read "标志-首次累积报警"() -> (w896:bool)
                n421 = call "今日-日期时间字符串.vi"() -> ("日期时间"=w914:string)  [unwired: 9 in, 2 out]
                n422 = Bundle By Name(cluster=T14 {"记录时间"="", "起始时间"="", "累积剂量"=0.0, "报警"=FALSE, "记录名称"=""} ("单条数据"), "记录名称"=w906, "记录时间"=w914, "起始时间"=w912, "累积剂量"=w909, "报警"=w910) -> (w899:T14)
                n423 = case shown="真" w896 {
                  selector: w896 -> [_ w916]
                  tunnel: w899 -> [_ w917]
                  frame False {
                  }
                  frame True {
                    # "由于首次报警而触发的事件"
                    n424 = Not(x=w916) -> (.not. x?=w915:bool)
                    n425 = vi-ref "弹窗-累积超限通知.vi"() -> (w918:refnum<vi>)
                    n426 = local write "标志-首次累积报警"(w915) -> ()
                    n427 = property class="VI接口类型9"(reference=w918) -> ("Name"=w919:string)  [unwired: 1 in, 2 out]
                    n428 = Open VI Reference(type specifier VI Refnum (for type only)=refnum<vi> refnum ("类型说明符VI引用句柄（仅用于类型）"), vi path=w919, options=128 ("选项")) -> (vi reference=w921:refnum<vi>)  [unwired: 3 in, 1 out]
                    n429 = call-by-ref "开始异步调用"(reference=w921, "报警信息"=w917) -> ()  [unwired: 12 in, 2 out]
                  }
                }
                n430 = call "连接数据库.vi"() -> ("error out"=w905:errorcluster, "connection reference"=w908:T30)  [unwired: 10 in]
                n431 = call "插入数据.vi"("error in (no error)"=w905, "单条数据"=w899, "数据库连接引用 i"=w908) -> ("error out"=w897:errorcluster, "数据库连接引用 o"=w904:T30)  [unwired: 7 in]
                n432 = call <vilib>:"DB Tools Close Connection.vi"("error in (no error)"=w897, "connection reference"=w904) -> ("error out"=w898:errorcluster)  [unwired: 5 in]
                n433 = call <vilib>:"Clear Errors.vi"("error in (no error)"=w898) -> ()  [unwired: 5 in, 2 out]
              }
            }
          }
          event "信号-设置": Value Change {
            n434 = event-data() -> ()  [unwired: 1 in, 6 out]
            n435 = stacked-sequence {
              frame #0 {
                # "弹窗设置，暂停读数据，在设置完报警值后 恢复发送"
                n436 = flat-sequence {
                  frame #0 {
                    w927 = 3600000.0  # 1小时
                    n437 = control-ref of="暂停发送"() -> (w932:refnum<vi>)
                    n438 = control-ref of="本VI"() -> (w933:refnum<vi>)
                    n439 = local read "测量值"() -> (w926:cluster{"X":timestamp, "Y":dbl}[])
                    n440 = control-ref of="实时数据列表"() -> (w925:refnum<vi>)
                    n441 = local read "周期"() -> (w931:i64)
                    n442 = Divide(x=w931, y=w927) -> (x/y=w929:dbl)
                    n443 = call-by-ref "?"("存储间隔（小时）"=w929, "VI引用句柄"=w933, "实时数据列表"=w925, "测量值"=w926, "暂停发送-引用"=w932) -> ("存储间隔（h）"=w930:dbl)  [unwired: 8 in, 2 out]
                    n444 = Multiply(x=w927, y=w930) -> (x*y=w928:dbl)
                    n445 = local write "周期"(w928) -> ()
                  }
                  frame #1 {
                    n446 = global read "全局变量-35点监测.vi" "波特率"() -> (w938:enum16{"9600", "19200"})
                    n447 = global read "全局变量-35点监测.vi" "COM口"() -> (w939:refnum<visa-resource-name>)
                    n448 = Equal To 0?(x=w938) -> (x = 0?=w937:bool)
                    n449 = Select(t="9600" ("当前波特率"), s=w937, f="19200" ("当前波特率")) -> (s? t:f=w934:string)
                    n450 = local write "当前端口"(w939) -> ()
                    n451 = local write "当前波特率"(w934) -> ()
                  }
                }
              }
              frame #1 {
                w946 = T27 {"报警方式"=enum."常报警", "延迟计时"=0, "报警中？"=TRUE}  # 默认报警方式
                w959 = inf
                w966 = TRUE  # T
                w967 = FALSE  # F
                # "将未显示的“限值”和“探头名称”重新初始化，\n防止下次变动时冲突"
                # "依据最大探头数，修改探头启用"
                n452 = global read "全局变量-35点监测.vi" "最大探头数"() -> (w944:i32)
                n453 = local read "限值"() -> (w960:T4)
                n454 = local read "探头信息"() -> (w950:string[])
                n455 = Bundle(cluster=T15 {"限值1"=0.0, "限值2"=0.0, "探头限值"=enum."一级限值"} ("探头限值簇"), "限值1"=w959, "限值2"=w959, "探头限值"=enum16{"一级限值", "二级限值"}."一级限值") -> (w958:T15)
                n456 = Subtract(x=32, y=w944) -> (x-y=w947:i32)
                n457 = Initialize Array(w958, w947) -> (w957:T4)
                n458 = Initialize Array("", w947) -> (w949:string[])
                n459 = Initialize Array(w946, w947) -> (w943:T1)
                n460 = Initialize Array(w967, w947) -> (w964:bool[])
                n461 = Initialize Array(w966, w944) -> (w965:bool[])
                n462 = Replace Array Subset(array=w950, new element=w949, index=w944) -> (w948:string[])
                n463 = Replace Array Subset(array=w960, new element=w957, index=w944) -> (w956:T4)
                n464 = Replace Array Subset(array="报警方式", new element=w943, index=w944) -> (w942:T1)
                n465 = Insert Into Array(array=bool[] [] ("数组"), new element #1=w965, new element #2=w964) -> (w962:bool[])  [unwired: 1 in]
                n466 = local write "探头信息"(w948) -> ()
                n467 = local write "探头启用状态？"(w962) -> ()
                n468 = flat-sequence {
                  tunnel: w942 -> [w969]
                  frame #0 {
                    n469 = local write "报警方式"(w969) -> ()
                  }
                  frame #1 {
                    w970 = TRUE  # T
                    n470 = local write "报警方式变了？"(w970) -> ()
                  }
                }
                n471 = flat-sequence {
                  tunnel: w956 -> [w974]
                  frame #0 {
                    n472 = local write "限值"(w974) -> ()
                  }
                  frame #1 {
                    w975 = TRUE  # T
                    n473 = local write "限值变了？"(w975) -> ()
                  }
                }
                n474 = local read "监测数量限值"() -> (w955:cluster{"min":i32, "max":i32})
                n475 = Wait (ms)(milliseconds to wait=u32 1000 ("等待时间（毫秒）")) -> ()  [unwired: 1 out]
                n476 = Unbundle By Name(w955) -> ("max"=w954:i32, "min"=w953:i32)
                n477 = In Range and Coerce(upper limit=w954, x=w944, lower limit=w953) -> (In Range?=w952:bool)  [unwired: 1 out]
                n478 = case shown="假" w952 {
                  frame False {
                    # "范围外，关闭监测VI"
                    n479 = local read "监-停止信号"() -> (w973:refnum<vi>)
                    n480 = property class="Ctl"(reference=w973, "Val(Sgnl)"=TRUE) -> (error out=w971:errorcluster)  [unwired: 1 in, 1 out]
                    n481 = call <vilib>:"Clear Errors.vi"("error in (no error)"=w971) -> ()  [unwired: 5 in, 2 out]
                  }
                  frame True {
                    # "范围内，不停止监测VI"
                  }
                }
              }
              frame #2 {
                # "同步： 数据库累积剂量设备表 与 “累积剂量”变量"
                n482 = call "连接数据库.vi"() -> ("error out"=w978:errorcluster, "connection reference"=w979:T30)  [unwired: 10 in]
                n483 = local read "累积剂量"() -> (w981:T2)
                n484 = call "从数据库同步累积剂量.vi"("error in (no error)"=w978, "累积剂量 i"=w981, "数据库连接引用 i"=w979) -> ("数据库连接引用 o"=w977:T30, "error out"=w976:errorcluster, "累积剂量 o"=w980:T2)  [unwired: 5 in, 1 out]
                n485 = local write "累积剂量"(w980) -> ()
                n486 = call <vilib>:"DB Tools Close Connection.vi"("error in (no error)"=w976, "connection reference"=w977) -> ()  [unwired: 5 in, 1 out]
              }
              frame #3 {
                w984 = TRUE  # T
                # "确认"
                n487 = local write "确认设置"(w984) -> ()
                n488 = call <vilib>:"Stop Timed Structure.vi"("name"="累积剂量记录" ("源名称")) -> ("error out"=w982:errorcluster)  [unwired: 10 in]
                n489 = call <vilib>:"Clear Errors.vi"("error in (no error)"=w982) -> ()  [unwired: 5 in, 2 out]
              }
              frame #4 {
                # "保存配置"
                n490 = property on="信号-保存配置" class="Bool (严格)"("Val(Sgnl)"=FALSE ("值(信号)")) -> ()  [unwired: 2 in, 2 out]
              }
            }
          }
          event "实时数据列表", "报警记录列表": Mouse Down {
            # "使  右击行  列表能够获取焦点"
            n491 = event-data() -> ("CtlRef"=w990:refnum<vi>, "Coords"=w992:T31)  [unwired: 1 in, 7 out]
            n492 = property class="MCListbox (严格)"(reference=w990) -> ("Label.Text"=w989:string)  [unwired: 1 in, 2 out]
            n493 = invoke class="多列列表框 (严格)" method="Point To Row Column"(reference=w990, "Point"=w992) -> ("CellPosition"=w991:T5)  [unwired: 5 in, 6 out]
            "点到行列-实时列表" <- w991
            n494 = property on="实时数据列表" class="MCListbox (严格)"() -> ("Label.Text"=w988:string)  [unwired: 2 in, 2 out]
            n495 = call-poly <vilib>:"Acquire Input Data.vi"("device ID"="device ID") -> ("button info"=w994:T32)  [unwired: 15 in, 3 out]
            n496 = Unbundle By Name "btn_2"(w994) -> ("button 2"=w993:bool)
            n497 = Equal?(x=w989, y=w988) -> (x = y?=w987:bool)
            n498 = case shown="真" w993 {
              tunnel: w990 -> [_ w1010]
              tunnel: w991 -> [_ w1008]
              tunnel: w987 -> [_ w1002]
              frame False {
                # "不是右键"
              }
              frame True {
                w1005 = TRUE  # T
                w1011 = TRUE  # T
                # "右键"
                n499 = property class="多列列表框 (严格)" props=["ContentRectPosTop", "Value"](reference=w1010) -> ("Value"=w1007:i32[])  [unwired: 1 in, 3 out]
                n500 = global read "全局变量-35点监测.vi" "最大探头数"() -> (w1001:i32)
                n501 = local read "报警记录数"() -> (w1000:i32)
                n502 = Unbundle By Name(w1008) -> ("Row"=w999:i32)
                n503 = Select(t=w1001, s=w1002, f=w1000) -> (s? t:f=w997:i32)
                n504 = Increment(x=w999) -> (x+1=w998:i32)
                n505 = Less Or Equal? "点在有效信息行内？"(x=w998, y=w997) -> (x <= y?=w995:bool)
                n506 = Empty Array? "空数组？"(array=w1007) -> (empty?=w1006:bool)
                n507 = for {
                  tunnel: w1007 -> [w1028] mode=indexing
                  shift-right: [w1025] -> w1004
                  shift-left: w1011 -> [w1026]
                  tunnel: w999 -> [w1024]
                  tunnel: w995 -> [w1022]
                  stop <- w1025 continue-if-true
                  # "在选中项之外？"
                  n508 = Not Equal?(x=w1028, y=w1024) -> (x != y?=w1027:bool)
                  n509 = Greater Or Equal To 0?(x=w1024) -> (x >= 0?=w1023:bool)
                  n510 = Compound Arithmetic op=AND(w1027, w1026, w1023, w1022) -> (w1025:bool)
                }
                n511 = Build Array(w999) -> (w1009:i32[])
                n512 = Select(t=w1005, s=w1006, f=w1004) -> (s? t:f=w1003:bool)
                n513 = And(x=w1003, y=w995) -> (x .and. y?=w996:bool)
                n514 = case shown="假" w996 {
                  tunnel: w1009 -> [_ w1019]
                  tunnel: w1002 -> [w1012 w1018]
                  tunnel: w995 -> [w1013 _]
                  frame False {
                    # "在选中项之中，不赋值"
                    n515 = case shown="假" w1013 {
                      tunnel: w1012 -> [w1015 _]
                      frame False {
                        # "点在不可选行，清空"
                        n516 = case shown="真" w1015 {
                          tunnel: i32[] [] ("实时数据列表") -> [w1016 w1017]
                          frame False {
                            n517 = local write "报警记录列表"(w1016) -> ()
                          }
                          frame True {
                            n518 = local write "实时数据列表"(w1017) -> ()
                          }
                        }
                      }
                      frame True {
                      }
                    }
                  }
                  frame True {
                    # "在选中项之外，赋值"
                    n519 = case shown="假" w1018 {
                      tunnel: w1019 -> [w1020 w1021]
                      frame False {
                        n520 = local write "报警记录列表"(w1020) -> ()
                      }
                      frame True {
                        n521 = local write "实时数据列表"(w1021) -> ()
                      }
                    }
                  }
                }
              }
            }
          }
          event "监测模式": Value Change {
            # "判断是否可以切换到监测模式\n跳过“禁用项”。"
            # "切换到 方格 样式 界面"
            n522 = event-data() -> ()  [unwired: 1 in, 6 out]
            n523 = local read "探头启用状态？"() -> (w1029:bool[])
            n524 = global read "全局变量-35点监测.vi" "最大探头数"() -> (w1031:i32)
            n525 = local read "探头信息"() -> (w1035:string[])
            n526 = local read "限值"() -> (w1036:T4)
            n527 = local write "监测模式"(FALSE ("监测模式")) -> ()
            n528 = for {
              N: w1031 -> [_]
              tunnel: w1035 -> [w1043] mode=indexing
              tunnel: [w1037] -> w1032
              tunnel: w1029 -> [w1040] mode=indexing
              stop <- w1037 stop-if-true
              w1039 = FALSE  # f
              # "查找未命名项"
              n529 = Empty String/Path?(string/path=w1043) -> (empty?=w1042:bool)
              n530 = White Space?(1:w1043) -> (0:w1041:bool)
              n531 = Or(x=w1042, y=w1041) -> (x .or. y?=w1038:bool)
              n532 = Select "启用的？"(t=w1038, s=w1040, f=w1039) -> (s? t:f=w1037:bool)
            }
            n533 = for {
              N: w1031 -> [_]
              tunnel: w1036 -> [w1108] mode=indexing
              tunnel: [w1102] -> w1033
              tunnel: w1029 -> [w1105] mode=indexing
              stop <- w1102 stop-if-true
              w1103 = FALSE  # f
              # "查找是否有未设置的报警值"
              n534 = Unbundle By Name(w1108) -> ("限值1"=w1107:dbl)
              n535 = Equal?(x=w1107, y=inf) -> (x = y?=w1104:bool)
              n536 = Select "启用的？"(t=w1104, s=w1105, f=w1103) -> (s? t:f=w1102:bool)
            }
            n537 = Or(x=w1033, y=w1032) -> (x .or. y?=w1034:bool)
            n538 = case shown="假" w1034 {
              tunnel: w1031 -> [w1045 _]
              tunnel: w1033 -> [_ w1101]
              tunnel: w1032 -> [_ w1100]
              frame False {
                # "没有 未设置报警值 或 未命名 的探头"
                n539 = case shown="0..2, 默认" w1045 {
                  tunnel: [w1074 w1076 w1078 w1080 w1082 w1084 w1086 w1088 w1090 w1092] -> w1051
                  tunnel: [cluster{"min":i32, "max":i32} {"min"=1, "max"=2} ("监测数量限值") cluster{"min":i32, "max":i32} {"min"=3, "max"=4} ("监测数量限值") cluster{"min":i32, "max":i32} {"min"=5, "max"=6} ("监测数量限值") cluster{"min":i32, "max":i32} {"min"=7, "max"=8} ("监测数量限值") cluster{"min":i32, "max":i32} {"min"=9, "max"=12} ("监测数量限值") cluster{"min":i32, "max":i32} {"min"=13, "max"=16} ("监测数量限值") cluster{"min":i32, "max":i32} {"min"=17, "max"=20} ("监测数量限值") cluster{"min":i32, "max":i32} {"min"=21, "max"=24} ("监测数量限值") cluster{"min":i32, "max":i32} {"min"=25, "max"=28} ("监测数量限值") cluster{"min":i32, "max":i32} {"min"=29, "max"=32} ("监测数量限值")] -> w1044
                  frame 0..2, Default {
                    n540 = vi-ref "探头窗口-2.vi"() -> (w1074:refnum<vi>)
                  }
                  frame 3, 4 {
                    n541 = vi-ref "探头窗口-4.vi"() -> (w1076:refnum<vi>)
                  }
                  frame 5, 6 {
                    n542 = vi-ref "探头窗口-6.vi"() -> (w1078:refnum<vi>)
                  }
                  frame 7, 8 {
                    n543 = vi-ref "探头窗口-8.vi"() -> (w1080:refnum<vi>)
                  }
                  frame 9..12 {
                    n544 = vi-ref "探头窗口-12.vi"() -> (w1082:refnum<vi>)
                  }
                  frame 13..16 {
                    n545 = vi-ref "探头窗口-16.vi"() -> (w1084:refnum<vi>)
                  }
                  frame 17..20 {
                    n546 = vi-ref "探头窗口-20.vi"() -> (w1086:refnum<vi>)
                  }
                  frame 21..24 {
                    n547 = vi-ref "探头窗口-24-4列.vi"() -> (w1088:refnum<vi>)
                  }
                  frame 25..28 {
                    n548 = vi-ref "探头窗口-28-4列.vi"() -> (w1090:refnum<vi>)
                  }
                  frame 29..32 {
                    n549 = vi-ref "探头窗口-32-4列.vi"() -> (w1092:refnum<vi>)
                  }
                }
                "监测数量限值" <- w1044
                n550 = invoke on="运行VI" class="VI" method="Run VI"(reference=w1051, "Wait until done"=FALSE ("结束前等待"), "Auto Dispose Ref"=TRUE ("自动销毁引用")) -> (reference out=w1055:refnum<vi>, error out=w1056:errorcluster)  [unwired: 2 in, 3 out]
                n551 = disable-structure shown="启用" {
                  disable-tunnel: w1056 -> [w1070 w1071]
                  disable-tunnel: w1055 -> [w1068 w1072]
                  disable-tunnel: [w1063 w1071] -> w1052
                  disable-tunnel: [w1062 w1072] -> w1046
                  frame Disabled {
                    # "无顶层框架时候，启用"
                    n552 = invoke on="打开前面板" class="VI" method="FP.Open"(reference=w1068, error in=w1070, "Activate"=TRUE ("激活？"), "State"=T7."Maximized" ("状态")) -> (reference out=w1062:refnum<vi>, error out=w1065:errorcluster)  [unwired: 1 in, 3 out]
                    n553 = control-ref of="本VI"() -> (w1066:refnum<vi>)
                    n554 = property class="VI"(reference=w1066, error in=w1065, "FP.State"=T7."Minimized" ("前面板窗口:状态")) -> (error out=w1063:errorcluster)  [unwired: 1 out]
                  }
                  frame Enabled {
                    # "有顶层框架时启用"
                  }
                }
                n555 = call <vilib>:"Clear Errors.vi"("error in (no error)"=w1052) -> ()  [unwired: 5 in, 2 out]
                n556 = stacked-sequence {
                  tunnel: w1046 -> [w1057 _]
                  frame #0 {
                    n557 = call "通过控件名获取控件引用.vi"("控件名数组"=string[] ["停止信号"], "VI引用"=w1057) -> ("控件引用输出"=w1058:refnum<vi>[])  [unwired: 7 in, 2 out]
                    n558 = Index Array(array=w1058) -> (element=→"监-停止信号":refnum<vi>)  [unwired: 1 in]
                    "监测窗口VI" <- w1057
                  }
                  frame #1 {
                    w1061 = FALSE  # F
                    n559 = property on="更新列表？" class="Bool (严格)"("Val(Sgnl)"=w1061) -> ()  [unwired: 2 in, 2 out]
                  }
                }
                n560 = call "通过控件名获取控件引用.vi"("控件名数组"=string[] ["更新数据", "更新数据？"], "VI引用"=w1046) -> ("控件引用输出"=w1049:refnum<vi>[])  [unwired: 7 in, 2 out]
                n561 = Index Array(array=w1049) -> (element #1=→"引用-更新数据簇":refnum<vi>, element #2=→"引用-更新数据信号":refnum<vi>)  [unwired: 2 in]
              }
              frame True {
                w1099 = ""
                # "存在未设置报警值的探头，弹窗提示"
                n562 = Select(t="\n报警限值", s=w1101, f=w1099) -> (s? t:f=w1096:string)
                n563 = Select(t="\n设备名称", s=w1100, f=w1099) -> (s? t:f=w1095:string)
                n564 = Concatenate Strings("存在待设置项：\n", w1096, w1095) -> (w1093:string)
                n565 = call "存在待设置项"("Message"=w1093) -> ()  [unwired: 9 in, 2 out]
              }
            }
          }
          event "查看报表": Value Change {
            # "打开文件路径"
            n566 = event-data() -> ()  [unwired: 1 in, 6 out]
            n567 = call "路径查找创建-报警记录清单.vi"() -> ("报表文件夹"=w1109:path)  [unwired: 8 in, 11 out]
            n568 = call "cmd打开文件夹.vi"("文件路径"=w1109) -> ()  [unwired: 10 in, 1 out]
          }
          event "帮助": Value Change {
            n569 = event-data() -> ()  [unwired: 1 in, 6 out]
            n570 = call "路径查找创建-报警记录清单.vi"() -> ("帮助文档路径"=w1110:path)  [unwired: 8 in, 11 out]
            n571 = call "cmd打开文件.vi"("文件路径"=w1110) -> ()  [unwired: 10 in, 1 out]
          }
          event "公司LOGO与型号": Mouse Up {
            n572 = event-data() -> ("Mods.Double Click"=w1111:bool)  [unwired: 1 in, 7 out]
            n573 = case shown="真" w1111 {
              frame False {
              }
              frame True {
                # "双击打开网址"
              }
            }
          }
          event "状态栏-项名[]": Value Change {
            # "在其他VI里改变值，在此处处理"
            n574 = event-data() -> ()  [unwired: 1 in, 6 out]
            n575 = local read "状态类型"() -> (w1115:enum16{"全部", "报警", "通信", "设置"})
            n576 = Array Size(array="状态栏-项名[]") -> (size(s)=w1118:i32)
            n577 = Decrement(x=w1118) -> (x-1=w1119:i32)
            n578 = Index Array "获取新增项"(array="状态栏-项名[]", index=w1119) -> (element=w1114:string)
            n579 = Equal To 0?(x=w1115) -> (x = 0?=w1116:bool)
            n580 = case shown="真" w1116 {
              tunnel: w1115 -> [w1135 _]
              tunnel: w1114 -> [w1133 _]
              tunnel: [w1130 w1136] -> w1112
              frame False {
                # "按关键词过滤"
                n581 = property on="状态类型" class="Enum (严格)"() -> ("Strings []"=w1129:string[])  [unwired: 2 in, 2 out]
                n582 = Index Array "当前关键词"(array=w1129, index=w1135) -> (element=w1132:string)
                n583 = Match Pattern(string=w1133, regular expression=w1132, offset (0)=20 ("偏移量(0)")) -> (offset past match=w1131:i32)  [unwired: 3 out]
                n584 = Greater Or Equal To 0?(x=w1131) -> (x >= 0?=w1130:bool)
              }
              frame True {
                w1136 = TRUE  # T
                # "显示全部"
              }
            }
            n585 = control-ref of="状态栏"() -> (w1113:refnum<vi>)
            n586 = case shown="真" w1112 {
              tunnel: w1113 -> [_ w1128]
              tunnel: w1114 -> [_ w1124]
              frame False {
                # "未匹配，不添加"
              }
              frame True {
                # "添加，并置为左上可见"
                n587 = call-poly "多态-列表插入项名.vi"("项名"=w1124, "限定行数(500)"=u32 500, "LstBox引用句柄"=w1128) -> ("引用输出"=w1127:refnum<vi>)  [unwired: 8 in]
                n588 = property class="LstBox"(reference=w1127) -> (reference out=w1126:refnum<vi>, error out=w1125:errorcluster, "Item Names"=w1123:string[])  [unwired: 1 in]
                n589 = Array Size(array=w1123) -> (size(s)=w1122:i32)
                n590 = Decrement(x=w1122) -> (x-1=w1121:i32)
                n591 = property class="LstBox"(reference=w1126, error in=w1125, "Top Row"=w1121) -> ()  [unwired: 2 out]
              }
            }
          }
          event "状态类型": Value Change {
            n592 = event-data() -> ()  [unwired: 1 in, 6 out]
            n593 = local read "状态栏-项名[]"() -> (w1144:string[])
            n594 = Equal To 0?(x="状态类型") -> (x = 0?=w1146:bool)
            n595 = case shown="假" w1146 {
              tunnel: "状态类型" -> [w1154 _]
              tunnel: w1144 -> [w1153 w1166]
              tunnel: [w1151 w1166] -> w1138
              frame False {
                # "按关键词过滤"
                n596 = property on="状态类型" class="Enum (严格)"() -> ("Strings []"=w1150:string[])  [unwired: 2 in, 2 out]
                n597 = Index Array "当前关键词"(array=w1150, index=w1154) -> (element=w1149:string)
                n598 = Concatenate Strings(w1149, " 】 ") -> (w1147:string)
                n599 = for {
                  tunnel: w1153 -> [w1156] mode=indexing
                  tunnel: w1147 -> [w1159]
                  shift-right: [w1155] -> w1151
                  shift-left: string[] [] ("项名") -> [w1157]
                  # "过滤关键词"
                  n600 = Match Pattern(string=w1156, regular expression=w1159, offset (0)=20 ("偏移量(0)")) -> (offset past match=w1161:i32)  [unwired: 3 out]
                  n601 = Greater Or Equal To 0?(x=w1161) -> (x >= 0?=w1158:bool)
                  n602 = case shown="真" w1158 {
                    tunnel: w1157 -> [w1162 w1165]
                    tunnel: w1156 -> [_ w1164]
                    tunnel: [w1162 w1163] -> w1155
                    frame False {
                      # "不匹配"
                    }
                    frame True {
                      # "匹配"
                      n603 = Insert Into Array(array=w1165, new element=w1164) -> (w1163:string[])  [unwired: 1 in]
                    }
                  }
                }
              }
              frame True {
                # "显示全部"
              }
            }
            n604 = Array Size(array=w1138) -> (size(s)=w1139:i32)
            n605 = Decrement(x=w1139) -> (x-1=w1141:i32)
            n606 = control-ref of="状态栏"() -> (w1137:refnum<vi>)
            n607 = Less Than 0?(x=w1141) -> (x < 0?=w1140:bool)
            n608 = Select(t=0, s=w1140, f=w1141) -> (s? t:f=w1143:i32)
            n609 = property class="LstBox (严格)"(reference=w1137, "Item Names"=w1138, "Top Row"=w1143) -> ()  [unwired: 1 in, 2 out]
          }
          event "清除状态": Value Change {
            n610 = event-data() -> ()  [unwired: 1 in, 6 out]
            n611 = control-ref of="状态栏"() -> (w1171:refnum<vi>)
            n612 = property class="LstBox (严格)"(reference=w1171, "Item Names"=string[] [] ("项名")) -> ()  [unwired: 1 in, 2 out]
            n613 = local read "状态栏-项名[]"() -> (w1169:string[])
            n614 = local read "状态类型"() -> (w1167:enum16{"全部", "报警", "通信", "设置"})
            n615 = Equal To 0?(x=w1167) -> (x = 0?=w1170:bool)
            n616 = case shown="假" w1170 {
              tunnel: w1167 -> [w1178 _]
              tunnel: w1169 -> [w1177 _]
              tunnel: [w1174 string[] [] ("项名")] -> w1168
              frame False {
                # "关键词以外的，保留"
                n617 = property on="状态类型" class="Enum (严格)"() -> ("Strings []"=w1173:string[])  [unwired: 2 in, 2 out]
                n618 = Index Array "当前关键词"(array=w1173, index=w1178) -> (element=w1176:string)
                n619 = for {
                  tunnel: w1177 -> [w1180] mode=indexing
                  tunnel: w1176 -> [w1183]
                  shift-right: [w1179] -> w1174
                  shift-left: string[] [] ("项名") -> [w1181]
                  # "过滤关键词"
                  n620 = Match Pattern(string=w1180, regular expression=w1183, offset (0)=20 ("偏移量(0)")) -> (offset past match=w1185:i32)  [unwired: 3 out]
                  n621 = Less Than 0? "不匹配？"(x=w1185) -> (x < 0?=w1182:bool)
                  n622 = case shown="假" w1182 {
                    tunnel: w1181 -> [w1186 w1189]
                    tunnel: w1180 -> [_ w1188]
                    tunnel: [w1186 w1187] -> w1179
                    frame False {
                      # "匹配\n不保留"
                    }
                    frame True {
                      # "不匹配\n保留"
                      n623 = Insert Into Array(array=w1189, new element=w1188) -> (w1187:string[])  [unwired: 1 in]
                    }
                  }
                }
              }
              frame True {
                # "全部清除"
              }
            }
            n624 = local write "状态栏-项名[]"(w1168) -> ()
          }
          event "更新列表？": Value Change {
            # "从方格窗口切换回来"
            n625 = event-data() -> ()  [unwired: 1 in, 6 out]
            n626 = disable-structure shown="启用" {
              frame Disabled {
                # "无顶层框架时候，开启"
                n627 = local read "监测窗口VI"() -> (w1195:refnum<vi>)
                n628 = invoke class="VI" method="FP.Close"(reference=w1195) -> (error out=w1192:errorcluster)  [unwired: 2 in, 2 out]
                n629 = control-ref of="本VI"() -> (w1193:refnum<vi>)
                n630 = property class="VI"(reference=w1193, error in=w1192, "FP.State"=T7."Standard" ("前面板窗口:状态")) -> (error out=w1191:errorcluster)  [unwired: 1 out]
                n631 = call <vilib>:"Clear Errors.vi"("error in (no error)"=w1191) -> ()  [unwired: 5 in, 2 out]
              }
              frame Enabled {
              }
            }
          }
          event "实时数据列表": Double Click {
            # "使 双击 可寻找到对应的列，并触发菜单处理事件，使打开修改弹窗"
            n632 = event-data() -> ("CtlRef"=w1203:refnum<vi>, "Coords"=w1215:T31, "PlatMods"=w1206:T33)  [unwired: 1 in, 6 out]
            n633 = property class="MCListbox (严格)"(reference=w1203) -> ("Value"=w1212:i32[])  [unwired: 1 in, 2 out]
            n634 = invoke class="多列列表框 (严格)" method="Point To Row Column"(reference=w1203, "Point"=w1215) -> ("CellPosition"=w1216:T5)  [unwired: 5 in, 6 out]
            n635 = property class="MCListbox (严格)"(reference=w1203) -> ("ItemNames"=w1202:string[][])  [unwired: 1 in, 2 out]
            n636 = Unbundle By Name(w1206) -> ("Shift"=w1208:bool, "Ctrl"=w1207:bool)
            n637 = local read "探头启用状态？"() -> (w1210:bool[])
            n638 = Not Or(1:w1207, 2:w1208) -> (0:w1204:bool)
            n639 = Array Size(array=w1202) -> (size(s)=w1201:i32[])
            n640 = Unbundle By Name(w1216) -> ("Row"=w1196:i32, "Column"=w1214:i32)
            n641 = Index Array(array=w1212) -> (element=w1211:i32)  [unwired: 1 in]
            n642 = Index Array(array=w1201) -> (element=w1200:i32)  [unwired: 1 in]
            n643 = Index Array(array=w1210, index=w1211) -> (element=w1209:bool)
            n644 = Decrement(x=w1200) -> (x-1=w1198:i32)
            n645 = Greater Or Equal?(x=w1198, y=w1196) -> (x >= y?=w1197:bool)
            n646 = Greater Or Equal To 0?(x=w1196) -> (x >= 0?=w1213:bool)
            n647 = And(x=w1197, y=w1213) -> (x .and. y?=w1199:bool)
            n648 = And(x=w1199, y=w1204) -> (x .and. y?=w1205:bool)
            n649 = case shown="真" w1205 {
              tunnel: w1203 -> [_ w1220]
              tunnel: w1214 -> [_ w1219]
              tunnel: w1209 -> [_ w1218]
              tunnel: w1196 -> [_ w1217]
              frame False {
                # "无效行"
              }
              frame True {
                # "有效行"
                n650 = case shown="0..2, 4..8" w1219 {
                  tunnel: w1219 -> [_ w1226]
                  tunnel: w1220 -> [_ w1225]
                  tunnel: w1218 -> [_ w1223]
                  tunnel: w1217 -> [_ w1221]
                  frame -1, Default {
                    # "不触发菜单事件"
                  }
                  frame 0..2, 4..8 {
                    # "指定列内才可以触发菜单事件"
                    n651 = case shown="8" w1226 {
                      tunnel: [T16."交换探头地址" ("启用") w1232 T17."修改探头信息" ("值(信号)") T17."修改报警限值" ("值(信号)") T18."累积清零" ("值(信号)") T18."累积报警阈值" ("值(信号)") T3."探头报警方式" ("菜单项-实时列表")] -> w1224
                      tunnel: w1225 -> [_ _ _ _ _ _ _]
                      tunnel: w1223 -> [w1228 w1231 _ w1240 _ _ w1256]
                      tunnel: [w1228 w1230 w1238 w1240 w1242 w1249 w1256] -> w1222
                      tunnel: w1221 -> [_ _ _ _ w1246 w1250 _]
                      frame 0, Default {
                        # "探头列，交换探头"
                      }
                      frame 1 {
                        # "禁用“禁用”、“启用”探头功能\n因为这个功能并没有什么实用价值"
                        # "状态列，禁用或启用探头"
                        n652 = disable-structure shown="禁用" {
                          disable-tunnel: [w1237 _] -> w1232
                          disable-tunnel: w1231 -> [w1234 _]
                          disable-tunnel: [w1233 _] -> w1230
                          frame Disabled {
                            w1233 = TRUE  # T
                            w1235 = T17."启用"  # 启用
                            w1236 = T17."禁用"  # 禁用
                            n653 = Select(t=w1236, s=w1234, f=w1235) -> (s? t:f=w1237:T17)
                          }
                          frame Enabled {
                          }
                        }
                      }
                      frame 2 {
                        w1238 = TRUE  # T
                        # "探头信息列，修改探头信息"
                      }
                      frame 4, 5 {
                        # "一级限值列"
                      }
                      frame 6 {
                        # "清零累积"
                        n654 = local read "累积剂量"() -> (w1244:T2)
                        n655 = local read "探头信息"() -> (w1247:string[])
                        n656 = Index Array(array=w1247, index=w1246) -> (element=w1245:string)
                        n657 = call "查找匹配累积剂量.vi"("探头名称"=w1245, "累积剂量"=w1244) -> ("匹配的累积剂量"=w1243:T20)  [unwired: 7 in, 2 out]
                        n658 = Unbundle By Name(w1243) -> ("启用累积？"=w1242:bool)
                      }
                      frame 7 {
                        # "设置累积报警阈值"
                        n659 = local read "累积剂量"() -> (w1252:T2)
                        n660 = local read "探头信息"() -> (w1254:string[])
                        n661 = Index Array(array=w1254, index=w1250) -> (element=w1253:string)
                        n662 = call "查找匹配累积剂量.vi"("探头名称"=w1253, "累积剂量"=w1252) -> ("匹配的累积剂量"=w1251:T20)  [unwired: 7 in, 2 out]
                        n663 = Unbundle By Name(w1251) -> ("启用累积？"=w1249:bool)
                      }
                      frame 8 {
                        # "探头报警方式"
                      }
                    }
                    n664 = case shown="真" w1222 {
                      tunnel: w1224 -> [_ w1227]
                      frame False {
                      }
                      frame True {
                        # "是否触发"
                        n665 = property on="菜单项-实时列表" class="Enum (严格)"("Val(Sgnl)"=w1227) -> ()  [unwired: 2 in, 2 out]
                      }
                    }
                  }
                }
              }
            }
          }
          event "报警记录列表": Double Click {
            # "历史数据列表双击，删除记录提示"
            n666 = event-data() -> ("CtlRef"=w1264:refnum<vi>, "Coords"=w1272:T31, "PlatMods"=w1269:T33)  [unwired: 1 in, 6 out]
            n667 = property class="MCListbox (严格)"(reference=w1264) -> ("ItemNames"=w1266:string[][])  [unwired: 1 in, 2 out]
            n668 = invoke class="多列列表框 (严格)" method="Point To Row Column"(reference=w1264, "Point"=w1272) -> ("CellPosition"=w1273:T5)  [unwired: 5 in, 6 out]
            "点到行列-报警记录" <- w1273
            n669 = Unbundle By Name(w1269) -> ("Shift"=w1270:bool, "Ctrl"=w1271:bool)
            n670 = Not Or(1:w1271, 2:w1270) -> (0:w1267:bool)
            n671 = Array Size(array=w1266) -> (size(s)=w1265:i32[])
            n672 = Unbundle By Name(w1273) -> ("Row"=w1261:i32)  [unwired: 1 out]
            n673 = Index Array(array=w1265) -> (element=w1263:i32)  [unwired: 1 in]
            n674 = Decrement(x=w1263) -> (x-1=w1262:i32)
            n675 = Greater Or Equal?(x=w1262, y=w1261) -> (x >= y?=w1260:bool)
            n676 = Greater Or Equal To 0?(x=w1261) -> (x >= 0?=w1259:bool)
            n677 = And(x=w1260, y=w1259) -> (x .and. y?=w1258:bool)
            n678 = And(x=w1258, y=w1267) -> (x .and. y?=w1268:bool)
            n679 = case shown="真" w1268 {
              frame False {
                # "无效行"
              }
              frame True {
                # "有效行"
                n680 = property on="菜单项-报警列表" class="Enum (严格)"("Val(Sgnl)"=enum16{"刷新", "预览并生成报表", "删除记录"}."预览并生成报表" ("菜单项-报警列表")) -> ()  [unwired: 2 in, 2 out]
              }
            }
          }
          event "实时数据列表": Shortcut Menu Activation? {
            w1277 = "禁用累积" ("项名称")
            w1278 = "启用累积" ("项名称")
            w1291 = "累积设置" ("项名称")
            w1287 = "累积报警阈值" ("项名称")
            w1288 = "累积清零" ("项名称")
            w1296 = FALSE  # F
            w1297 = FALSE  # F
            w1298 = "备注信息" ("项名称")
            w1302 = "修改报警限值" ("项名称")
            w1314 = "交换探头地址" ("项名称")
            w1311 = "禁用" ("项名称")
            w1310 = "启用" ("项名称")
            # "禁用“禁用”、“启用”探头功能\n因为这个功能并没有什么实用价值"
            # "启用"
            # "禁用"
            # "配置菜单项-实时列表"
            n681 = event-data() -> ("CtlRef"=w1306:refnum<vi>, "MenuRef"=w1292:refnum<k9>)  [unwired: 1 in, 5 out]
            n682 = property class="多列列表框 (严格)"(reference=w1306) -> ("Value"=w1293:i32[])  [unwired: 1 in, 2 out]
            n683 = Array Size(array=w1293) -> (size(s)=w1315:i32)
            n684 = Equal?(x=w1315, y=1) -> (x = y?=w1294:bool)
            n685 = case shown="真" w1294 {
              tunnel: w1293 -> [_ w1326]
              tunnel: [w1318 w1320] -> w1290
              tunnel: [w1318 w1319] -> w1276
              frame False {
                w1318 = TRUE  # T
                # "多选 全部启用"
                # "多选"
              }
              frame True {
                # "单项选择"
                n686 = local read "探头信息"() -> (w1325:string[])
                n687 = local read "累积剂量"() -> (w1323:T2)
                n688 = Index Array(array=w1326) -> (element=w1324:i32)  [unwired: 1 in]
                n689 = Index Array(array=w1325, index=w1324) -> (element=w1322:string)
                n690 = call "查找匹配累积剂量.vi"("探头名称"=w1322, "累积剂量"=w1323) -> ("匹配？"=w1320:bool, "匹配的累积剂量"=w1321:T20)  [unwired: 7 in, 1 out]
                n691 = Unbundle By Name(w1321) -> ("启用累积？"=w1319:bool)
              }
            }
            n692 = case shown="真" w1294 {
              tunnel: [w1330 w1331] -> _
              tunnel: [w1330 w1334] -> _
              tunnel: w1293 -> [_ w1333]
              tunnel: [w1329 w1331] -> w1300
              frame False {
                w1330 = TRUE  # T
                # "多线选择"
                n693 = Not(x=w1330) -> (.not. x?=w1329:bool)
              }
              frame True {
                # "单项选择"
                n694 = local read "探头启用状态？"() -> (w1335:bool[])
                n695 = Index Array(array=w1333) -> (element=w1332:i32)  [unwired: 1 in]
                n696 = Index Array(array=w1335, index=w1332) -> (element=w1331:bool)
                n697 = Not(x=w1331) -> (.not. x?=w1334:bool)
              }
            }
            n698 = Set Menu Item Info(7:w1310, 9:w1296, 10:w1310, 11:w1292) -> (0:w1308:errorcluster, 3:w1309:refnum<k9>)  [unwired: 3 in]
            n699 = Set Menu Item Info(7:w1291, 9:w1290, 10:w1291, 11:w1292) -> (0:w1284:errorcluster, 3:w1285:refnum<k9>)  [unwired: 3 in]
            n700 = Set Menu Item Info(7:w1311, 8:w1308, 9:w1296, 10:w1311, 11:w1309) -> (0:w1312:errorcluster, 3:w1313:refnum<k9>)  [unwired: 2 in]
            n701 = Set Menu Item Info(7:w1314, 8:w1312, 9:w1300, 10:w1314, 11:w1313) -> (0:w1304:errorcluster, 3:w1303:refnum<k9>)  [unwired: 2 in]
            n702 = Set Menu Item Info(7:w1288, 8:w1284, 9:w1276, 10:w1288, 11:w1285) -> (0:w1286:errorcluster, 3:w1289:refnum<k9>)  [unwired: 2 in]
            n703 = disable-structure shown="禁用" {
              disable-tunnel: [w1327 w1328] -> w1301
              disable-tunnel: w1300 -> [w1327 _]
              frame Disabled {
              }
              frame Enabled {
                w1328 = TRUE  # T
              }
            }
            n704 = Set Menu Item Info(7:w1287, 8:w1286, 9:w1276, 10:w1287, 11:w1289) -> (0:w1283:errorcluster, 3:w1280:refnum<k9>)  [unwired: 2 in]
            n705 = Set Menu Item Info(7:w1302, 8:w1304, 9:w1301, 10:w1302, 11:w1303) -> (0:w1295:errorcluster, 3:w1299:refnum<k9>)  [unwired: 2 in]
            n706 = Not(x=w1276) -> (.not. x?=w1275:bool)
            n707 = Set Menu Item Info(7:w1278, 8:w1283, 9:w1275, 10:w1278, 11:w1280) -> (0:w1282:errorcluster, 3:w1279:refnum<k9>)  [unwired: 2 in]
            n708 = Set Menu Item Info(7:w1298, 8:w1295, 9:w1297, 10:w1298, 11:w1299) -> ()  [unwired: 2 in, 2 out]
            n709 = local read "暂停发送"() -> (w1317:bool)
            n710 = Empty Array?(array=w1293) -> (empty?=w1316:bool)
            n711 = Set Menu Item Info(7:w1277, 8:w1282, 9:w1276, 10:w1277, 11:w1279) -> (0:w1281:errorcluster)  [unwired: 2 in, 1 out]
            n712 = Or(x=w1316, y=w1317) -> (x .or. y?=w1305:bool)
            n713 = call <vilib>:"Clear Errors.vi"("error in (no error)"=w1281) -> ()  [unwired: 5 in, 2 out]
            n714 = event-data("Discard?"=w1305) -> ()  [unwired: 1 in, 1 out]
          }
          event "报警记录列表": Shortcut Menu Activation? {
            w1340 = "预览并生成报表" ("项标识符")
            # "菜单项启用状态，仅单选可预览"
            n715 = event-data() -> ("CtlRef"=w1345:refnum<vi>, "MenuRef"=w1337:refnum<k9>)  [unwired: 1 in, 5 out]
            n716 = property class="多列列表框 (严格)"(reference=w1345) -> ("Value"=w1336:i32[])  [unwired: 1 in, 2 out]
            n717 = Array Size(array=w1336) -> (size(s)=w1338:i32)
            n718 = Equal? "单项？"(x=w1338, y=1) -> (x = y?=w1341:bool)
            n719 = Set Menu Item Info(7:w1340, 9:w1341, 10:w1340, 11:w1337) -> ()  [unwired: 3 in, 2 out]
            n720 = local read "暂停发送"() -> (w1344:bool)
            n721 = Empty Array?(array=w1336) -> (empty?=w1343:bool)
            n722 = Or(x=w1343, y=w1344) -> (x .or. y?=w1342:bool)
            n723 = event-data("Discard?"=w1342) -> ()  [unwired: 1 in, 1 out]
          }
          event "实时数据列表": Shortcut Menu Selection (User) {
            # "实时列表-菜单选择"
            n724 = event-data() -> ("ItemTag"=w1347:string)  [unwired: 1 in, 7 out]
            n725 = property on="菜单项-实时列表" class="Enum (严格)"() -> ("Strings []"=w1348:string[])  [unwired: 2 in, 2 out]
            n726 = Search 1D Array(1D array=w1348, element=w1347) -> (index of element=w1346:i32)  [unwired: 1 in]
            n727 = property on="菜单项-实时列表" class="Enum (严格)"("Val(Sgnl)"=w1346) -> ()  [unwired: 2 in, 2 out]
          }
          event "报警记录列表": Shortcut Menu Selection (User) {
            # "处理报警列表菜单事件"
            n728 = event-data() -> ("ItemTag"=w1350:string)  [unwired: 1 in, 7 out]
            n729 = property on="菜单项-报警列表" class="Enum (严格)"() -> ("Strings []"=w1351:string[])  [unwired: 2 in, 2 out]
            n730 = Search 1D Array(1D array=w1351, element=w1350) -> (index of element=w1349:i32)  [unwired: 1 in]
            n731 = property on="菜单项-报警列表" class="Enum (严格)"("Val(Sgnl)"=w1349) -> ()  [unwired: 2 in, 2 out]
          }
          event "菜单项-实时列表": Value Change {
            # "实时列表，菜单事件处理"
            n732 = event-data() -> ("CtlRef"=w1354:refnum<vi>)  [unwired: 1 in, 5 out]
            n733 = local read "点到行列-实时列表"() -> (w1352:T5)
            n734 = local read "暂停发送"() -> (w1353:bool)
            n735 = case shown="假" w1353 {
              tunnel: w1354 -> [w1362 _]
              tunnel: w1352 -> [w1358 _]
              frame False {
                # "非暂停发送状态，可以产生菜单事件"
                n736 = property class="Enum (严格)"(reference=w1362) -> ("RingText.Text"=w1361:string)  [unwired: 1 in, 2 out]
                n737 = local read "探头信息"() -> (w1357:string[])
                n738 = global read "全局变量-35点监测.vi" "最大探头数"() -> (w1356:i32)
                n739 = local read "实时数据列表"() -> (w1360:i32[])
                n740 = local read "探头地址"() -> (w1359:i32[])
                n741 = Array Subset(array=w1357, length=w1356) -> (w1355:string[])  [unwired: 1 in]
                n742 = case shown="\"修改报警限值\"" w1361 {
                  tunnel: w1360 -> [w1373 w1393 w1404 _ w1456 _ _ w1475 w1489 w1539 w1551 _ w1595]
                  tunnel: w1359 -> [_ _ w1405 _ w1457 _ _ w1474 w1488 _ _ _ _]
                  tunnel: w1358 -> [_ _ _ w1441 _ _ _ _ _ _ _ _ _]
                  tunnel: w1355 -> [_ _ _ _ _ _ _ _ w1487 w1538 w1550 w1578 _]
                  frame "禁用" {
                    w1371 = inf
                    # "禁用探头"
                    n743 = local read "探头启用状态？"() -> (w1374:bool[])
                    n744 = local read "限值"() -> (w1370:T4)
                    n745 = Bundle(cluster=T15 {"限值1"=0.0, "限值2"=0.0, "探头限值"=enum."一级限值"} ("探头限值簇"), "限值1"=w1371, "限值2"=w1371, "探头限值"=enum16{"一级限值", "二级限值"}."一级限值") -> (w1369:T15)
                    n746 = for {
                      tunnel: w1373 -> [w1380] mode=indexing
                      shift-right: [w1386] -> w1372
                      shift-left: w1374 -> [w1387]
                      shift-right: [w1384] -> w1368
                      shift-left: w1370 -> [w1385]
                      tunnel: w1369 -> [w1383]
                      shift-right: [w1377] -> w1365
                      shift-left: "禁用探头" ("字符串") -> [w1378]
                      w1388 = FALSE  # F
                      n747 = Replace Array Subset "限值无穷大"(array=w1385, new element=w1383, index=w1380) -> (w1384:T4)
                      n748 = Replace Array Subset "更新 探头启用状态"(array=w1387, new element=w1388, index=w1380) -> (w1386:bool[])
                      n749 = Increment(x=w1380) -> (x+1=w1379:i32)
                      n750 = Number To Decimal String(number=w1379) -> (decimal integer string=w1381:string)  [unwired: 1 in]
                      n751 = Concatenate Strings(w1378, "，" ("字符串"), w1381) -> (w1377:string)
                    }
                    n752 = local write "探头启用状态？"(w1372) -> ()
                    n753 = flat-sequence {
                      tunnel: w1368 -> [w1375]
                      frame #0 {
                        n754 = local write "限值"(w1375) -> ()
                      }
                      frame #1 {
                        w1376 = TRUE  # T
                        n755 = local write "限值变了？"(w1376) -> ()
                      }
                    }
                    n756 = call "状态栏-插入状态信息-35点监测专用.vi"("消息内容"=w1365, "状态类型"=enum16{"全部", "报警", "通信", "设置"}."设置") -> ()  [unwired: 10 in]
                  }
                  frame "启用" {
                    # "启用探头"
                    n757 = local read "探头启用状态？"() -> (w1394:bool[])
                    n758 = for {
                      tunnel: w1393 -> [w1400] mode=indexing
                      shift-right: [w1401] -> w1392
                      shift-left: w1394 -> [w1402]
                      shift-right: [w1398] -> w1389
                      shift-left: "启用探头" ("字符串") -> [w1399]
                      w1403 = TRUE  # T
                      n759 = Increment(x=w1400) -> (x+1=w1395:i32)
                      n760 = Replace Array Subset "更新 探头启用状态"(array=w1402, new element=w1403, index=w1400) -> (w1401:bool[])
                      n761 = Number To Decimal String(number=w1395) -> (decimal integer string=w1396:string)  [unwired: 1 in]
                      n762 = Concatenate Strings(w1399, "，" ("字符串"), w1396) -> (w1398:string)
                    }
                    n763 = local write "探头启用状态？"(w1392) -> ()
                    n764 = call "状态栏-插入状态信息-35点监测专用.vi"("消息内容"=w1389, "状态类型"=enum16{"全部", "报警", "通信", "设置"}."设置") -> ()  [unwired: 10 in]
                  }
                  frame "修改探头信息" {
                    # "只允许单项修改，探头名称不允许重复"
                    n765 = stacked-sequence {
                      tunnel: w1405 -> [_ w1414 _]
                      tunnel: w1404 -> [_ w1413 _]
                      frame #0 {
                        # "防止修改‘探头信息’‘累积剂量’造成读写冲突"
                        # "打开软键盘"
                        n766 = global read "全局变量-35点监测.vi" "屏幕键盘？"() -> (w1407:bool)
                        n767 = local write "暂停发送"(TRUE ("暂停发送")) -> ()
                        n768 = case shown="真" w1407 {
                          frame False {
                          }
                          frame True {
                            n769 = call "cmd启动屏幕键盘.vi"("软键盘开关"=enum16{"关闭", "打开"}."打开") -> ()  [unwired: 9 in, 2 out]
                          }
                        }
                      }
                      frame #1 {
                        # "弹窗修改"
                        n770 = local read "探头信息"() -> (w1409:string[])
                        n771 = for {
                          tunnel: w1414 -> [w1426]
                          tunnel: w1413 -> [w1424] mode=indexing
                          shift-right: [w1423] -> _
                          shift-left: w1409 -> [w1415]
                          shift-right: [w1421] -> w1411
                          shift-left: "修改探头信息：\n" -> [w1420]
                          # "依次修改探头信息"
                          n772 = Index Array(array=w1426, index=w1424) -> (element=w1425:i32)
                          n773 = Index Array(array=w1415, index=w1424) -> (element=w1416:string)
                          n774 = call "创建文本"("探头地址"=w1425) -> ("Result"=w1419:string)  [unwired: 13 in, 1 out]
                          n775 = call "修改探头名称.vi"("探头信息"=w1415, "原名称"=w1416, "输入信息"=w1419) -> ("确定修改？"=w1417:bool, "新名称 o"=w1418:string)  [unwired: 7 in]
                          n776 = case shown="真" w1417 {
                            tunnel: w1418 -> [_ w1432]
                            tunnel: w1415 -> [w1427 w1437]
                            tunnel: w1424 -> [_ w1435]
                            tunnel: [w1427 w1436] -> w1423
                            tunnel: w1416 -> [_ w1433]
                            tunnel: [_ w1429] -> w1422
                            frame False {
                              # "取消不修改"
                            }
                            frame True {
                              # "确定则修改"
                              n777 = Increment(x=w1435) -> (x+1=w1434:i32)
                              n778 = Replace Array Subset(array=w1437, new element=w1432, index=w1435) -> (w1436:string[])
                              n779 = call "创建文本2"("编号"=w1434, "原名称"=w1433, "新名称"=w1432) -> ("Result"=w1431:string)  [unwired: 11 in, 1 out]
                              n780 = local write "探头信息"(w1436) -> ()
                              n781 = Concatenate Strings("L-----------------------------------" ("字符串"), w1431, "\r") -> (w1429:string)
                            }
                          }
                          n782 = Concatenate Strings(w1420, w1422) -> (w1421:string)
                        }
                        n783 = call "状态栏-插入状态信息-35点监测专用.vi"("消息内容"=w1411, "状态类型"=enum16{"全部", "报警", "通信", "设置"}."设置") -> ()  [unwired: 10 in]
                      }
                      frame #2 {
                        # "关闭软键盘"
                        n784 = local write "暂停发送"(FALSE ("暂停发送")) -> ()
                        n785 = call "cmd启动屏幕键盘.vi"("软键盘开关"=enum16{"关闭", "打开"}."关闭") -> ()  [unwired: 9 in, 2 out]
                        n786 = property on="信号-保存配置" class="Bool (严格)"("Val(Sgnl)"=FALSE ("值(信号)")) -> ()  [unwired: 2 in, 2 out]
                      }
                    }
                  }
                  frame "交换探头地址" {
                    # "只可单项修改  与指定的探头 交换地址"
                    n787 = stacked-sequence {
                      tunnel: w1441 -> [_ w1447 _]
                      frame #0 {
                        # "暂停发送"
                        n788 = local write "暂停发送"(TRUE ("暂停发送")) -> ()
                      }
                      frame #1 {
                        # "修改"
                        n789 = control-ref of="实时数据列表"() -> (w1454:refnum<vi>)
                        n790 = control-ref of="报警状态"() -> (w1445:refnum<vi>)
                        n791 = control-ref of="缓存值"() -> (w1453:refnum<vi>)
                        n792 = control-ref of="发送次数"() -> (w1452:refnum<vi>)
                        n793 = control-ref of="限值"() -> (w1451:refnum<vi>)
                        n794 = control-ref of="异常保存记录？"() -> (w1450:refnum<vi>)
                        n795 = control-ref of="报警记录标志？"() -> (w1449:refnum<vi>)
                        n796 = control-ref of="探头信息"() -> (w1446:refnum<vi>)
                        n797 = control-ref of="探头启用状态？"() -> (w1448:refnum<vi>)
                        n798 = Bundle By Name(cluster=T19 {"实时数据列表"=refnum, "缓存值"=refnum, "发送次数"=refnum, "限值"=refnum, "异常保存记录？"=refnum, "报警记录标志？"=refnum, "探头启用状态？"=refnum, "探头信息"=refnum, "报警状态"=refnum} ("引用输入"), "实时数据列表"=w1454, "缓存值"=w1453, "发送次数"=w1452, "限值"=w1451, "异常保存记录？"=w1450, "报警状态"=w1445, "报警记录标志？"=w1449, "探头启用状态？"=w1448, "探头信息"=w1446) -> (w1443:T19)
                        n799 = call "交换探头地址.vi"("引用输入"=w1443, "点到行列-实时列表"=w1447) -> ()  [unwired: 8 in, 2 out]
                      }
                      frame #2 {
                        # "恢复发送"
                        n800 = local write "暂停发送"(FALSE ("暂停发送")) -> ()
                      }
                    }
                  }
                  frame "微调测量值" {
                    # "单项可调"
                    n801 = disable-structure shown="启用" {
                      disable-tunnel: w1457 -> [w1461 _]
                      disable-tunnel: w1456 -> [w1460 _]
                      frame Disabled {
                        n802 = Index Array(array=w1460) -> (element=w1459:i32)  [unwired: 1 in]
                        n803 = Index Array(array=w1461, index=w1459) -> (element=w1458:i32)
                        n804 = control-ref of="本VI"() -> (w1462:refnum<vi>)
                        n805 = global read "全局变量-35点监测.vi" "COM口"() -> (w1463:refnum<visa-resource-name>)
                        n806 = call "修改-微调探头测量值-30.vi"("VI引用句柄"=w1462, "探头地址"=w1458, "VISA资源名称"=w1463) -> ()  [unwired: 8 in, 1 out]
                      }
                      frame Enabled {
                      }
                    }
                  }
                  frame "探头排序", Default {
                    # "进入可拖拽模式"
                  }
                  frame "备注信息" {
                    # "批量编辑 备注信息，进入可编辑模式（一些版本中禁用了此功能）"
                    n807 = stacked-sequence {
                      frame #0 {
                        w1465 = TRUE  # F
                        w1466 = TRUE  # T
                        # "暂停发送"
                        n808 = local write "T:G,F:B"(w1465) -> ()
                        n809 = local write "暂停发送"(w1466) -> ()
                        n810 = Wait (ms)(milliseconds to wait=u32 3000 ("等待时间（毫秒）")) -> ()  [unwired: 1 out]
                      }
                      frame #1 {
                        w1468 = TRUE  # T
                        w1471 = TRUE  # T
                        # "进入编辑模式"
                        n811 = property on="实时数据列表" class="MCListbox (严格)"("Allow Editing Cells"=w1471) -> ("ItemNames"=→"编辑前项名":string[][])  [unwired: 2 in, 2 out]
                        n812 = property on="状态与编辑" class="Bool (严格)"("Value"=w1468, "DisabledEnum"=T8."Enabled" ("禁用"), "BoolText.Text"="点此完成编辑" ("布尔文本.文本")) -> ()  [unwired: 2 in, 2 out]
                      }
                      frame #2 {
                        # "状态栏提示"
                        n813 = call "状态栏-插入状态信息-35点监测专用.vi"("消息内容"="现在进入可编辑模式，点击“探头信息列”单元格进行编辑，按菜单左上按钮完成编辑。", "状态类型"=enum16{"全部", "报警", "通信", "设置"}."设置") -> ()  [unwired: 10 in]
                      }
                    }
                  }
                  frame "修改报警限值" {
                    # "允许批量修改"
                    n814 = stacked-sequence {
                      tunnel: w1475 -> [_ _ _]
                      tunnel: w1474 -> [_ w1483 _]
                      frame #0 {
                        # "暂停读数据"
                        n815 = local write "暂停发送"(TRUE ("暂停发送")) -> ()
                      }
                      frame #1 {
                        w1478 = enum16{"全部限值", "一级限值", "二级限值"}."全部限值"  # 全部
                        n816 = global read "全局变量-35点监测.vi" "COM口"() -> (w1481:refnum<visa-resource-name>)
                        n817 = control-ref of="实时数据列表"() -> (w1477:refnum<vi>)
                        n818 = control-ref of="本VI"() -> (w1482:refnum<vi>)
                        n819 = local read "限值"() -> (w1480:T4)
                        n820 = call "修改-探头报警值-30.vi"("VI引用句柄"=w1482, "修改模式"=w1478, "VISA资源名称"=w1481, "限值 i"=w1480, "探头地址"=w1483, "实时数据列表"=w1477) -> ("限值 o"=w1479:T4)  [unwired: 5 in]
                        n821 = local write "限值"(w1479) -> ()
                      }
                      frame #2 {
                        w1486 = TRUE  # T
                        # "使改变生效，恢复数据读取"
                        n822 = property on="信号-保存配置" class="Bool (严格)"("Val(Sgnl)"=FALSE ("值(信号)")) -> ()  [unwired: 2 in, 2 out]
                        n823 = local write "限值变了？"(w1486) -> ()
                        n824 = local write "暂停发送"(FALSE ("暂停发送")) -> ()
                      }
                    }
                  }
                  frame "累积清零" {
                    n825 = stacked-sequence {
                      seq-local: [w1491 _ _ _] -> [_ w1506 w1524 _]
                      seq-local: [w1490 _ _ _] -> [_ w1505 w1523 _]
                      tunnel: w1489 -> [w1496 _ _ _]
                      tunnel: w1488 -> [w1495 _ _ _]
                      tunnel: w1487 -> [w1493 _ _ _]
                      frame #0 {
                        # "弹窗提示"
                        n826 = for {
                          tunnel: w1496 -> [w1502] mode=indexing
                          tunnel: w1495 -> [w1503]
                          shift-right: [w1498] -> w1492
                          shift-left: "确认清零以下设备？\n" -> [w1500]
                          tunnel: w1493 -> [w1504]
                          tunnel: [w1497] -> w1490 mode=indexing
                          # "创建提示语"
                          n827 = Index Array(array=w1503, index=w1502) -> (element=w1501:i32)
                          n828 = Index Array(array=w1504, index=w1502) -> (element=w1497:string)
                          n829 = call "创建文本4"("地址"=w1501, "名称"=w1497) -> ("Result"=w1499:string)  [unwired: 12 in, 1 out]
                          n830 = Concatenate Strings(w1500, w1499) -> (w1498:string)
                        }
                        n831 = call "显示对话框信息2"("Message"=w1492) -> ("确定"=w1491:bool)  [unwired: 9 in, 1 out]
                      }
                      frame #1 {
                        # "执行设置"
                        n832 = case shown="真" w1506 {
                          tunnel: w1505 -> [_ w1510]
                          frame False {
                            # "取消清零"
                          }
                          frame True {
                            # "执行清零"
                            n833 = local read "累积剂量"() -> (w1511:T2)
                            n834 = for {
                              tunnel: w1511 -> [w1514] mode=indexing
                              tunnel: w1510 -> [w1517]
                              tunnel: [w1512] -> w1507 mode=indexing
                              n835 = Unbundle By Name(w1514) -> ("设备名称"=w1516:string)
                              n836 = Search 1D Array(1D array=w1517, element=w1516) -> (index of element=w1515:i32)  [unwired: 1 in]
                              n837 = Greater Or Equal To 0?(x=w1515) -> (x >= 0?=w1513:bool)
                              n838 = case shown="真" w1513 {
                                tunnel: w1514 -> [w1518 w1522]
                                tunnel: [w1518 w1519] -> w1512
                                frame False {
                                # "未匹配，不清零"
                                }
                                frame True {
                                # "匹配到，清零"
                                n839 = Get Date/Time In Seconds() -> (seconds since 1Jan1904=w1521:timestamp)
                                n840 = Bundle By Name(cluster=w1522, "起始时间"=w1521, "累积剂量"=0.0) -> (w1519:T20)
                                }
                              }
                            }
                            n841 = call "路径查找创建-报警记录清单.vi"() -> ("累积剂量配置文件"=w1509:path)  [unwired: 8 in, 11 out]
                            n842 = local write "累积剂量"(w1507) -> ()
                            n843 = Flatten To XML(anything=w1507) -> (xml string=w1508:string)
                            n844 = call-poly <vilib>:"Write to XML File.vi"("XML Input"=w1508, "XML File Path"=w1509) -> ()  [unwired: 7 in, 3 out]
                          }
                        }
                      }
                      frame #2 {
                        # "状态提醒"
                        n845 = case shown="真" w1524 {
                          tunnel: w1523 -> [_ w1527]
                          frame False {
                          }
                          frame True {
                            # "更新状态"
                            n846 = for {
                              tunnel: w1527 -> [w1530] mode=indexing
                              shift-right: [w1531] -> w1525
                              shift-left: "累计剂量已清零：" -> [w1532]
                              # "构建文本"
                              n847 = Concatenate Strings(w1532, w1530, "，" ("字符串")) -> (w1531:string)
                            }
                            n848 = call "状态栏-插入状态信息-35点监测专用.vi"("消息内容"=w1525, "状态类型"=enum16{"全部", "报警", "通信", "设置"}."设置") -> ()  [unwired: 10 in]
                          }
                        }
                      }
                      frame #3 {
                        # "保存累积剂量"
                      }
                    }
                  }
                  frame "累积报警阈值" {
                    n849 = for {
                      tunnel: w1539 -> [w1541] mode=indexing
                      tunnel: w1538 -> [w1542]
                      tunnel: [w1540] -> w1536 mode=indexing
                      # "待修改探头列表"
                      n850 = Index Array(array=w1542, index=w1541) -> (element=w1540:string)
                    }
                    n851 = local read "累积剂量"() -> (w1537:T2)
                    n852 = call "修改累积剂量报警阈值.vi"("待修改探头"=w1536, "累积剂量 i"=w1537) -> ("累积剂量 o"=w1533:T2)  [unwired: 9 in]
                    n853 = local write "累积剂量"(w1533) -> ()
                    n854 = call "路径查找创建-报警记录清单.vi"() -> ("累积剂量配置文件"=w1535:path)  [unwired: 8 in, 11 out]
                    n855 = Flatten To XML(anything=w1533) -> (xml string=w1534:string)
                    n856 = call-poly <vilib>:"Write to XML File.vi"("XML Input"=w1534, "XML File Path"=w1535) -> ()  [unwired: 7 in, 3 out]
                  }
                  frame "启用累积" {
                    # "可批量启用累积剂量记录"
                    n857 = local read "累积剂量"() -> (w1549:T2)
                    n858 = for {
                      tunnel: w1551 -> [_]
                      tunnel: w1550 -> [w1561]
                      tunnel: w1549 -> [w1559] mode=indexing
                      tunnel: [w1558] -> w1543 mode=indexing
                      shift-right: [w1552] -> w1546
                      shift-left: "启用累积剂量：" -> [w1555]
                      # "替换一遍"
                      n859 = Unbundle By Name(w1559) -> ("设备名称"=w1556:string)
                      n860 = Search 1D Array(1D array=w1561, element=w1556) -> (index of element=w1560:i32)  [unwired: 1 in]
                      n861 = Greater Or Equal To 0? "匹配到？"(x=w1560) -> (x >= 0?=w1557:bool)
                      n862 = case shown="真" w1557 {
                        tunnel: w1559 -> [w1562 w1568]
                        tunnel: [w1562 w1570] -> w1558
                        tunnel: w1556 -> [_ w1569]
                        tunnel: [_ w1569] -> w1554
                        frame False {
                          # "无匹配"
                        }
                        frame True {
                          w1571 = TRUE  # T
                          # "匹配到"
                          n863 = Unbundle By Name(w1568) -> ("起始时间"=w1564:timestamp)
                          n864 = Get Date/Time In Seconds() -> (seconds since 1Jan1904=w1565:timestamp)
                          n865 = Equal? "空？"(x=w1564, y=timestamp(0 s since 1904-01-01)) -> (x = y?=w1566:bool)
                          n866 = Select(t=w1565, s=w1566, f=w1564) -> (s? t:f=w1563:timestamp)
                          n867 = Bundle By Name(cluster=w1568, "启用累积？"=w1571, "起始时间"=w1563) -> (w1570:T20)
                        }
                      }
                      n868 = Concatenate Strings(w1555, w1554, "，" ("字符串")) -> (w1552:string)
                    }
                    n869 = call "路径查找创建-报警记录清单.vi"() -> ("累积剂量配置文件"=w1545:path)  [unwired: 8 in, 11 out]
                    n870 = local write "累积剂量"(w1543) -> ()
                    n871 = call "状态栏-插入状态信息-35点监测专用.vi"("消息内容"=w1546, "状态类型"=enum16{"全部", "报警", "通信", "设置"}."设置") -> ()  [unwired: 10 in]
                    n872 = Flatten To XML(anything=w1543) -> (xml string=w1544:string)
                    n873 = call-poly <vilib>:"Write to XML File.vi"("XML Input"=w1544, "XML File Path"=w1545) -> ()  [unwired: 7 in, 3 out]
                  }
                  frame "禁用累积" {
                    n874 = local read "累积剂量"() -> (w1579:T2)
                    n875 = for {
                      tunnel: w1578 -> [w1589]
                      tunnel: w1579 -> [w1587] mode=indexing
                      tunnel: [w1586] -> w1572 mode=indexing
                      shift-right: [w1580] -> w1575
                      shift-left: "禁用累积剂量：" -> [w1583]
                      # "替换一遍"
                      n876 = Unbundle By Name(w1587) -> ("设备名称"=w1584:string)
                      n877 = Search 1D Array(1D array=w1589, element=w1584) -> (index of element=w1588:i32)  [unwired: 1 in]
                      n878 = Greater Or Equal To 0? "匹配到？"(x=w1588) -> (x >= 0?=w1585:bool)
                      n879 = case shown="真" w1585 {
                        tunnel: w1587 -> [w1590 w1594]
                        tunnel: [w1590 w1592] -> w1586
                        tunnel: w1584 -> [_ w1591]
                        tunnel: [_ w1591] -> w1582
                        frame False {
                          # "无匹配"
                        }
                        frame True {
                          w1593 = FALSE  # F
                          # "匹配到"
                          n880 = Bundle By Name(cluster=w1594, "启用累积？"=w1593) -> (w1592:T20)
                        }
                      }
                      n881 = Concatenate Strings(w1583, w1582, "，" ("字符串")) -> (w1580:string)
                    }
                    n882 = local write "累积剂量"(w1572) -> ()
                    n883 = call "路径查找创建-报警记录清单.vi"() -> ("累积剂量配置文件"=w1574:path)  [unwired: 8 in, 11 out]
                    n884 = call "状态栏-插入状态信息-35点监测专用.vi"("消息内容"=w1575, "状态类型"=enum16{"全部", "报警", "通信", "设置"}."设置") -> ()  [unwired: 10 in]
                    n885 = Flatten To XML(anything=w1572) -> (xml string=w1573:string)
                    n886 = call-poly <vilib>:"Write to XML File.vi"("XML Input"=w1573, "XML File Path"=w1574) -> ()  [unwired: 7 in, 3 out]
                  }
                  frame "探头报警方式" {
                    # "允许批量设置，‘常报警’‘自动静音’‘手动静音’"
                    n887 = call "弹窗-设置探头报警方式.vi"() -> ("探头报警方式 o"=w1596:enum16{"常报警", "自动静音", "手动静音"}, "确定？"=w1597:bool)  [unwired: 10 in]
                    n888 = case shown="真" w1597 {
                      tunnel: w1596 -> [_ w1607]
                      tunnel: w1595 -> [_ w1606]
                      frame False {
                        # "取消修改"
                      }
                      frame True {
                        # "确认修改"
                        n889 = local read "报警方式"() -> (w1605:T1)
                        n890 = for {
                          shift-right: [w1620] -> w1598
                          shift-left: w1605 -> [w1621]
                          tunnel: w1607 -> [w1619]
                          tunnel: w1606 -> [w1618] mode=indexing
                          shift-right: [w1614] -> w1601
                          shift-left: "" -> [w1613]
                          # "批量修改报警方式"
                          n891 = in-place {
                            in-place-border: w1619 -> [w1623]
                            n892 = in-place-array #7(w1621, w1618) -> (w1624:T27)
                            n893 = in-place {
                              in-place-border: w1623 -> [w1626]
                              n894 = in-place-cluster #8(w1624) -> ()  [unwired: 2 out]
                              n895 = in-place-cluster #8("报警方式"=w1626, "延迟计时"=u16 0) -> (w1622:T27)
                            }
                            n896 = in-place-array #7(w1622) -> (w1620:T1)  [unwired: 1 out]
                          }
                          n897 = Increment(x=w1618) -> (x+1=w1617:i32)
                          n898 = Number To Decimal String(number=w1617) -> (decimal integer string=w1616:string)  [unwired: 1 in]
                          n899 = Concatenate Strings(w1613, w1616, ", ") -> (w1614:string)
                        }
                        n900 = case shown="\"手动静音\"" w1607 {
                          tunnel: ["常报警" "自动静音" "手动静音"] -> w1600
                          frame "常报警", Default {
                          }
                          frame "自动静音" {
                          }
                          frame "手动静音" {
                          }
                        }
                        n901 = local write "报警方式"(w1598) -> ()
                        n902 = flat-sequence {
                          tunnel: w1598 -> [_]
                          frame #0 {
                            w1608 = TRUE  # T
                            n903 = local write "报警方式变了？"(w1608) -> ()
                            n904 = property on="信号-保存配置" class="Bool (严格)"("Val(Sgnl)"=FALSE ("值(信号)")) -> ()  [unwired: 2 in, 2 out]
                          }
                        }
                        n905 = Concatenate Strings(w1601, " 号探头 探头报警方式设为 ", w1600) -> (w1599:string)
                        n906 = call "状态栏-插入状态信息-35点监测专用.vi"("消息内容"=w1599, "状态类型"=enum16{"全部", "报警", "通信", "设置"}."设置") -> ()  [unwired: 10 in]
                      }
                    }
                  }
                }
              }
              frame True {
                # "暂停发送状态下，不允许产生菜单事件"
              }
            }
          }
          event "菜单项-报警列表": Value Change {
            # "报警列表，菜单事件处理"
            n907 = event-data() -> ("CtlRef"=w1628:refnum<vi>)  [unwired: 1 in, 5 out]
            n908 = local read "点到行列-报警记录"() -> (w1627:T5)
            n909 = local read "暂停发送"() -> (w1629:bool)
            n910 = case shown="假" w1629 {
              tunnel: w1628 -> [w1635 _]
              tunnel: w1627 -> [w1633 _]
              frame False {
                # "非暂停，可执行"
                n911 = local read "报警记录缓存数据文件"() -> (w1632:string[])
                n912 = local read "报警记录列表"() -> (w1630:i32[])
                n913 = property class="Enum (严格)"(reference=w1635) -> ("RingText.Text"=w1634:string)  [unwired: 1 in, 2 out]
                n914 = Unbundle By Name(w1633) -> ()  [unwired: 1 out]
                n915 = for {
                  tunnel: w1632 -> [w1638]
                  tunnel: [w1637] -> w1631 mode=indexing
                  tunnel: w1630 -> [w1636] mode=indexing
                  n916 = Index Array(array=w1638, index=w1636) -> (element=w1637:string)
                }
                n917 = case shown="\"预览并生成报表\"" w1634 {
                  tunnel: w1631 -> [_ _ w1657 w1693 _]
                  tunnel: w1630 -> [_ _ w1651 _ w1720]
                  frame "假", Default {
                  }
                  frame "刷新" {
                    # "刷新报警记录清单"
                    n918 = call "读取-缓存数据文件夹至报警记录列表.vi"() -> ("文件名"=w1640:string[], "新记录文件名"=w1642:string[], "新记录列表"=w1643:string[][], "报警记录列表"=w1646:string[][])  [unwired: 8 in]
                    "报警记录缓存数据文件" <- w1640
                    n919 = Array Size(array=w1640) -> (size(s)=w1639:i32)
                    n920 = for {
                      workers-P: _ -> [_]
                      tunnel: w1643 -> [w1649] mode=indexing
                      tunnel: w1642 -> [w1648] mode=indexing
                      tunnel: [w1647] -> w1641 mode=indexing
                      # "数组到簇绑定"
                      n921 = Bundle("新记录列表"=w1649, "字符串"=w1648) -> (w1647:cluster{"新记录列表":string[], "字符串":string})  [unwired: 1 in]
                    }
                    n922 = local write "报警记录数"(w1639) -> ()
                    n923 = property on="报警记录列表" class="MCListbox (严格)"("ItemNames"=w1646, "Value"=i32[] [] ("报警记录列表"), "TopLeft"=T6 {"Row"=0, "Column"=0} ("左上可见单元格")) -> ()  [unwired: 2 in, 2 out]
                    n924 = property on="新记录簇" class="Arr (严格)"("Val(Sgnl)"=w1641) -> ()  [unwired: 2 in, 2 out]
                  }
                  frame "预览并生成报表" {
                    # "获得文件路径，预览并生成报表"
                    n925 = property on="报警记录列表" class="MCListbox (严格)"() -> ("ItemNames"=w1652:string[][])  [unwired: 2 in, 2 out]
                    n926 = Array Size(array=w1652) -> (size(s)=w1653:i32[])
                    n927 = Index Array(array=w1651) -> (element=w1654:i32)  [unwired: 1 in]
                    n928 = Index Array(array=w1653) -> (element=w1655:i32)  [unwired: 1 in]
                    n929 = Increment(x=w1654) -> (x+1=w1656:i32)
                    n930 = Greater Or Equal? "有效行？"(x=w1655, y=w1656) -> (x >= y?=w1650:bool)
                    n931 = case shown="真" w1650 {
                      tunnel: w1657 -> [_ w1658]
                      frame False {
                      }
                      frame True {
                        n932 = call "路径查找创建-报警记录清单.vi"() -> ("缓存数据文件夹"=w1659:path)  [unwired: 8 in, 11 out]
                        n933 = vi-ref "生成报表.vi"() -> (w1660:refnum<vi>)
                        n934 = disable-structure shown="启用" {
                          disable-tunnel: w1660 -> [w1663 w1674]
                          disable-tunnel: w1659 -> [w1662 w1673]
                          disable-tunnel: w1658 -> [w1661 w1672]
                          frame Disabled {
                            n935 = for {
                              tunnel: w1663 -> [w1670]
                              tunnel: w1662 -> [w1666]
                              tunnel: w1661 -> [w1664] mode=indexing
                              # "打开多个窗口？"
                              n936 = property class="VI"(reference=w1670) -> ("Name"=w1669:string)  [unwired: 1 in, 2 out]
                              n937 = Build Path(base path=w1666, name or relative path=w1664) -> (appended path=w1665:path)
                              n938 = Open VI Reference(type specifier VI Refnum (for type only)=refnum<vi> refnum ("类型说明符VI引用句柄（仅用于类型）"), vi path=w1669, options=128 ("选项")) -> (vi reference=w1667:refnum<vi>)  [unwired: 3 in, 1 out]
                              n939 = call-by-ref "开始异步调用"(reference=w1667, "缓存数据路径"=w1665) -> ()  [unwired: 12 in, 2 out]
                            }
                          }
                          frame Enabled {
                            n940 = Index Array(array=w1672) -> (element=w1675:string)  [unwired: 1 in]
                            n941 = Build Path(base path=w1673, name or relative path=w1675) -> (appended path=w1682:path)
                            n942 = invoke class="VI" method="FP.Open"(reference=w1674, "Activate"=TRUE ("激活？"), "State"=T7."Hidden" ("状态")) -> (reference out=w1678:refnum<vi>, error out=w1691:errorcluster)  [unwired: 2 in, 3 out]
                            n943 = call "通过控件名获取控件引用.vi"("控件名数组"=string[] ["缓存数据路径"], "VI引用"=w1678) -> ("控件引用输出"=w1680:refnum<vi>[], "VI引用o"=w1683:refnum<vi>)  [unwired: 7 in, 1 out]
                            n944 = Index Array(array=w1680) -> (element=w1681:refnum<vi>)  [unwired: 1 in]
                            n945 = property class="Ctl"(reference=w1681, error in=w1691, "Val(Sgnl)"=w1682) -> (error out=w1692:errorcluster)  [unwired: 1 out]
                            n946 = invoke class="VI" method="Run VI"(reference=w1683, error in=w1692, "Wait until done"=FALSE ("结束前等待"), "Auto Dispose Ref"=TRUE ("自动销毁引用")) -> (reference out=w1686:refnum<vi>, error out=w1687:errorcluster)  [unwired: 1 in, 3 out]
                            n947 = invoke class="VI" method="FP.Open"(reference=w1686, error in=w1687, "Activate"=TRUE ("激活？"), "State"=T7."Standard" ("状态")) -> (error out=w1690:errorcluster)  [unwired: 1 in, 4 out]
                            n948 = call <vilib>:"Clear Errors.vi"("error in (no error)"=w1690) -> ()  [unwired: 5 in, 2 out]
                          }
                        }
                      }
                    }
                  }
                  frame "删除记录" {
                    # "删除缓存的xml文件，然后刷新"
                    n949 = stacked-sequence {
                      seq-local: [w1694 _ _ _] -> [_ _ w1701 _]
                      seq-local: [_ w1700 _ _] -> [_ _ w1702 _]
                      tunnel: w1693 -> [w1695 _ _ _]
                      frame #0 {
                        # "删除缓存数据xml文件"
                        n950 = call "路径查找创建-报警记录清单.vi"() -> ("缓存数据文件夹"=w1696:path)  [unwired: 8 in, 11 out]
                        n951 = for {
                          tunnel: w1696 -> [w1699]
                          tunnel: w1695 -> [w1698] mode=indexing
                          tunnel: [w1697] -> w1694 mode=indexing
                          n952 = Build Path(base path=w1699, name or relative path=w1698) -> (appended path=w1697:path)
                        }
                      }
                      frame #1 {
                        # "弹窗确认"
                        n953 = call "显示对话框信息"() -> ("确定"=w1700:bool)  [unwired: 10 in, 1 out]
                      }
                      frame #2 {
                        # "删除操作"
                        n954 = case shown="真" w1702 {
                          tunnel: w1701 -> [_ w1703]
                          frame False {
                          }
                          frame True {
                            n955 = for {
                              workers-P: _ -> [_]
                              tunnel: w1703 -> [w1705] mode=indexing
                              n956 = Delete(path (use dialog)=w1705) -> (error out=w1704:errorcluster)  [unwired: 4 in, 2 out]
                              n957 = call <vilib>:"Clear Errors.vi"("error in (no error)"=w1704) -> ()  [unwired: 5 in, 2 out]
                            }
                          }
                        }
                      }
                      frame #3 {
                        # "刷新列表"
                        n958 = call "读取-缓存数据文件夹至报警记录列表.vi"() -> ("文件名"=w1707:string[], "报警记录列表"=w1708:string[][])  [unwired: 8 in, 2 out]
                        n959 = local write "报警记录缓存数据文件"(w1707) -> ()
                        n960 = property on="报警记录列表" class="MCListbox (严格)"("ItemNames"=w1708, "Value"=i32[] [] ("报警记录列表")) -> ()  [unwired: 2 in, 2 out]
                      }
                    }
                  }
                  frame "复制选中项至剪贴板" {
                    # "复制列表数据到剪贴板"
                    n961 = property on="报警记录列表" class="MCListbox (严格)"() -> ("ItemNames"=w1723:string[][])  [unwired: 2 in, 2 out]
                    n962 = for {
                      tunnel: w1723 -> [w1727] mode=indexing
                      tunnel: [w1728] -> w1722 mode=indexing
                      tunnel: [w1727] -> w1719
                      n963 = To Variant(anything=w1727) -> (Variant=w1728:variant)
                    }
                    n964 = call "重排数组.vi"("新索引顺序"=w1720, "原数组"=w1722) -> ("排序后数组"=w1721:variant[])  [unwired: 9 in]
                    n965 = call "状态栏-插入状态信息-35点监测专用.vi"("消息内容"="已复制 报警记录列表选中项 至剪贴板", "状态类型"=enum16{"全部", "报警", "通信", "设置"}."设置") -> ()  [unwired: 10 in]
                    n966 = for {
                      tunnel: w1721 -> [w1726] mode=indexing
                      tunnel: w1719 -> [w1725]
                      tunnel: [w1724] -> w1718 mode=indexing
                      n967 = Variant To Data(type=w1725, Variant=w1726) -> (data=w1724:string[])  [unwired: 1 in, 1 out]
                    }
                    n968 = Array To Spreadsheet String(array=w1718, 3:"%s" ("格式字符串")) -> (spreadsheet string=w1711:string)  [unwired: 1 in]
                    n969 = Array To Spreadsheet String(array=string[] ["报警时间", "探头编号", "探头信息", "最大值（μSv/h）", "报警等级"] ("ItemNames"), 3:"%s" ("格式字符串")) -> (spreadsheet string=w1709:string)  [unwired: 1 in]
                    n970 = control-ref of="本应用程序"() -> (w1716:refnum<vi>)
                    n971 = Concatenate Strings(w1709, w1711) -> (w1710:string)
                    n972 = invoke class="App" method="Clipboard.Write"(reference=w1716, "Param 0"=w1710) -> ()  [unwired: 2 in, 4 out]
                  }
                }
              }
              frame True {
                # "暂停发送，不执行"
              }
            }
          }
          event "报警记录列表": Key Down {
            (unwired) eventvkey."ASCII" ("V键")
            # "用于删除（delete）或打开（enter）报警记录的 键盘快捷键"
            n973 = event-data() -> ("CtlRef"=w1735:refnum<vi>, "VKey"=w1741:T34)  [unwired: 1 in, 8 out]
            n974 = property class="MCListbox (严格)"(reference=w1735) -> ("Value"=w1732:i32[])  [unwired: 1 in, 2 out]
            n975 = property class="MCListbox (严格)"(reference=w1735) -> ("ItemNames"=w1738:string[][])  [unwired: 1 in, 2 out]
            n976 = Array Size(array=w1738) -> (size(s)=w1737:i32[])
            n977 = Array Size(array=w1732) -> (size(s)=w1739:i32)
            n978 = Index Array(array=w1732) -> (element=w1731:i32)  [unwired: 1 in]
            n979 = Index Array(array=w1737) -> (element=w1736:i32)  [unwired: 1 in]
            n980 = Greater Than 0?(x=w1739) -> (x > 0?=w1740:bool)
            n981 = Decrement(x=w1736) -> (x-1=w1733:i32)
            n982 = In Range and Coerce(upper limit=w1733, x=w1731, lower limit=0 ("下限")) -> (In Range?=w1729:bool)  [unwired: 1 out]
            n983 = And(x=w1729, y=w1740) -> (x .and. y?=w1730:bool)
            n984 = case shown="真" w1730 {
              tunnel: w1741 -> [_ w1743]
              tunnel: w1739 -> [_ w1742]
              frame False {
                # "空数组，不执行"
              }
              frame True {
                # "范围内，数组非空，执行"
                n985 = case shown="\"Delete\"" w1743 {
                  tunnel: w1742 -> [_ w1745 _]
                  frame "ASCII", Default {
                    # "无操作"
                  }
                  frame "Enter", "Return" {
                    # "打开记录，仅单选时"
                    n986 = Equal?(x=w1745, y=1) -> (x = y?=w1746:bool)
                    n987 = case shown="真" w1746 {
                      frame False {
                      }
                      frame True {
                        # "单选"
                        n988 = property on="菜单项-报警列表" class="Enum (严格)"("Val(Sgnl)"=enum16{"刷新", "预览并生成报表", "删除记录", "复制选中项至剪贴板"}."预览并生成报表" ("值(信号)")) -> ()  [unwired: 2 in, 2 out]
                      }
                    }
                  }
                  frame "Delete" {
                    # "删除记录"
                    n989 = property on="菜单项-报警列表" class="Enum (严格)"("Val(Sgnl)"=enum16{"刷新", "预览并生成报表", "删除记录", "复制选中项至剪贴板"}."删除记录" ("值(信号)")) -> ()  [unwired: 2 in, 2 out]
                  }
                }
              }
            }
          }
          event "状态与编辑": Value Change {
            n990 = event-data() -> ("OldVal"=w1751:bool, "NewVal"=w1750:bool)  [unwired: 1 in, 4 out]
            n991 = Not Equal?(x=w1751, y=w1750) -> (x != y?=w1749:bool)
            n992 = case "条件结构" shown="真" w1749 {
              tunnel: w1750 -> [_ w1752]
              frame False {
                # "值未改变"
              }
              frame True {
                # "值有变化"
                n993 = case shown="假" w1752 {
                  frame False {
                    # "点击  结束修改"
                    n994 = stacked-sequence {
                      frame #0 {
                        w1756 = 2 ("禁用的索引 (列)")
                        # "更改受影响的项"
                        n995 = local read "编辑前项名"() -> (w1757:string[][])
                        n996 = property on="实时数据列表" class="MCListbox (严格)"() -> (error out=w1754:errorcluster, "ItemNames"=w1758:string[][])  [unwired: 2 in, 1 out]
                        n997 = Index Array "探头信息列"(array=w1758, index (col)=w1756) -> (element=w1753:string[])  [unwired: 1 in]
                        n998 = local write "探头信息"(w1753) -> ()
                        n999 = Replace Array Subset(array=w1757, new element=w1753, index (col)=w1756) -> (w1755:string[][])  [unwired: 1 in]
                        n1000 = property on="实时数据列表" class="MCListbox (严格)"(error in=w1754, "Allow Editing Cells"=FALSE ("允许编辑单元格"), "ItemNames"=w1755) -> ()  [unwired: 1 in, 2 out]
                      }
                      frame #1 {
                        # "更改标志，使在状态机中检测到更改"
                        n1001 = flat-sequence {
                          frame #0 {
                            w1760 = TRUE  # T
                            n1002 = local write "变了？"(w1760) -> ()
                          }
                          frame #1 {
                            w1762 = FALSE  # F
                            n1003 = local write "暂停发送"(w1762) -> ()
                            n1004 = property on="状态与编辑" class="Bool (严格)"("DisabledEnum"=T8."Disabled" ("禁用")) -> ()  [unwired: 2 in, 2 out]
                          }
                        }
                      }
                      frame #2 {
                        # "状态栏提示"
                        n1005 = call "状态栏-插入状态信息-35点监测专用.vi"("消息内容"="修改探头信息成功", "状态类型"=enum16{"全部", "报警", "通信", "设置"}."设置") -> ()  [unwired: 10 in]
                      }
                    }
                  }
                  frame True {
                    # "不执行"
                  }
                }
              }
            }
          }
          event "设置": Value Change {
            # "设置"
            n1006 = event-data() -> ()  [unwired: 1 in, 6 out]
            n1007 = property on="信号-设置" class="Bool (严格)"("Val(Sgnl)"=FALSE ("值(信号)")) -> ()  [unwired: 2 in, 2 out]
          }
          event "信号-保存配置": Value Change {
            w1766 = T25 {"COM"="", "探头地址"=[], "探头启用状态？"=[], "开机启动？"=FALSE, "探头信息"=[], "限值"=[], "最大探头数"=0, "波特率"=enum."19200", "周期"=0, "报警方式"=[], "静音延迟"=0}  # 配置内容
            w1769 = FALSE  # F
            # "设置之后，保存配置"
            n1008 = event-data() -> ()  [unwired: 1 in, 6 out]
            n1009 = local read "探头启用状态？"() -> (w1780:bool[])
            n1010 = global read "全局变量-35点监测.vi" "最大探头数"() -> (w1782:i32)
            n1011 = local read "探头地址"() -> (w1775:i32[])
            n1012 = global read "全局变量-35点监测.vi" "COM口"() -> (w1776:refnum<visa-resource-name>)
            n1013 = global read "全局变量-35点监测.vi" "静音延迟 s"() -> (w1767:u16)
            n1014 = local read "探头信息"() -> (w1781:string[])
            n1015 = local read "报警方式"() -> (w1768:T1)
            n1016 = local read "周期"() -> (w1770:i64)
            n1017 = global read "全局变量-35点监测.vi" "波特率"() -> (w1774:enum16{"9600", "19200"})
            n1018 = local read "限值"() -> (w1779:T4)
            n1019 = Bundle By Name(cluster=w1766, "限值"=w1779, "COM"=w1776, "探头地址"=w1775, "探头启用状态？"=w1780, "最大探头数"=w1782, "开机启动？"=w1769, "探头信息"=w1781, "波特率"=w1774, "周期"=w1770, "报警方式"=w1768, "静音延迟"=w1767) -> (w1777:T25)
            n1020 = local read "累积剂量"() -> (w1773:T2)
            n1021 = Flatten To XML(anything=w1777) -> (xml string=w1778:string)
            n1022 = call "路径查找创建-报警记录清单.vi"() -> ("配置文件"=w1783:path, "累积剂量配置文件"=w1771:path)  [unwired: 8 in, 10 out]
            n1023 = Flatten To XML(anything=w1773) -> (xml string=w1772:string)
            n1024 = call-poly <vilib>:"Write to XML File.vi"("XML Input"=w1772, "XML File Path"=w1771) -> ()  [unwired: 7 in, 3 out]
            n1025 = call-poly <vilib>:"Write to XML File.vi"("XML Input"=w1778, "XML File Path"=w1783) -> ()  [unwired: 7 in, 3 out]
          }
          event Panel Resize {
            # "允许纵向调整大小"
            n1026 = event-data() -> ("VIRef"=w1785:refnum<vi>, "NewBnds"=w1784:T23)  [unwired: 1 in, 6 out]
            n1027 = disable-structure shown="禁用" {
              disable-tunnel: w1785 -> [w1789 _]
              disable-tunnel: w1784 -> [w1788 _]
              frame Disabled {
                n1028 = Bundle By Name(cluster=w1788, "Left"="Left", "Right"="Right") -> (w1790:T23)
                n1029 = property class="VI"(reference=w1789, "Front Panel.PanelBounds"=w1790) -> ()  [unwired: 1 in, 2 out]
              }
              frame Enabled {
              }
            }
          }
        }
      }
      n1030 = local read "蜂鸣音效"() -> (w92:waveform(dbl)[])
      n1031 = while {
        tunnel: [w95] -> w84
        stop <- w95 stop-if-true
        # "等待启动配置"
        n1032 = local read "确认设置"() -> (w95:bool)
        n1033 = Wait (ms)(milliseconds to wait=u32 100 ("等待时间（毫秒）")) -> ()  [unwired: 1 out]
      }
      n1034 = while {
        tunnel: w92 -> [w148]
        tunnel: [w147] -> w91
        stop <- w152 stop-if-true
        # "报警音效"
        n1035 = case shown="\"一级报警\"" "报警状态" {
          tunnel: [w157 w165 w167] -> w150
          tunnel: [u32 500 ("等待时间（毫秒）") u32 500 ("等待时间（毫秒）") u32 0 ("等待时间（毫秒）")] -> w149
          frame "正常", "累积报警" {
            w161 = 0 ("y")
            w163 = 6  # 3s
            n1036 = feedback #9(w161) -> (w159:i32)
            n1037 = Greater Or Equal?(x=w159, y=w163) -> (x >= y?=w156:bool)
            n1038 = And(x="有掉线？", y=w156) -> (x .and. y?=w157:bool)
            n1039 = Select(t=w161, s=w156, f=w159) -> (s? t:f=w162:i32)
            n1040 = Increment(x=w162) -> (x+1=w160:i32)
            n1041 = feedback-in #9(w160) -> ()
          }
          frame "一级报警" {
            w165 = TRUE  # T
          }
          frame "二级报警" {
            w167 = TRUE  # T
          }
        }
        n1042 = case shown="真" w150 {
          tunnel: w148 -> [_ w154]
          tunnel: [_ w153] -> w147
          frame False {
          }
          frame True {
            n1043 = call "播放波形"("Data"=w154) -> ("error out"=w153:errorcluster)  [unwired: 18 in]
          }
        }
        n1044 = Wait (ms)(milliseconds to wait=w149) -> ()  [unwired: 1 out]
        n1045 = local read "停止"() -> (w152:bool)
      }
      n1046 = while {
        tunnel: w84 -> [_]
        stop <- w98 stop-if-true
        # "随时切换定时周期"
        n1047 = node-c288("周期", "周期", "累积剂量记录" ("源名称")) -> (w101:T10)  [unwired: 7 in]
        n1048 = timed-loop {
          timing: w101 -> [_]
          timing-out: [_] -> w100
          stop <- _ stop-if-true
          # "每小时，记录一次累积剂量到数据库"
          n1049 = node-c288() -> ()  [unwired: 1 in, 1 out]
          n1050 = local read "事件-累积剂量"() -> (w103:refnum<user-event>)
          n1051 = local read "累积剂量"() -> (w102:T2)
          n1052 = for {
            tunnel: w103 -> [w107]
            tunnel: w102 -> [w104] mode=indexing
            # "依次触发事件"
            n1053 = Unbundle By Name(w104) -> ("启用累积？"=w105:bool)
            n1054 = case shown="真" w105 {
              tunnel: w107 -> [_ w110]
              tunnel: w104 -> [_ w108]
              frame False {
                # "未启用则不记"
              }
              frame True {
                # "启用则记录"
                n1055 = Generate User Event(user event=w110, event data cluster=w108) -> (error out=w109:errorcluster)  [unwired: 2 in, 1 out]
                n1056 = call <vilib>:"Clear Errors.vi"("error in (no error)"=w109) -> ()  [unwired: 5 in, 2 out]
              }
            }
            n1057 = Wait (ms)(milliseconds to wait=u32 500 ("等待时间（毫秒）")) -> ()  [unwired: 1 out]
          }
          n1058 = node-c288() -> ()  [unwired: 1 in, 1 out]
        }
        n1059 = local read "停止"() -> (w98:bool)
        n1060 = node-c288(w100) -> ()  [unwired: 1 out]
      }
      n1061 = call <vilib>:"Clear Errors.vi"("error in (no error)"=w91) -> ()  [unwired: 5 in, 2 out]
      n1062 = Array Size(array="报警列表提示") -> (size(s)=w89:i32)
      n1063 = Array Size(array="设备列表提示") -> (size(s)=w88:i32)
      n1064 = Decrement(x=w89) -> (x-1=w86:i32)
      n1065 = Decrement(x=w88) -> (x-1=w85:i32)
      n1066 = while {
        stop <- w759 stop-if-true
        # "列表动态效果"
        n1067 = local read "暂停发送"() -> (w760:bool)
        n1068 = case shown="真" w760 {
          selector: w760 -> [_ w778]
          frame False {
            n1069 = local write "等待时间（毫秒）"(u32 1000 ("等待时间（毫秒）")) -> ()
            n1070 = case shown="真" "回复背景色锁" {
              selector: "回复背景色锁" -> [_ w773]
              frame False {
              }
              frame True {
                w771 = -2 ("Column")
                n1071 = Not(x=w773) -> (.not. x?=w772:bool)
                n1072 = local write "回复背景色锁"(w772) -> ()
                n1073 = Bundle("Column"=w771, "Column"=w771) -> (w768:cluster{"Column":i32, "Column":i32})  [unwired: 1 in]
                n1074 = property on="实时数据列表" class="MCListbox (严格)"("ActiveCell"=w768, "CellBG"=u32 16777226) -> (error out=w765:errorcluster)  [unwired: 2 in, 1 out]
                n1075 = Bundle("Column"=-1, "Column"=-2) -> (w766:cluster{"Column":i32, "Column":i32})  [unwired: 1 in]
                n1076 = property on="实时数据列表" class="MCListbox (严格)"(error in=w765, "ActiveCell"=w766, "CellBG"=u32 13816530) -> ()  [unwired: 1 in, 2 out]
              }
            }
          }
          frame True {
            w776 = -2 ("Column")
            w779 = u8 20 ("B动态范围")
            # "处于编辑模式的列表，背景色渐变"
            n1077 = local write "回复背景色锁"(w778) -> ()
            n1078 = feedback #10(0.0 ("y")) -> (w787:dbl)
            n1079 = Greater Or Equal?(x=w787, y=1.0) -> (x >= y?=w782:bool)
            n1080 = feedback #11(0.05 ("y")) -> (w785:dbl)
            n1081 = Add(x=w787, y=w785) -> (x+y=w790:dbl)
            n1082 = feedback-in #10(w790) -> ()
            n1083 = case shown="假" w782 {
              tunnel: [w799 -0.05 ("y")] -> w784
              tunnel: w787 -> [w802 _]
              tunnel: w785 -> [w800 _]
              frame False {
                n1084 = Less Or Equal?(x=w802, y=-1.0) -> (x <= y?=w798:bool)
                n1085 = case shown="真" w798 {
                  tunnel: w800 -> [w803 _]
                  tunnel: [w803 0.05 ("y")] -> w799
                  frame False {
                  }
                  frame True {
                    # "-1"
                    n1086 = Wait (ms)(milliseconds to wait=u32 0 ("等待时间（毫秒）")) -> ()  [unwired: 1 out]
                  }
                }
              }
              frame True {
                # "1"
                n1087 = Wait (ms)(milliseconds to wait=u32 0 ("等待时间（毫秒）")) -> ()  [unwired: 1 out]
              }
            }
            n1088 = Multiply(x=3.141592653589793, y=w790) -> (x*y=w792:dbl)
            n1089 = Cosine(x=w792) -> (cos(x)=w793:dbl)
            n1090 = Multiply(x=w793, y=w779) -> (x*y=w783:dbl)
            n1091 = Add(x=w783, y=w779) -> (x+y=w781:dbl)
            n1092 = Absolute Value(x=w781) -> (abs(x)=w794:dbl)
            n1093 = case shown="假" "T:G,F:B" {
              tunnel: w794 -> [w809 w813]
              tunnel: [w810 w812] -> w796
              tunnel: [w808 w811] -> w795
              frame False {
                w810 = u8 255 ("G")
                # "B"
                n1094 = Subtract(x=w810, y=w809) -> (x-y=w808:dbl)
              }
              frame True {
                w811 = u8 255 ("G")
                # "G"
                n1095 = Subtract(x=w811, y=w813) -> (x-y=w812:dbl)
              }
            }
            n1096 = feedback-in #11(w784) -> ()
            n1097 = Bundle("Column"=w776, "Column"=w776) -> (w774:cluster{"Column":i32, "Column":i32})  [unwired: 1 in]
            n1098 = call <vilib>:"RGB to Color.vi"("B"=w796, "G"=w795, "R"=u8 125 ("R常量")) -> ("Color"=w775:u32)
            n1099 = local write "等待时间（毫秒）"(u32 5 ("等待时间（毫秒）")) -> ()
            n1100 = property on="实时数据列表" class="多列列表框 (严格)"("ActiveCell"=w774, "CellBG"=w775) -> ()  [unwired: 2 in, 2 out]
          }
        }
        n1101 = Wait (ms)(milliseconds to wait="等待时间（毫秒）") -> ()  [unwired: 1 out]
        n1102 = local read "停止"() -> (w759:bool)
      }
      n1103 = while {
        tunnel: "报警列表提示" -> [w121]
        tunnel: "设备列表提示" -> [w122]
        tunnel: w86 -> [w124]
        tunnel: w85 -> [w123]
        stop <- w119 stop-if-true
        w127 = 0 ("y")
        w125 = 10  # 5s
        # "滚动提示切换"
        n1104 = feedback #12(w127) -> (w129:i32)
        n1105 = Greater Or Equal?(x=w129, y=w125) -> (x >= y?=w120:bool)
        n1106 = Wait (ms)(milliseconds to wait=u32 500 ("等待时间（毫秒）")) -> ()  [unwired: 1 out]
        n1107 = Select(t=w127, s=w120, f=w129) -> (s? t:f=w126:i32)
        n1108 = Increment(x=w126) -> (x+1=w128:i32)
        n1109 = feedback-in #12(w128) -> ()
        n1110 = case shown="真" w120 {
          tunnel: w124 -> [_ w143]
          tunnel: w123 -> [_ w140]
          tunnel: w122 -> [_ w135]
          tunnel: w121 -> [_ w134]
          frame False {
            # "未到 5s"
          }
          frame True {
            w131 = 0 ("y")
            w146 = 0 ("y")
            # "5s 到了"
            n1111 = feedback #13(w146) -> (w145:i32)
            n1112 = feedback #14(w131) -> (w141:i32)
            n1113 = Greater?(x=w145, y=w143) -> (0:w144:bool)
            n1114 = Greater?(x=w141, y=w140) -> (0:w142:bool)
            n1115 = Select(t=w146, s=w144, f=w145) -> (s? t:f=w139:i32)
            n1116 = Select(t=w131, s=w142, f=w141) -> (s? t:f=w136:i32)
            n1117 = Increment(x=w139) -> (x+1=w138:i32)
            n1118 = feedback-in #13(w138) -> ()
            n1119 = Increment(x=w136) -> (x+1=w137:i32)
            n1120 = feedback-in #14(w137) -> ()
            n1121 = Index Array(array=w134, index=w139) -> (element=→"报警列表操作提示":string)
            n1122 = Index Array(array=w135, index=w136) -> (element=→"设备列表操作提示":string)
          }
        }
        n1123 = local read "停止"() -> (w119:bool)
      }
    }
  }
